vi "Text control 2 v6.0_pump-specific.vi"() -> ()   [LabVIEW 2016]
panel:
  in  "Tab Control":enum32{"Main", "Other parameters"}(tab)
  out "Line running":i32
  out "Total lines":i32
  out "Path":path=path "C:/users/rlp38/09Apr2009LTtesting/test2.txt"
  out "I vs Vg":cluster{"Y data in":dbl[], "X data in":dbl[]}[](graph)
  out "Is max":dbl format="%.2e"
  out "Id max":dbl format="%.2e"
  out "Ig max":dbl format="%.2e"
  out "Imax vs time":cluster{"Y data in":dbl[], "X data in":dbl[]}[](graph)
  out "Imin vs time":cluster{"Y data in":dbl[], "X data in":dbl[]}[](graph)
  out "I vs Vd":cluster{"Y data in":dbl[], "X data in":dbl[]}[](graph)
  in  "Script":string="#-------------------------------------------------------\n# SPM pump cleaning script\n#\n# Version 0.5\n# Author: Dimitrios Simatos\n# Last updated: 2018-01-05\n#-------------------------------------------------------\n# Description\n#\n# This script is designed to run the cleaning sequence of the SPM OEM pump.\n# This script needs to be run 4 times!\n#-------------------------------------------------------\n# Changes\n#\n# Placed initialization and hard stop commands in the beginning.\n#-------------------------------------------------------\n# Important points\n#\n# Never leave any liquid in the pump to dry after the experiments. If they dry, the residue may block the valve.\n# Always run the cleaning cycle after the experiments.\n# Use clockwise rotation when going up in valve port numbers and vice versa.\n#-------------------------------------------------------\n# Things to do before running the script\n#\n# Set time units to minutes.\n# Set filenames.\n# Replace the tubing, if necessary.\n#-------------------------------------------------------\n# Port connections\n#\n# Port 1: Waste\n# Port 2: Waste\n# Port 3: Various cleaning liquids\n# Port 4: Waste\n# Port 5: Waste\n# Port 6: Waste\n#\n# Between each of the 4 runs, the settings of Port 3 will change, according to the cleaning protocol.\n# The settings for Port 3 are:\n# 1st run: 1% v/v solution of sodium hypochlorite in ultrapure water\n# 2nd run: 0.1% w/v solution of sodium dodecyl sulfate in ultrapure water\n# 3rd run: Ultrapure water\n# 4th run: Waste (in air, not immersed in liquid)\n#-------------------------------------------------------\n# Cleaning protocol for the SPM OEM pump (from the manual)\n#\n# A cleaning procedure should be performed at the end of each day or in between two different experiments.\n# An effective cleaning can be performed in the following manner:\n# • Bleach solution to kill microorganisms\n# 1. Prepare a solution of 1% chlorine bleach and deionized water\n#    NOTE: Prepare a 1% v/v solution of sodium hypochlorite in deionized water\n# 2. Prepare a reservoir and place 1 tubing in the bleach solution and 5 tubings in a waste recipient\n# 3. Pick up the bleach solution through 1 port to entirely fill the syringe\n# 4. Sequentially output the syringe content through the remaining ports and throw it to the waste\n# 5. Repeat operation at least 2 times\n# • Detergent solution to remove debris\n# 1. Prepare a solution of 0.1% detergent and deionized water\n#    NOTE: Prepare a 0.1% w/v solution of sodium dodecyl sulfate in deionized water\n# 2. Move the tubing from the bleach solution reservoir and place it into a reservoir of detergent solution\n# 3. Pick up the detergent solution through 1 port to entirely fill the syringe\n# 4. Sequentially output the detergent solution through the remaining ports into the waste recipient\n# 5. Repeat operation at least 2 times\n# • Rinsing water to prepare the pump for your next experiment\n# 1. Move the tubing from the detergent solution reservoir and place it into a reservoir of deionized water\n# 2. Pick up the rinsing solution through 1 port to entirely fill the syringe\n# 3. Sequentially output the rinse water through the remaining ports into the waste recipient\n# 4. Repeat operation at least 2 times\n# • Replace the tubing, if necessary\n#-------------------------------------------------------\n# Pumping cycles and execution time\n#\n# Execution time for a single cycle: 6 x (1 min + 10 sec) = 7 minutes\n# Total execution time: 4 x 7 = 28 minutes\n# Since the script has to run 4 times, the cleaning lasts for: 4 x 28 = 112 minutes\n# Air must be the last to be pumped through the valve, to remove all liquids.\n# There are 4 pumping cycles. Each one draws a different liquid through port 3 and pumps it sequentially through ports 1,2,4,5,6.\n# During the sequential pumping, each port receives 200 ml of liquid (20% of the total syringe volume = 600 \"plunger units\")\n# The device must be disconnected from the port during the cleaning procedure.\n# All cycles are similar, except cycle 1 has the initialization command uncommented and the first report valve command commented.\n#-------------------------------------------------------\n# Volume of liquid needed\n#\n# Volume of liquid needed per cycle: 1 ml\n# Total volume of liquid needed per script run: 4 x 1 = 4 ml\n# Since the script has to run 4 times, the first 3 with different liquids, I need:\n# 4 ml of 1% v/v solution of sodium hypochlorite in ultrapure water\n# 4 ml of 0.1% w/v solution of sodium dodecyl sulfate in ultrapure water\n# 4 ml of ultrapure water\n#-------------------------------------------------------\n# Parameters\n#\n# Syringe size: 1 ml\n# Step resolution N = 0.01 mm\n# Drawing flow V = 300 pulses/second (6000 ul/min)\n# Pumping flow V = 300 pulses/second (6000 ul/min)\n#-------------------------------------------------------\n# Pump initialization\npump /1T #hard stop pump\npump /1ZR #initialize pump\n#-------------------------------------------------------\n# Cycle 1\n# Fill the syringe\npump /1Q #query pump\npump /1? #report absolute plunger position\n#pump /1?6 #report valve position\nwait-min 1 #wait 1 minute\npump /1N0R #set step resolution: 0.01 mm\npump /1Q #query pump\npump /1? #report absolute plunger position (the plunger should be at 0)\npump /1?6 #report valve position\nwait 1000 #wait 1 second\npump /1V300R #choose speed: 300 steps/s (6000 ul/min)\npump /1Q #query pump\nwait 1000 #wait 1 second\npump /1I3R #go to port 3, clockwise rotation\npump /1Q #query pump\npump /1?6 #report valve position\nwait 1000 #wait 1 second\npump /1A3000R #go to absolute position 3000 (= draw 1 ml)\nwait 30000 #wait 30 seconds\npump /1Q #query pump\npump /1? #report absolute plunger position (the plunger should have finished moving)\n#pump /1?6 #report valve position\n# The sequential pumping begins\n# Port 1\npump /1O1R #switch to port 1, counterclockwise rotation\npump /1Q #query pump\npump /1?6 #report valve position\npump /1A2400R #go to absolute position 2400 (= pump 200 ul)\npump /1Q #query pump\npump /1? #report absolute plunger position (the plunger should be moving to 0)\nwait-min 1 #wait 1 minute\npump /1? #report absolute plunger position (the plunger should have finished moving)\n# Port 2\npump /1I2R #switch to port 2, clockwise rotation\npump /1Q #query pump\npump /1?6 #report valve position\npump /1A1800R #go to absolute position 1800 (= pump 200 ul)\npump /1Q #query pump\npump /1? #report absolute plunger position (the plunger should be moving to 0)\nwait-min 1 #wait 1 minute\npump /1? #report absolute plunger position (the plunger should have finished moving)\n# Port 4\npump /1I4R #switch to port 4, clockwise rotation\npump /1Q #query pump\npump /1?6 #report valve position\npump /1A1200R #go to absolute position 1200 (= pump 200 ul)\npump /1Q #query pump\npump /1? #report absolute plunger position (the plunger should be moving to 0)\nwait-min 1 #wait 1 minute\npump /1? #report absolute plunger position (the plunger should have finished moving)\n# Port 5\npump /1I5R #switch to port 5, clockwise rotation\npump /1Q #query pump\npump /1?6 #report valve position\npump /1A600R #go to absolute position 600 (= pump 200 ul)\npump /1Q #query pump\npump /1? #report absolute plunger position (the plunger should be moving to 0)\nwait-min 1 #wait 1 minute\npump /1? #report absolute plunger position (the plunger should have finished moving)\n# Port 6\npump /1I6R #switch to port 6, clockwise rotation\npump /1Q #query pump\npump /1?6 #report valve position\npump /1A0R #go to absolute position 0 (= pump 200 ul)\npump /1Q #query pump\npump /1? #report absolute plunger position (the plunger should be moving to 0)\nwait-min 1 #wait 1 minute\npump /1? #report absolute plunger position (the plunger should have finished moving)\n#-------------------------------------------------------\n# Cycle 2\n# Fill the syringe\n#pump /1ZR #initialize pump\npump /1Q #query pump\npump /1? #report absolute plunger position\npump /1?6 #report valve position\nwait-min 1 #wait 1 minute\npump /1N0R #set step resolution: 0.01 mm\npump /1Q #query pump\npump /1? #report absolute plunger position (the plunger should be at 0)\npump /1?6 #report valve position\nwait 1000 #wait 1 second\npump /1V300R #choose speed: 300 steps/s (6000 ul/min)\npump /1Q #query pump\nwait 1000 #wait 1 second\npump /1O3R #go to port 3, counterclockwise rotation\npump /1Q #query pump\npump /1?6 #report valve position\nwait 1000 #wait 1 second\npump /1A3000R #go to absolute position 3000 (= draw 1 ml)\nwait 30000 #wait 30 seconds\npump /1Q #query pump\npump /1? #report absolute plunger position (the plunger should have finished moving)\n#pump /1?6 #report valve position\n# The sequential pumping begins\n# Port 1\npump /1O1R #switch to port 1, counterclockwise rotation\npump /1Q #query pump\npump /1?6 #report valve position\npump /1A2400R #go to absolute position 2400 (= pump 200 ul)\npump /1Q #query pump\npump /1? #report absolute plunger position (the plunger should be moving to 0)\nwait-min 1 #wait 1 minute\npump /1? #report absolute plunger position (the plunger should have finished moving)\n# Port 2\npump /1I2R #switch to port 2, clockwise rotation\npump /1Q #query pump\npump /1?6 #report valve position\npump /1A1800R #go to absolute position 1800 (= pump 200 ul)\npump /1Q #query pump\npump /1? #report absolute plunger position (the plunger should be moving to 0)\nwait-min 1 #wait 1 minute\npump /1? #report absolute plunger position (the plunger should have finished moving)\n# Port 4\npump /1I4R #switch to port 4, clockwise rotation\npump /1Q #query pump\npump /1?6 #report valve position\npump /1A1200R #go to absolute position 1200 (= pump 200 ul)\npump /1Q #query pump\npump /1? #report absolute plunger position (the plunger should be moving to 0)\nwait-min 1 #wait 1 minute\npump /1? #report absolute plunger position (the plunger should have finished moving)\n# Port 5\npump /1I5R #switch to port 5, clockwise rotation\npump /1Q #query pump\npump /1?6 #report valve position\npump /1A600R #go to absolute position 600 (= pump 200 ul)\npump /1Q #query pump\npump /1? #report absolute plunger position (the plunger should be moving to 0)\nwait-min 1 #wait 1 minute\npump /1? #report absolute plunger position (the plunger should have finished moving)\n# Port 6\npump /1I6R #switch to port 6, clockwise rotation\npump /1Q #query pump\npump /1?6 #report valve position\npump /1A0R #go to absolute position 0 (= pump 200 ul)\npump /1Q #query pump\npump /1? #report absolute plunger position (the plunger should be moving to 0)\nwait-min 1 #wait 1 minute\npump /1? #report absolute plunger position (the plunger should have finished moving)\n#-------------------------------------------------------\n# Cycle 3\n# Fill the syringe\n#pump /1ZR #initialize pump\npump /1Q #query pump\npump /1? #report absolute plunger position\npump /1?6 #report valve position\nwait-min 1 #wait 1 minute\npump /1N0R #set step resolution: 0.01 mm\npump /1Q #query pump\npump /1? #report absolute plunger position (the plunger should be at 0)\npump /1?6 #report valve position\nwait 1000 #wait 1 second\npump /1V300R #choose speed: 300 steps/s (6000 ul/min)\npump /1Q #query pump\nwait 1000 #wait 1 second\npump /1O3R #go to port 3, counterclockwise rotation\npump /1Q #query pump\npump /1?6 #report valve position\nwait 1000 #wait 1 second\npump /1A3000R #go to absolute position 3000 (= draw 1 ml)\nwait 30000 #wait 30 seconds\npump /1Q #query pump\npump /1? #report absolute plunger position (the plunger should have finished moving)\n#pump /1?6 #report valve position\n# The sequential pumping begins\n# Port 1\npump /1O1R #switch to port 1, counterclockwise rotation\npump /1Q #query pump\npump /1?6 #report valve position\npump /1A2400R #go to absolute position 2400 (= pump 200 ul)\npump /1Q #query pump\npump /1? #report absolute plunger position (the plunger should be moving to 0)\nwait-min 1 #wait 1 minute\npump /1? #report absolute plunger position (the plunger should have finished moving)\n# Port 2\npump /1I2R #switch to port 2, clockwise rotation\npump /1Q #query pump\npump /1?6 #report valve position\npump /1A1800R #go to absolute position 1800 (= pump 200 ul)\npump /1Q #query pump\npump /1? #report absolute plunger position (the plunger should be moving to 0)\nwait-min 1 #wait 1 minute\npump /1? #report absolute plunger position (the plunger should have finished moving)\n# Port 4\npump /1I4R #switch to port 4, clockwise rotation\npump /1Q #query pump\npump /1?6 #report valve position\npump /1A1200R #go to absolute position 1200 (= pump 200 ul)\npump /1Q #query pump\npump /1? #report absolute plunger position (the plunger should be moving to 0)\nwait-min 1 #wait 1 minute\npump /1? #report absolute plunger position (the plunger should have finished moving)\n# Port 5\npump /1I5R #switch to port 5, clockwise rotation\npump /1Q #query pump\npump /1?6 #report valve position\npump /1A600R #go to absolute position 600 (= pump 200 ul)\npump /1Q #query pump\npump /1? #report absolute plunger position (the plunger should be moving to 0)\nwait-min 1 #wait 1 minute\npump /1? #report absolute plunger position (the plunger should have finished moving)\n# Port 6\npump /1I6R #switch to port 6, clockwise rotation\npump /1Q #query pump\npump /1?6 #report valve position\npump /1A0R #go to absolute position 0 (= pump 200 ul)\npump /1Q #query pump\npump /1? #report absolute plunger position (the plunger should be moving to 0)\nwait-min 1 #wait 1 minute\npump /1? #report absolute plunger position (the plunger should have finished moving)\n#-------------------------------------------------------\n# Cycle 4\n# Fill the syringe\n#pump /1ZR #initialize pump\npump /1Q #query pump\npump /1? #report absolute plunger position\npump /1?6 #report valve position\nwait-min 1 #wait 1 minute\npump /1N0R #set step resolution: 0.01 mm\npump /1Q #query pump\npump /1? #report absolute plunger position (the plunger should be at 0)\npump /1?6 #report valve position\nwait 1000 #wait 1 second\npump /1V300R #choose speed: 300 steps/s (6000 ul/min)\npump /1Q #query pump\nwait 1000 #wait 1 second\npump /1O3R #go to port 3, counterclockwise rotation\npump /1Q #query pump\npump /1?6 #report valve position\nwait 1000 #wait 1 second\npump /1A3000R #go to absolute position 3000 (= draw 1 ml)\nwait 30000 #wait 30 seconds\npump /1Q #query pump\npump /1? #report absolute plunger position (the plunger should have finished moving)\n#pump /1?6 #report valve position\n# The sequential pumping begins\n# Port 1\npump /1O1R #switch to port 1, counterclockwise rotation\npump /1Q #query pump\npump /1?6 #report valve position\npump /1A2400R #go to absolute position 2400 (= pump 200 ul)\npump /1Q #query pump\npump /1? #report absolute plunger position (the plunger should be moving to 0)\nwait-min 1 #wait 1 minute\npump /1? #report absolute plunger position (the plunger should have finished moving)\n# Port 2\npump /1I2R #switch to port 2, clockwise rotation\npump /1Q #query pump\npump /1?6 #report valve position\npump /1A1800R #go to absolute position 1800 (= pump 200 ul)\npump /1Q #query pump\npump /1? #report absolute plunger position (the plunger should be moving to 0)\nwait-min 1 #wait 1 minute\npump /1? #report absolute plunger position (the plunger should have finished moving)\n# Port 4\npump /1I4R #switch to port 4, clockwise rotation\npump /1Q #query pump\npump /1?6 #report valve position\npump /1A1200R #go to absolute position 1200 (= pump 200 ul)\npump /1Q #query pump\npump /1? #report absolute plunger position (the plunger should be moving to 0)\nwait-min 1 #wait 1 minute\npump /1? #report absolute plunger position (the plunger should have finished moving)\n# Port 5\npump /1I5R #switch to port 5, clockwise rotation\npump /1Q #query pump\npump /1?6 #report valve position\npump /1A600R #go to absolute position 600 (= pump 200 ul)\npump /1Q #query pump\npump /1? #report absolute plunger position (the plunger should be moving to 0)\nwait-min 1 #wait 1 minute\npump /1? #report absolute plunger position (the plunger should have finished moving)\n# Port 6\npump /1I6R #switch to port 6, clockwise rotation\npump /1Q #query pump\npump /1?6 #report valve position\npump /1A0R #go to absolute position 0 (= pump 200 ul)\npump /1Q #query pump\npump /1? #report absolute plunger position (the plunger should be moving to 0)\nwait-min 1 #wait 1 minute\npump /1? #report absolute plunger position (the plunger should have finished moving)\n#-------------------------------------------------------"
  out "Command running:":string
  out "Serial port data":string
  out "Elapsed Time":dbl caption="Elapsed Time (s)"
  in  "Units (label only)":u16(ring)=1 items=["Seconds", "Minutes", "Hours"]
  in  "Time Offset":dbl caption="Set Start Time (s)"
  in  "Reset":bool
  in  "Auto Reset":bool
  in  "integration time":u32(slide) max=2 step=1 scale=0.0..2.0
  in  "Interrupt run":bool
  out "Absolute plunger position vs time":cluster{"Y data in":dbl[], "X data in":dbl[]}[](graph)
  out "Valve position vs time":cluster{"Y data in":dbl[], "X data in":dbl[]}[](graph)
  out "Is on":dbl format="%.2e"
  out "Id on":dbl format="%.2e"
  out "Ig on":dbl format="%.2e"
  out "Ion vs time":cluster{"Y data in":dbl[], "X data in":dbl[]}[](graph)
  out "Ioff vs time":cluster{"Y data in":dbl[], "X data in":dbl[]}[](graph)
  out "Ig min":dbl format="%.2e"
  out "Id min":dbl format="%.2e"
  out "Is min":dbl format="%.2e"
  out "Is off":dbl format="%.2e"
  out "Id off":dbl format="%.2e"
  out "Ig off":dbl format="%.2e"
  in  "Integration time (long)":dbl=0.32 min=0.04 max=2.0 step=0.02 format="%.2f"
  in  "Integration time (short)":dbl=0.0019 min=8e-05 max=0.0019 step=8e-05 format="%^.0e"
  in  "Gate: Compliance":dbl=0.001 format="%.8f"
  in  "Drain: Compliance":dbl=0.001 format="%.8f"
  in  "Hard stop pump":bool
  in  "Halt pump":bool
  in  "Gate Range\nmode":u16(ring) items=["Auto", "Limited", "Fixed"]
  in  "Gate Range":u8(slide)=6 max=11 scale=0.0..11.0
  in  "Source/Drain\nRange mode":u16(ring) items=["Auto", "Limited", "Fixed"]
  in  "Source/Drain Range":u8(slide)=6 max=11 scale=0.0..11.0
  in  "Panel Controls":T1={"Emergency Stop"=refnum, "TransGraph Max"=1e-05, "Text/Graph (text=false)"=TRUE} {"TransGraph Max" format="%.2e"}
  in  "Panel Controls 2":T2={"Emergency Stop"=refnum, "TransGraph Max"=1e-05, "Text/Graph (text=false)"=TRUE, "TransGraph Min"=1e-11} {"TransGraph Min" format="%.2e"; "TransGraph Max" format="%.2e"}
  in  "SMU4":cluster{"on/off":bool, "Voltage":dbl} {"Voltage" min=-100.0 max=100.0 format="%.2f"}
  in  "Full Reset":bool
  in  "Standby":T3
  out "error out":errorcluster
  in  "Delay before read (ms)":u32=1000
  in  "byte count":u32=64
  in  "Serial End Mode for Reads":u16(ring)=2 items=["None", "LastBit", "TermChar"]
  in  "Timeout (ms)":u32=10000
  in  "Enable Termination\nChar (T)":bool=TRUE
  in  "Termination char\n(0xA = '\\n' = LF)\n(0xD = '\\r' = CR)":u8=13 format="%.0x"
  in  "flow control":u16(ring) items=["None"=0, "XON/XOFF"=1, "RTS/CTS"=2, "DTR/DSR"=4]
  in  "stop bits":u16(ring)=10 items=["1.0"=10, "1.5"=15, "2.0"=20]
  in  "parity":u16(ring) items=["None", "Odd", "Even", "Mark", "Space"]
  in  "data bits":u16=8 min=5 max=8 step=1
  in  "VISA resource name":refnum<visa-resource-name>="COM6"
  in  "baud rate":u32=9600
  in  "Filename (variable part)":string="step_1_up-H2O_initial_"
  in  "Suffix (script)":string="step_1_up-H2O_initial_script.txt"
  out "Timings Indicator":T4
  in  "Timings (overwritten by the Front Panel)":T5={"integration time"=0, "Short/Long integration time"=0.00064, "hold time (sec)"=0.0, "delay time (sec)"=0.0, "Step Time (0 disables)"=0.0, "sweep method"=0, "Pulse period"=0.005, "Base voltage"=0.0, "Pulse width"=0.0005} {"Pulse width" min=0.0005 max=0.1 step=0.0001 format="%.4f"; "Base voltage" format="%^.4e"; "Pulse period" min=0.005 max=1.0 step=0.0001 format="%.4f"; "sweep method" items=["Continuous", "Pulsed"]; "Step Time (0 disables)" format="%.2f"; "delay time (sec)" format="%.4f"; "hold time (sec)" format="%.4f"; "Short/Long integration time" format="%^.0e"; "integration time" scale=0.0..2.0}
  in  "Gate":T6={"Gate Start"=0.0, "Gate Stop"=2.0, "Gate Step (linear only)"=1.0, "Gate Compliance"=0.0001, "Gate PComp"=0.0, "Range mode"=0, "Range"=6} {"Range" max=11 scale=0.0..11.0; "Range mode" items=["Auto", "Limited", "Fixed"]; "Gate PComp" format="%^.2e"; "Gate Compliance" format="%^.2e"; "Gate Step (linear only)" format="%^.4e"; "Gate Stop" format="%^.4e"; "Gate Start" format="%^.4e"}
  in  "Drain 2":T7={"Drain Start"=0.0, "Drain Stop"=2.0, "Drain Compliance"=0.0001, "Drain Step"=1.0, "Drain PComp"=0.0, "Range mode"=0, "Range"=6} {"Range" max=11 scale=0.0..11.0; "Range mode" items=["Auto", "Limited", "Fixed"]; "Drain PComp" format="%^.2e"; "Drain Step" format="%^.4e"; "Drain Compliance" format="%^.2e"; "Drain Stop" format="%^.4e"; "Drain Start" format="%^.4e"}
  # "Syntax:\nitime [s|m|l] time(sec): [s|m|l] determines the integration time setting (small|medium|long) and time sets the value.\nNOTE: The value of the integration time has to be within the range allowed by its category (s|m|l), otherwise, the closest value will be used. (e.g. if the category is set to short but the time value is very long, the actual value used will be the maximum short integration time.\nIntegration times:\n    Short: Default: 640 us. Range: 8E-5 - 1.92E-3 seconds.\n    Medium: Fixed at 1 NPL cycle (0.02 seconds).\n    Long: Default: 16 NPL cycles (0.32 seconds). Range: 2-100 NPL cycles (0.04 seconds - 2 seconds).\ngaterangemode [a|l|f]\ndrainrangemode [a|l|f]\npulsed [on|off] PulsePeriod(sec) PulseBaseVoltage PulseONWidth(sec)\nstandby [on l off]\nwait NumMilliseconds\nwait-min NumMinutes\n# texthere = comment\ntransfer [s|d] VgStart VgStop VgStep VdStart VdStop VdStep\noutput [s|d] VgStart VgStop VgStep VdStart VdStop VdStep\nsample Vg Vd NumSamples Time(s) SampleInterval(s)\nsamplei Idg NumSamples Time(s) SampleInterval(s) VDGcompliance\n100 samples is approximately 13 seconds with medium integration\n# if in doubt use SampleInterval(s) = 0.004\nstressV VG VD IGcompliance IDcompliance Duration(sec)\nstressI IDG VDGcompliance Duration(sec)\nvsu2pulse Bias Duration(s)\npulsedstressV [s|d] VEstop VgON VgOFF Period(s) PulseONwidth(s) Vd\nsample-fpp Vg Vd NumSamples Time\nresample-fpp Vg Vd\ntransfer-fpp [s|d] VgStart VgStop VgStep VdStart VdStop VdStep\noutput-fpp [s|d] VgStart VgStop VgStep VdStart VdStop VdStep\nserial SerialPortCommand\npump SerialPortCommand for the SPM pump\n\nSPM Pump Syntax (<x>: pump number, use 1 if only one pump):\nif the command syntax contains [R], then append the letter R to the command\n/<x>Q: query (a query command should follow each command)\n/<x>Z[R] or /<x>Y[R]: initialize pump\n/<x>N<n>[R] (<n>=0,1): <0> (<1>) microstep 0.01 mm (0.00125 mm) resolution\n/<x>I<n> (<n>=0-6): turn to port number n (clockwise)\n/<x>O<n> (<n>=0-6): turn to port number n (counterclockwise)\n/<x>X: Re-execute last command string\n/<x>G<n>[R] (<n>=0-60000): repeat command sequence (default: 0, 0=loop forever)\n/<x>g: Mark the start of a repeat sequence (max = 10)\n/<x>M<n>[R] (<n>=0-86400000): delay command execution by n milliseconds\n/<x>H: Halt; Pause the sequence after finishing the current move\n/<x>T: Hardstop; Interrupt the current move and suppress it from the sequence\n/<x>A<n>[R] (<n>=0-3000 with N=0, 0-24000 with N=1): absolute position\n/<x>P<n>[R] (<n>=0-3000 with N=0, 0-24000 with N=1): relative pickup\n/<x>D<n>[R] (<n>=0-3000 with N=0, 0-24000 with N=1): relative dispense\n/<x>V<n>[R] (<n>=1-1600 default: 150): set peak speed (pulses/sec)\nNOTE: The lowest speed limit is 1 pulse/sec, not 5, as the manual states.\n/<x>S<n>[R] (<n>=10-40 default: 22): set speed (NOT in pulses/sec, look in manual)\nNOTE: When controlled with absolute position, one does not need to pay special attention to the syringe that is mounted on the pump.\nWithdraw from lower stage (ports 3, 5), dispense from higher stage (ports 2, 4, 6).\nConnect Port 1 to waste."
  # "Time"
  # "1\n2\n3\n4\n5\n6\n7\n8\n9\n10\n11\n12\n13\n14\n15\n16\n17\n18\n19\n20"
  # "Serial port settings"
  # "Filename settings"
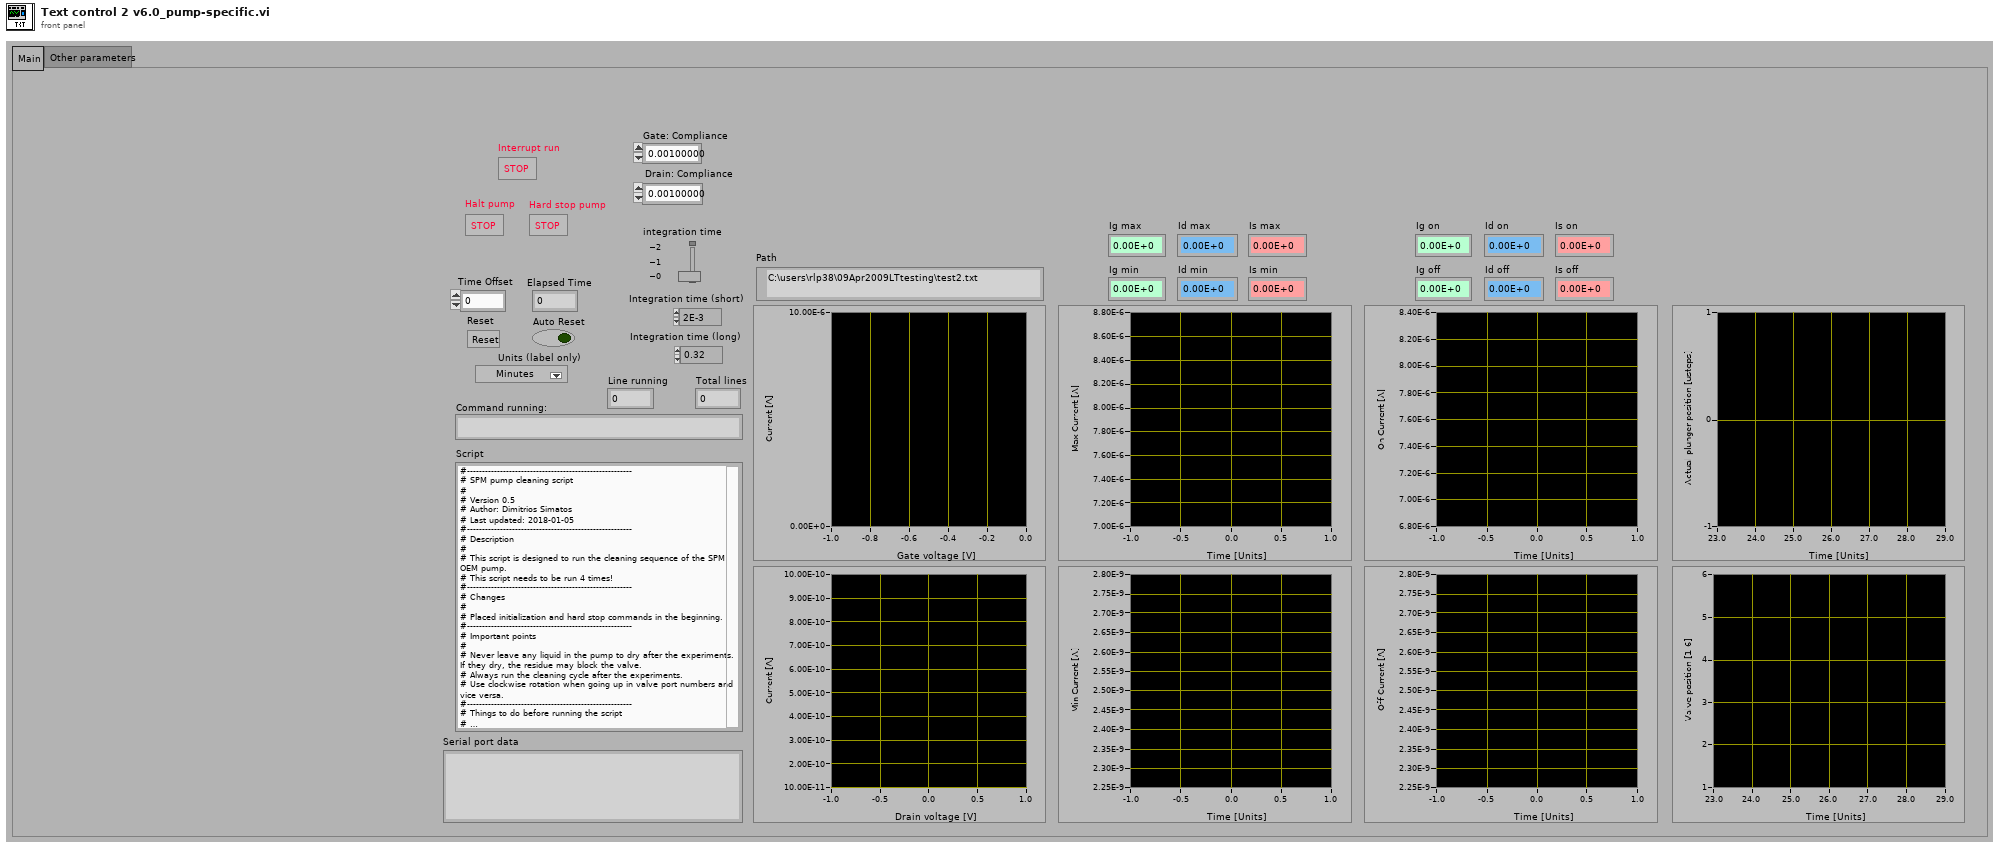
[diagram p1: front panel]
types:
  T1 = cluster{"Emergency Stop":refnum<vi>, "TransGraph Max":dbl, "Text/Graph (text=false)":bool}
  T2 = cluster{"Emergency Stop":refnum<vi>, "TransGraph Max":dbl, "Text/Graph (text=false)":bool, "TransGraph Min":dbl}
  T3 = cluster{"Gate Standby":bool, "Drain Standby":bool}
  T4 = cluster{"integration time (0:s, 1:m, 2:l)":u32, "Short/Long integration time":dbl, "hold time (sec)":dbl, "delay time (sec)":dbl, "Step Time (0 disables)":dbl, "sweep method":u16, "Pulse period":dbl, "Base voltage":dbl, "Pulse width":dbl}
  T5 = cluster{"integration time":u32, "Short/Long integration time":dbl, "hold time (sec)":dbl, "delay time (sec)":dbl, "Step Time (0 disables)":dbl, "sweep method":u16, "Pulse period":dbl, "Base voltage":dbl, "Pulse width":dbl}
  T6 = cluster{"Gate Start":dbl, "Gate Stop":dbl, "Gate Step (linear only)":dbl, "Gate Compliance":dbl, "Gate PComp":dbl, "Range mode":u16, "Range":u8}
  T7 = cluster{"Drain Start":dbl, "Drain Stop":dbl, "Drain Compliance":dbl, "Drain Step":dbl, "Drain PComp":dbl, "Range mode":u16, "Range":u8}
  T8 = enum16{"open", "replace", "create", "open or create", "replace or create", "replace or create with confirmation"}
  T9 = cluster{"V2 Start":dbl, "V2 Step":dbl, "Number of points":i32}
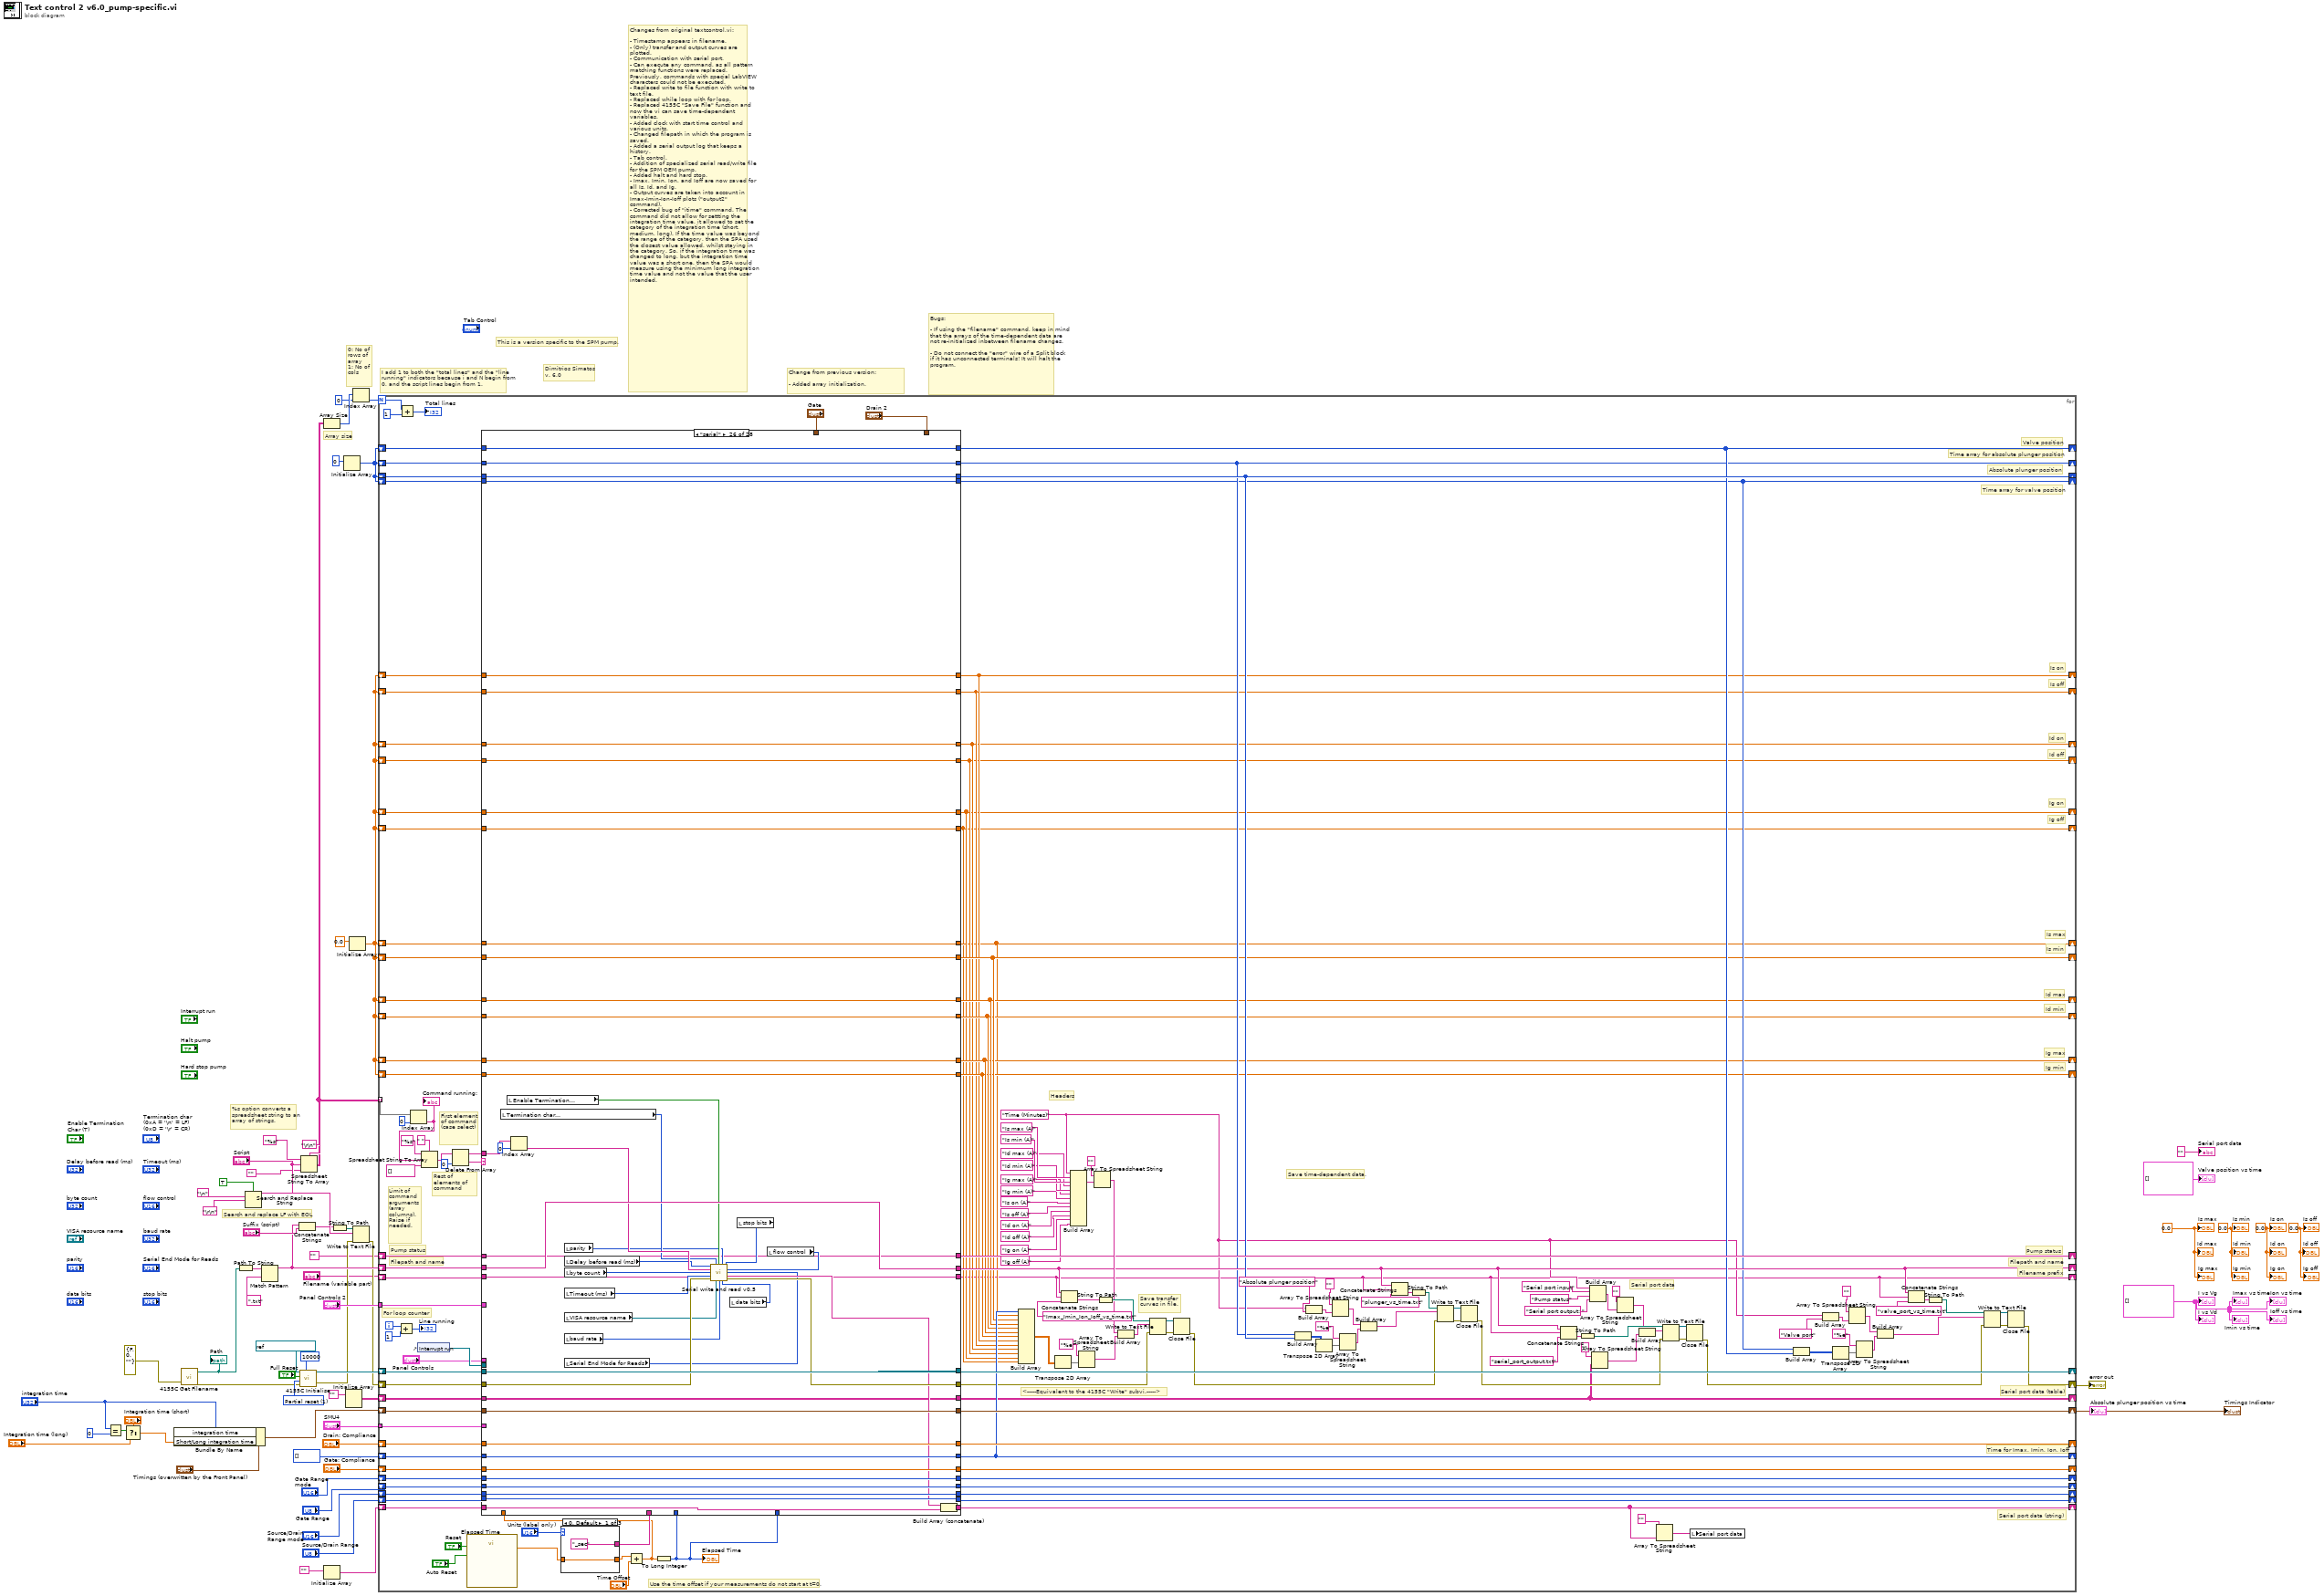
[diagram p0: block diagram]
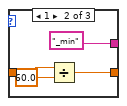
[diagram p2: hidden frame]
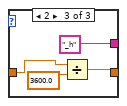
[diagram p3: hidden frame]
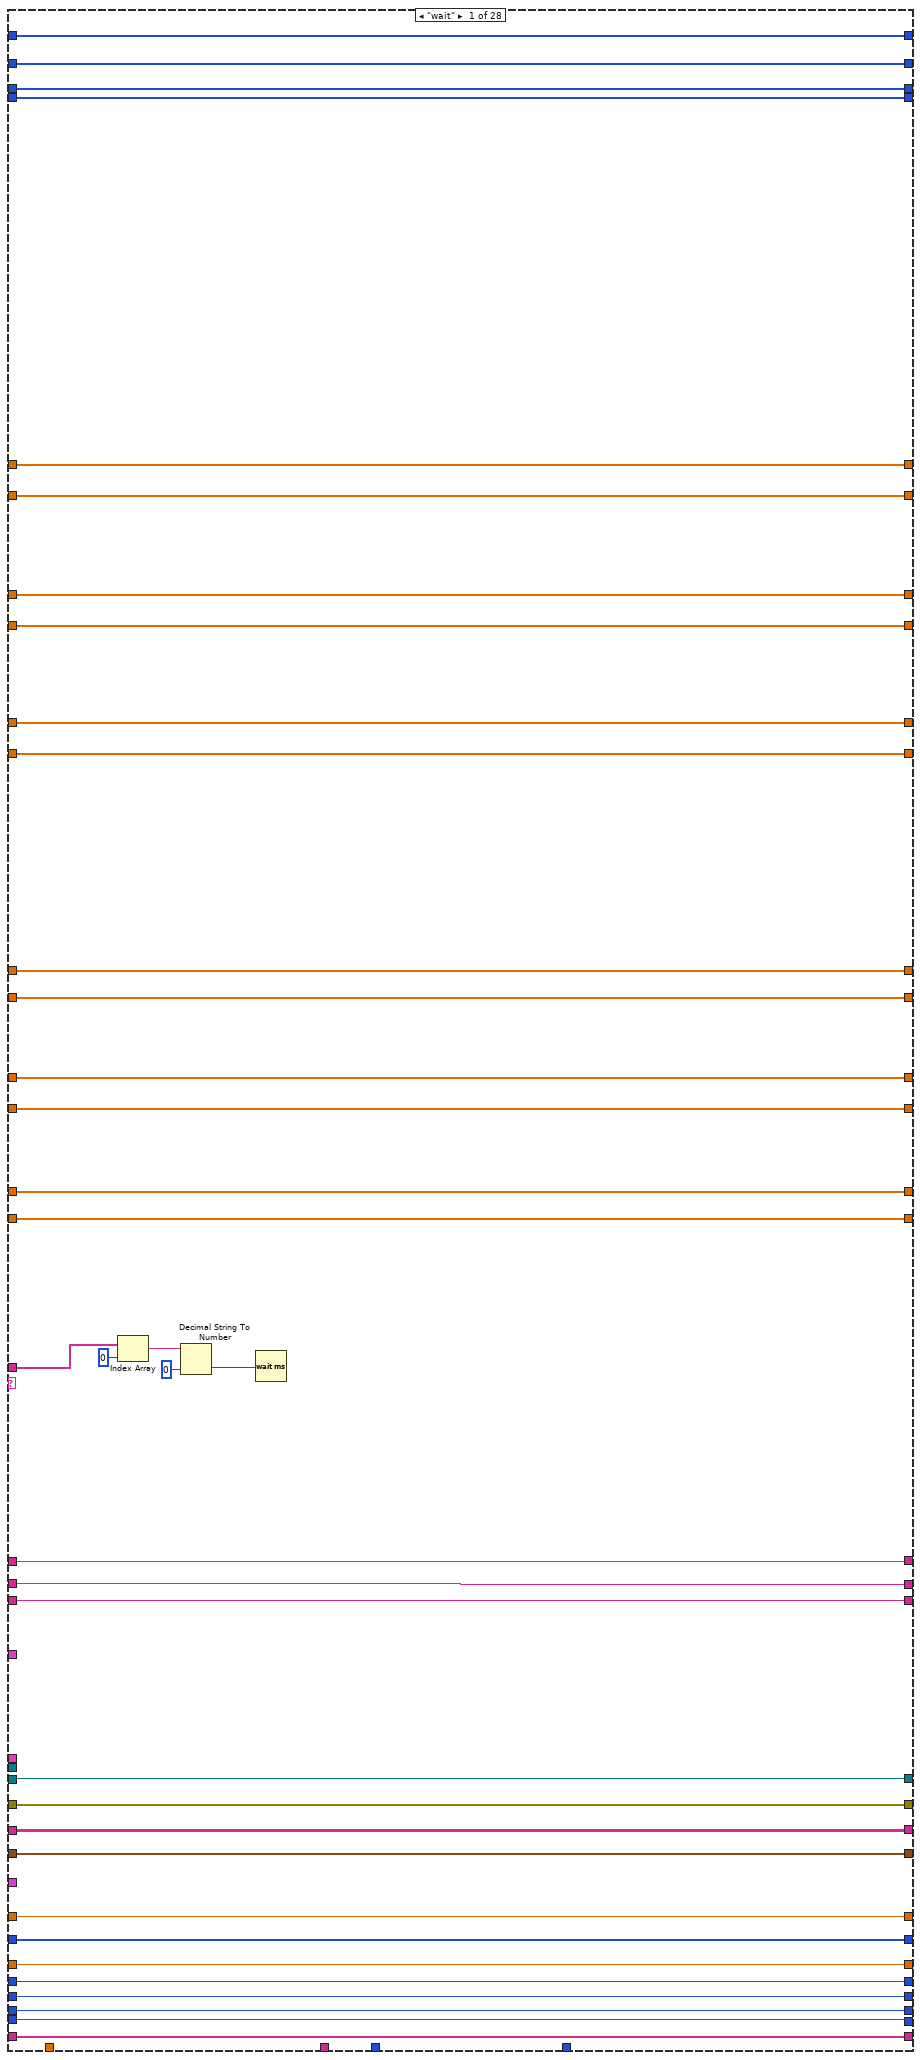
[diagram p4: hidden frame]
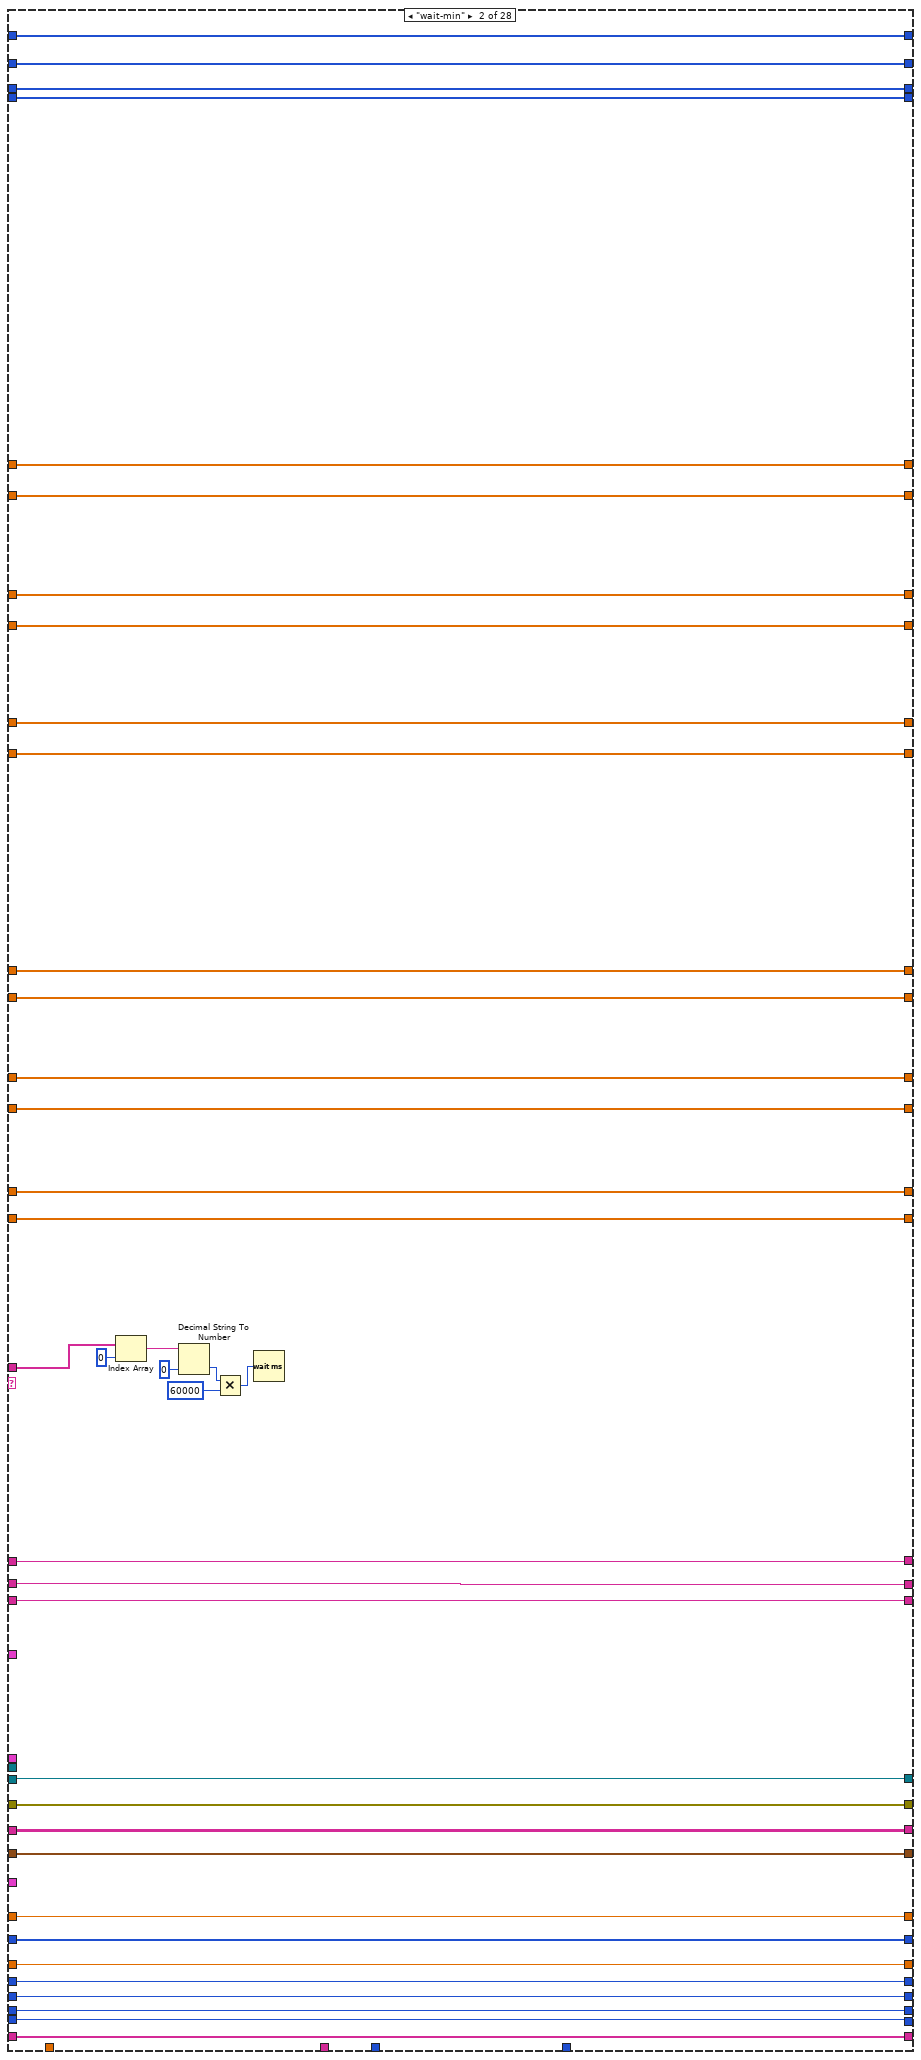
[diagram p5: hidden frame]
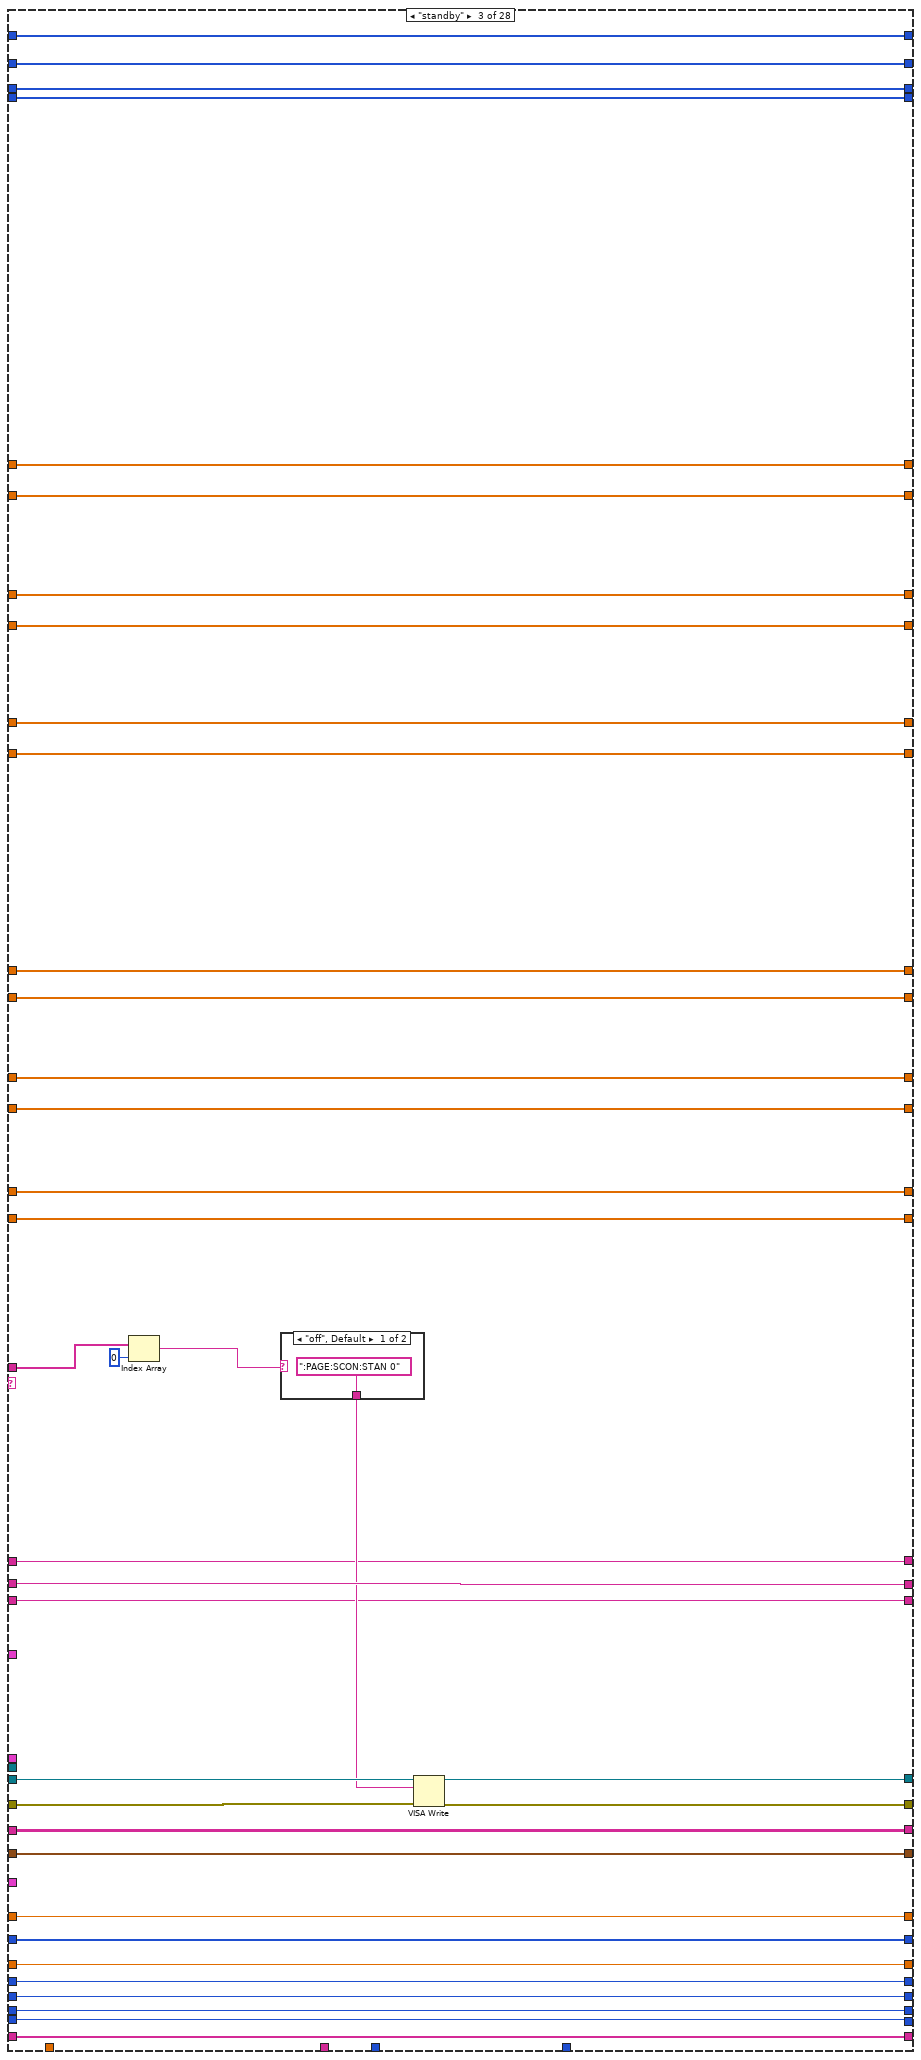
[diagram p6: hidden frame]
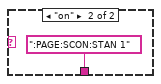
[diagram p7: hidden frame]
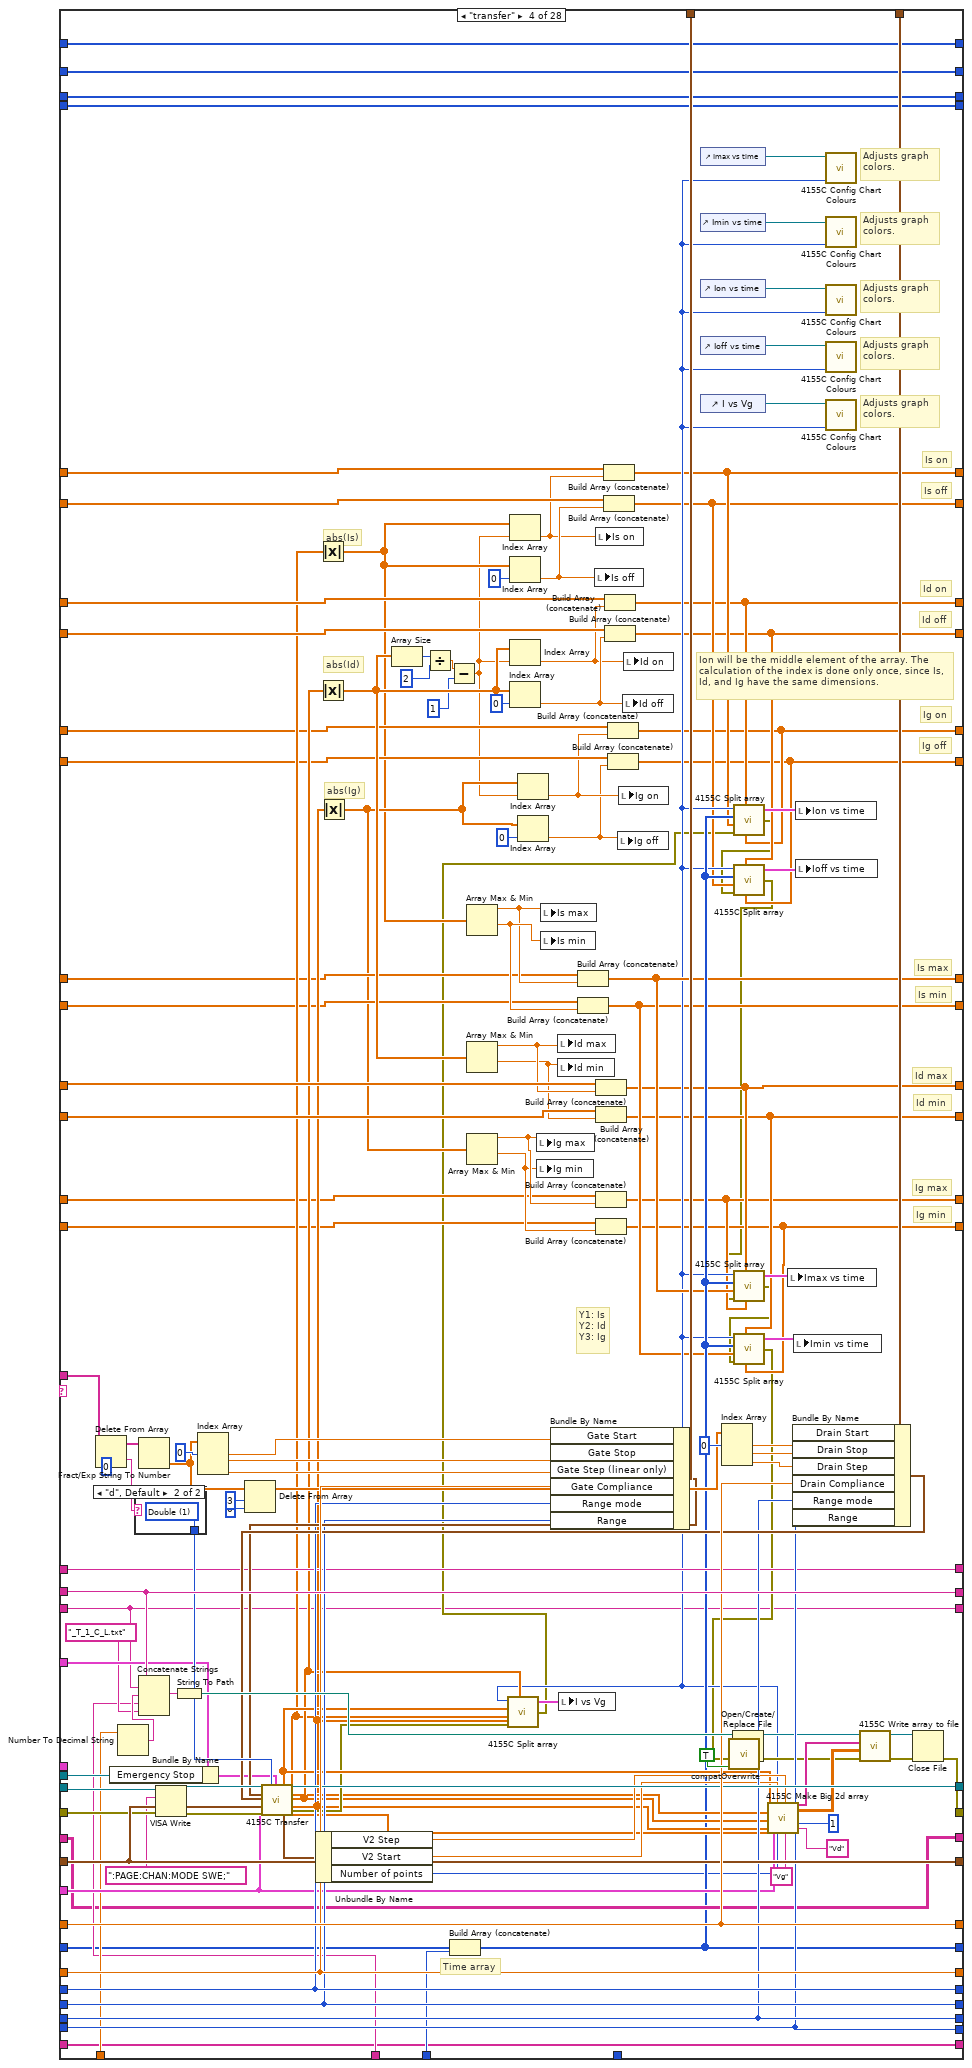
[diagram p8: hidden frame]
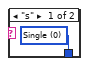
[diagram p9: hidden frame]
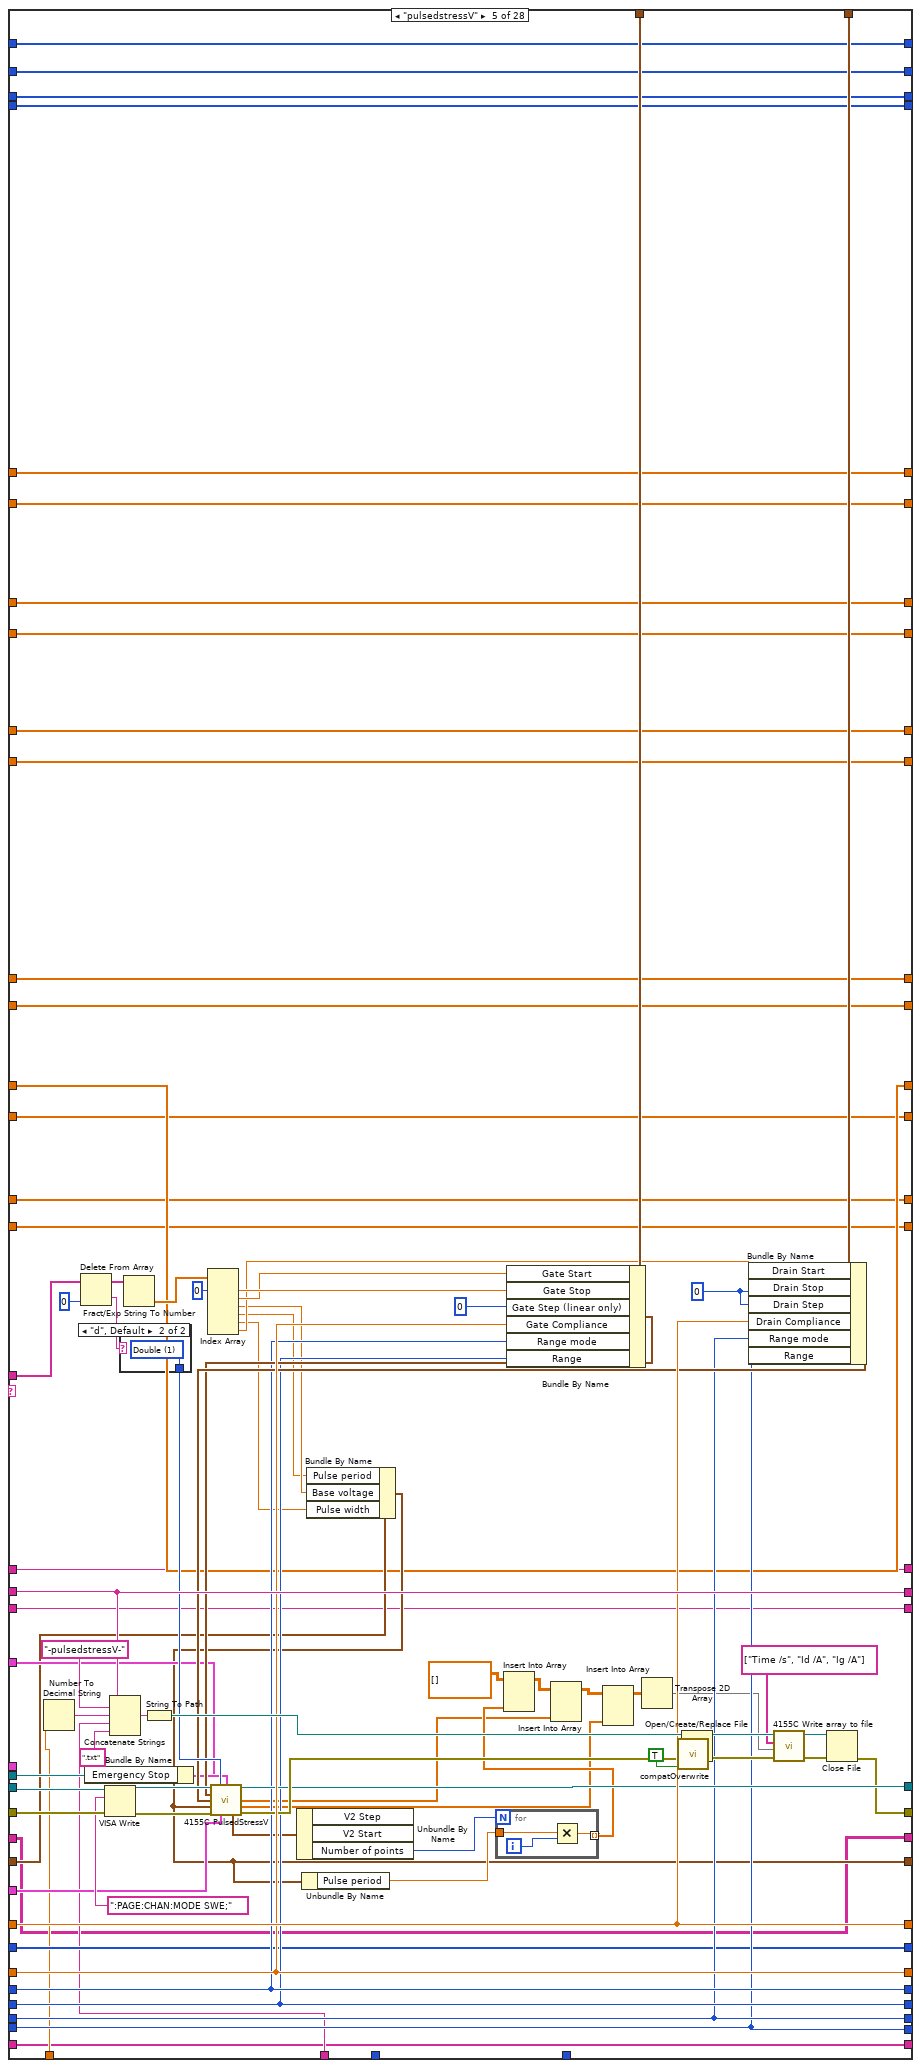
[diagram p10: hidden frame]
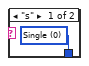
[diagram p11: hidden frame]
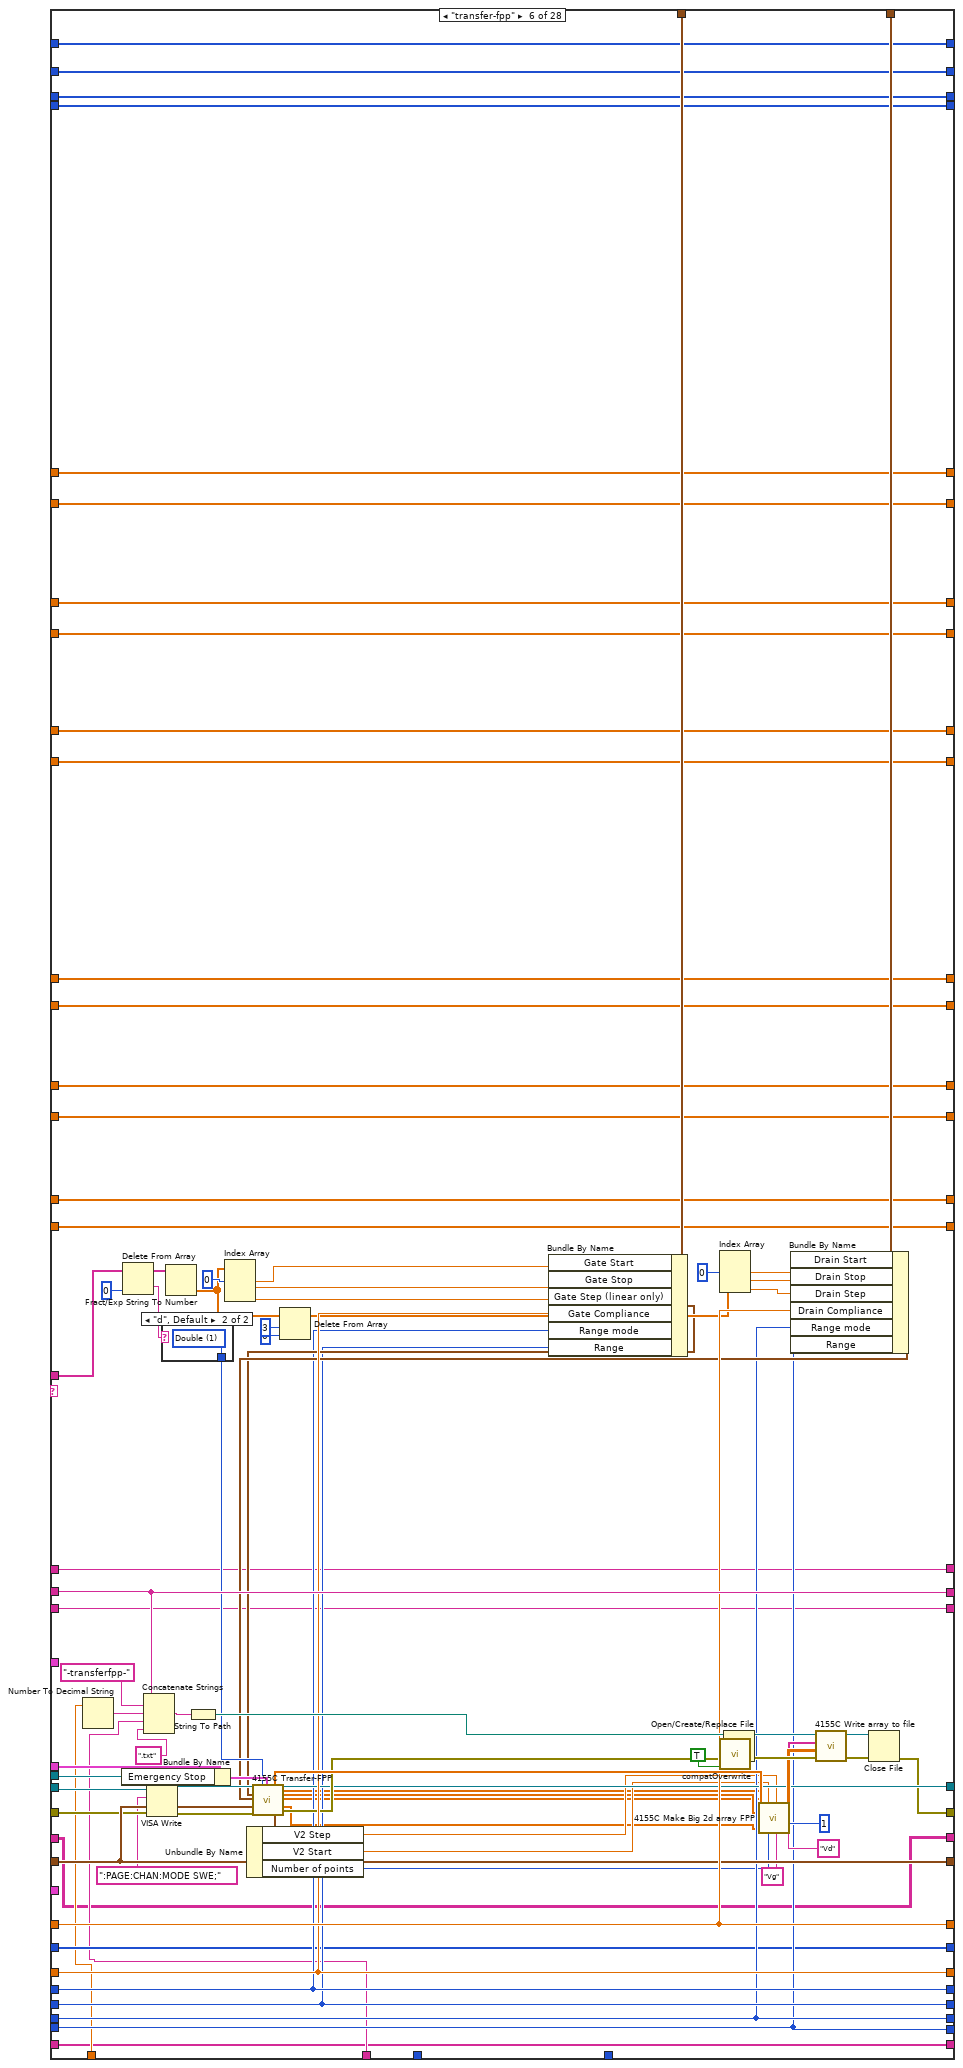
[diagram p12: hidden frame]
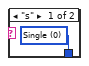
[diagram p13: hidden frame]
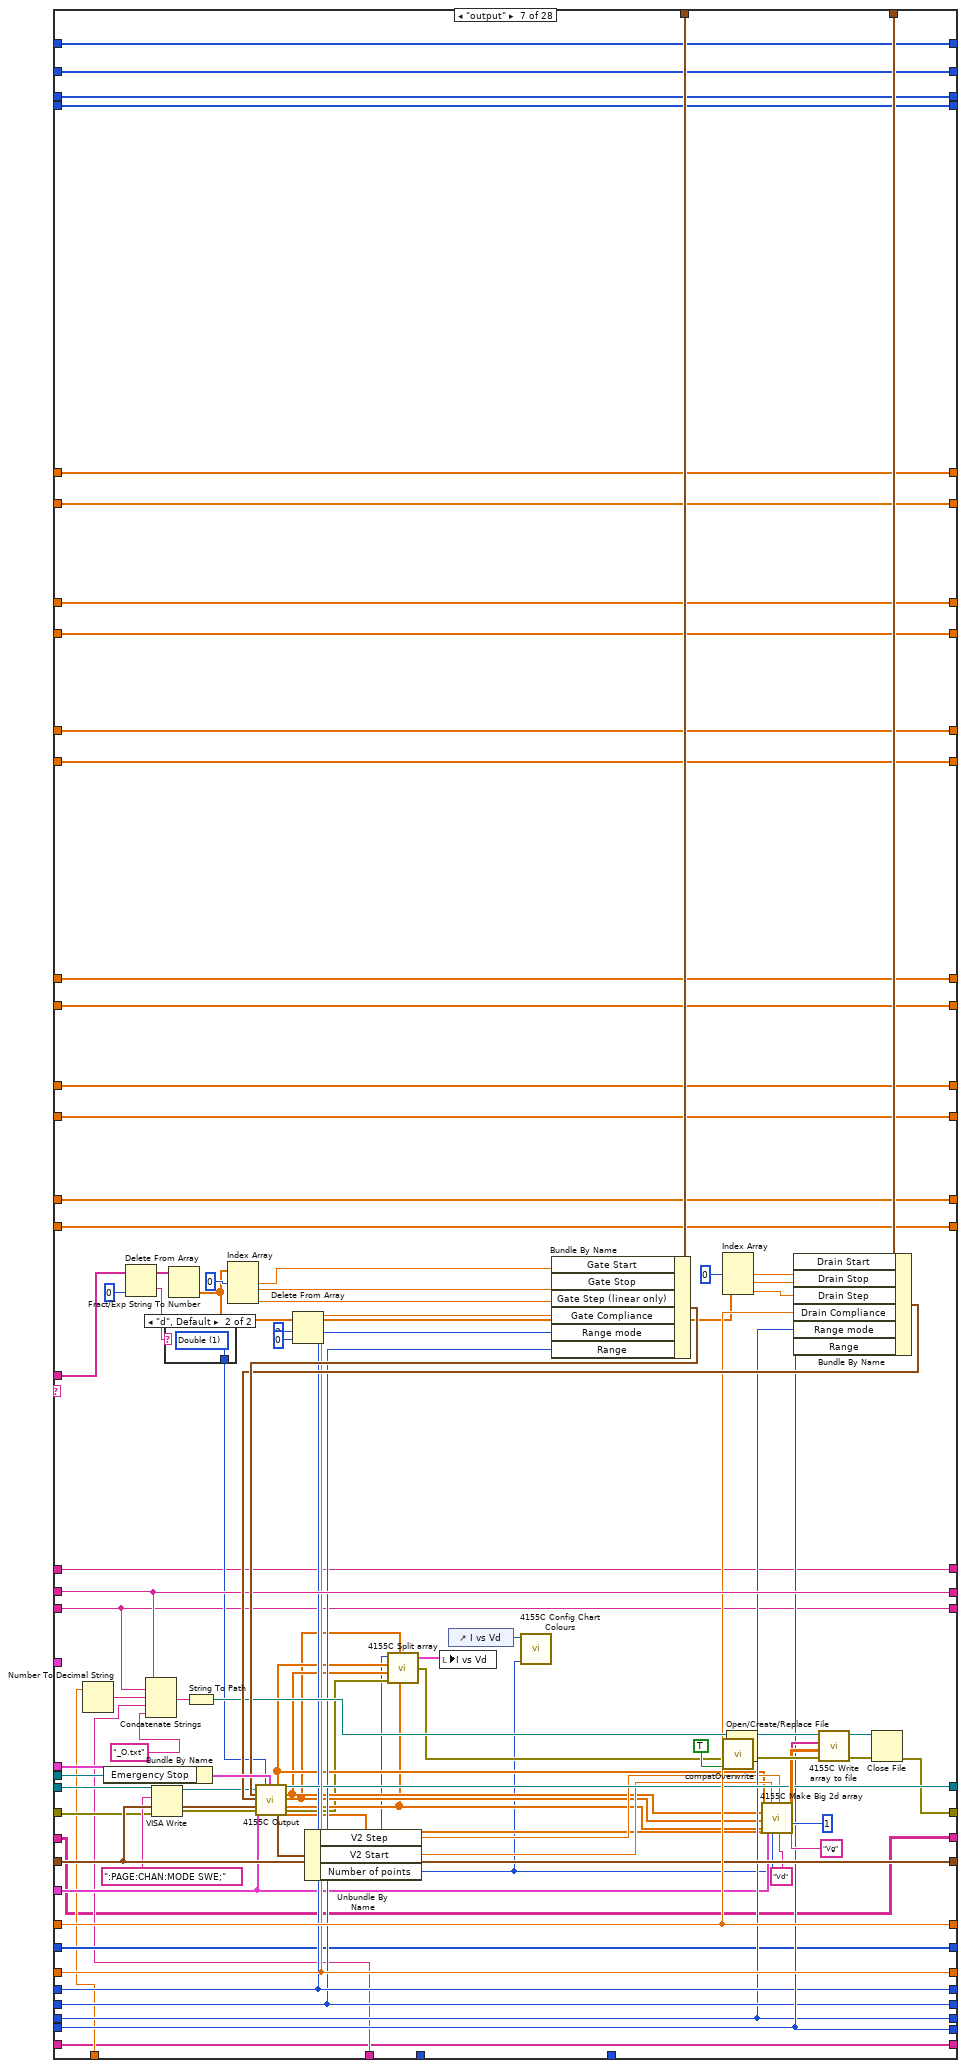
[diagram p14: hidden frame]
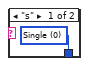
[diagram p15: hidden frame]
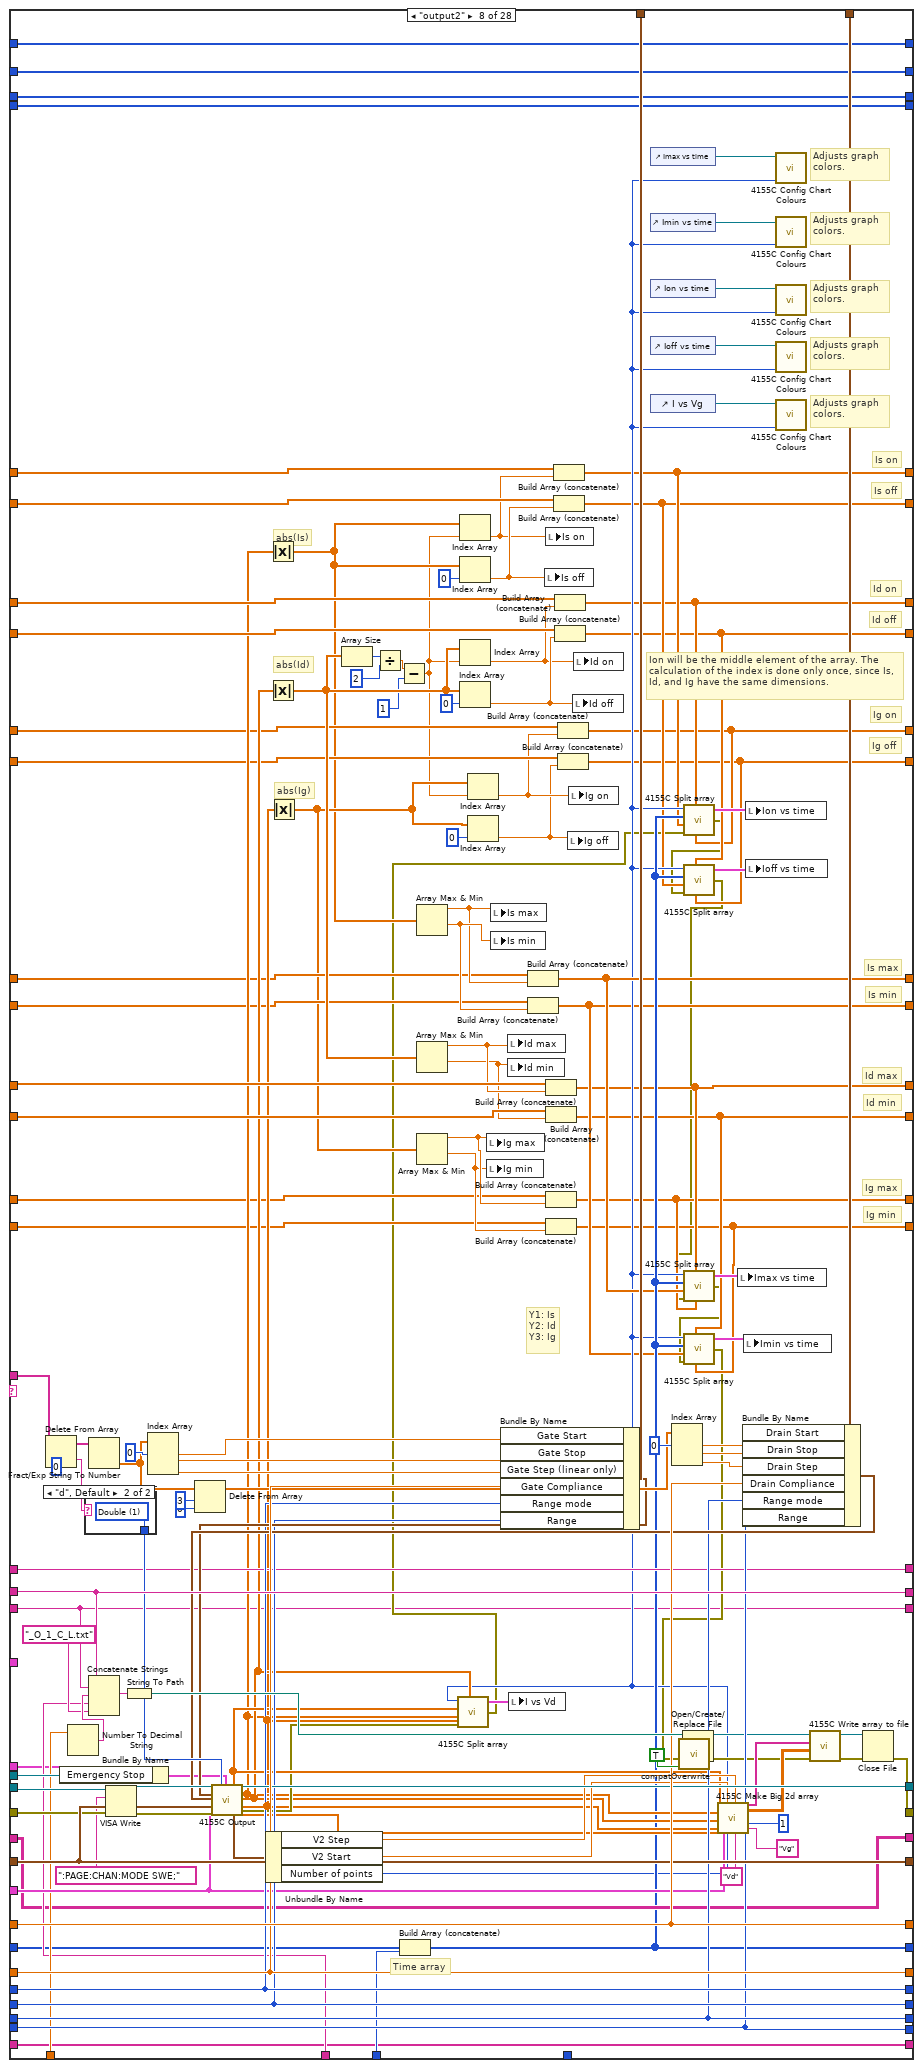
[diagram p16: hidden frame]
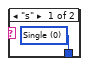
[diagram p17: hidden frame]
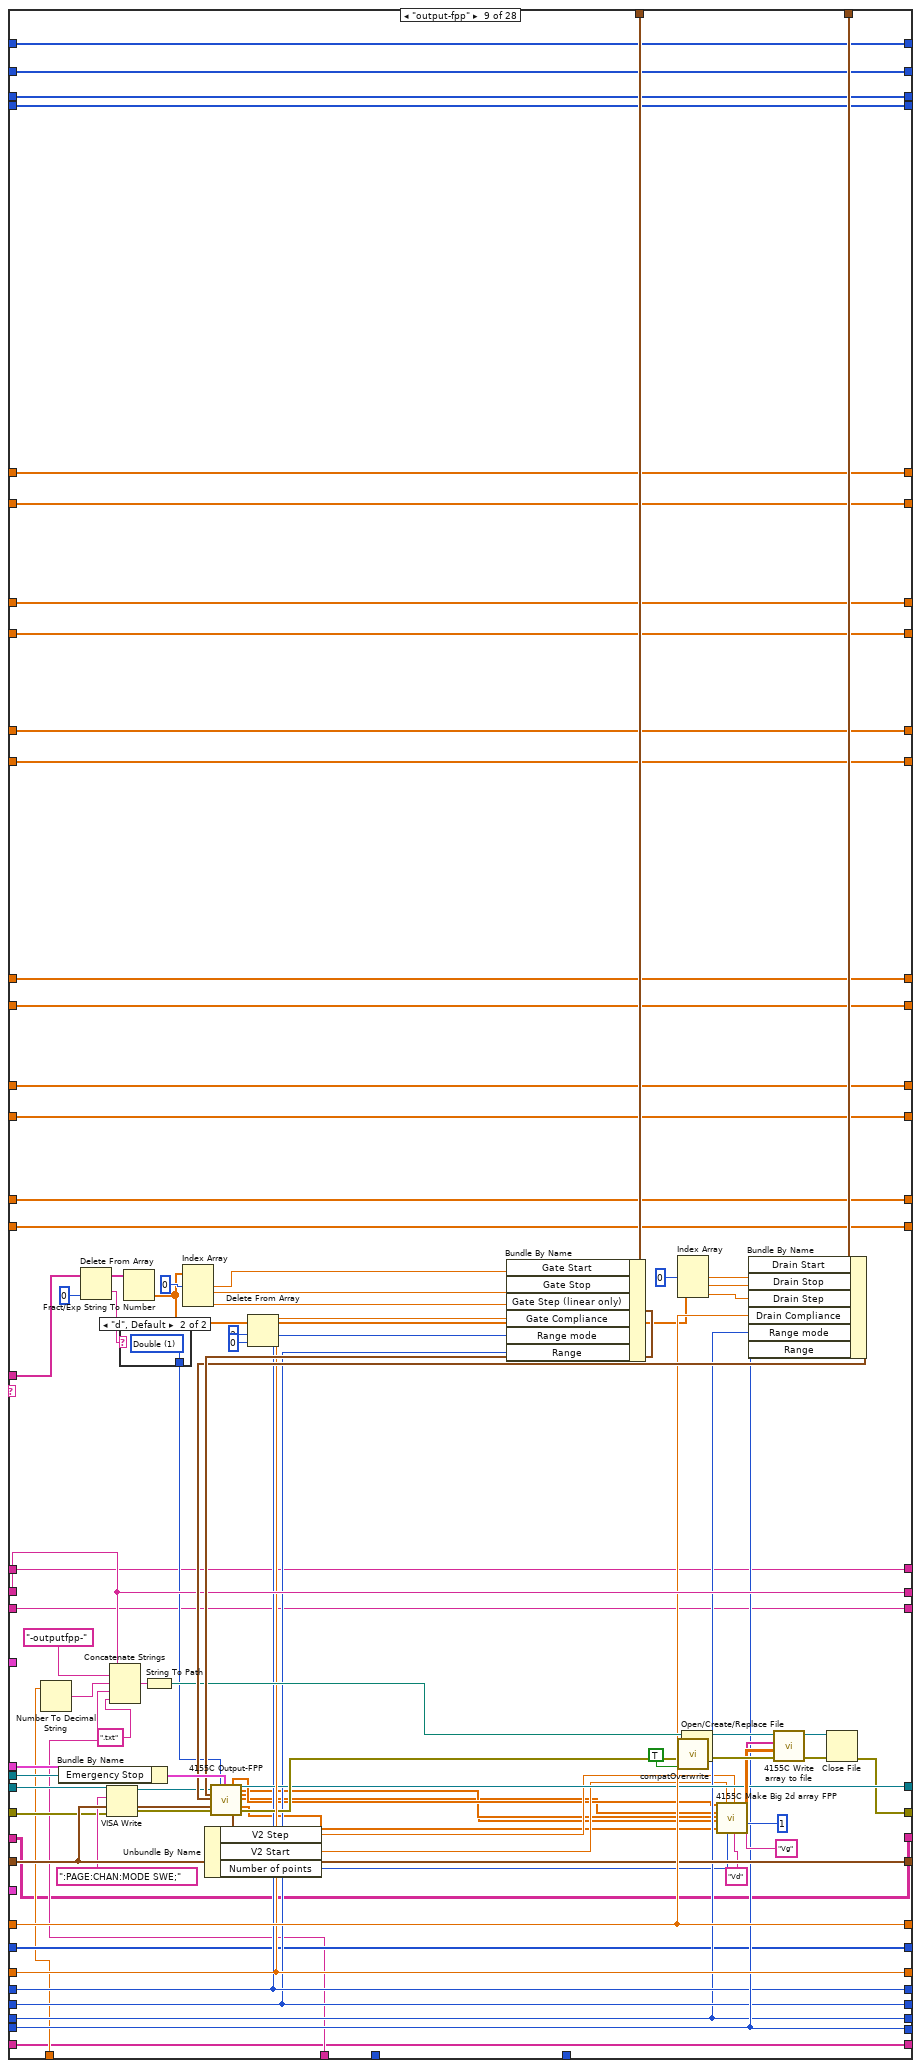
[diagram p18: hidden frame]
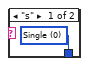
[diagram p19: hidden frame]
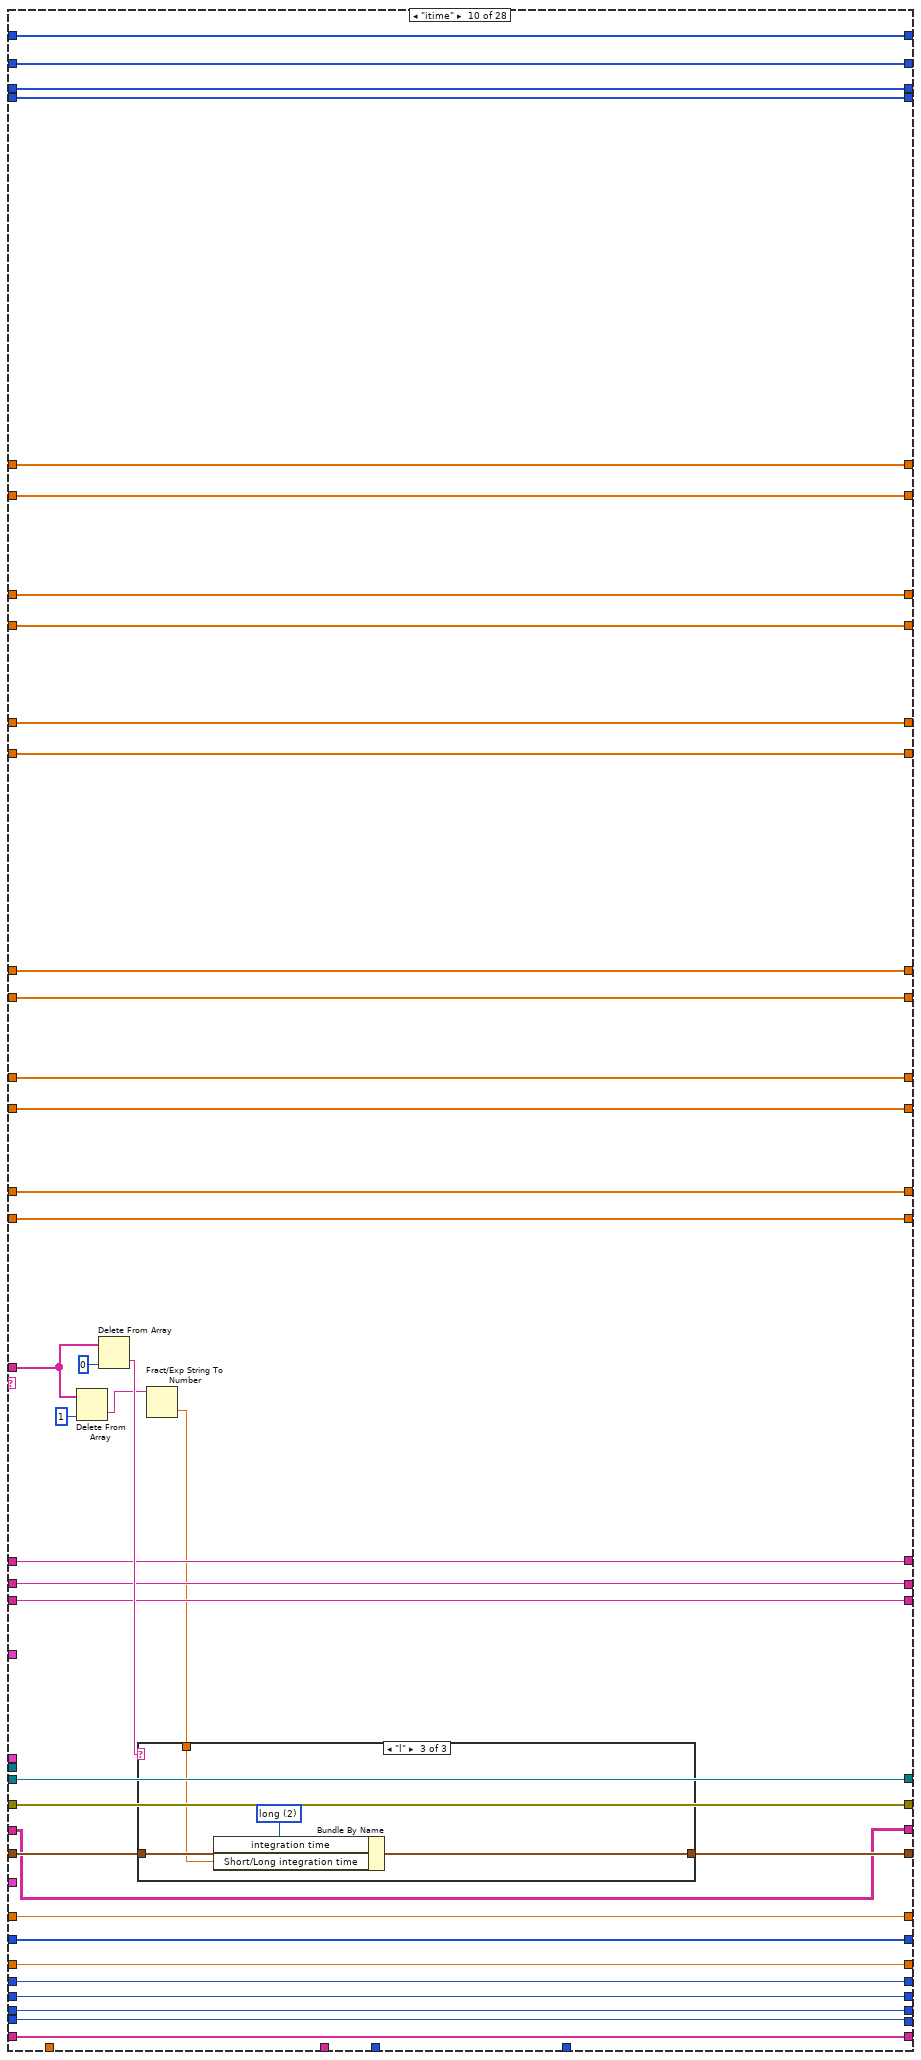
[diagram p20: hidden frame]
diagram:
  w4 = cluster{"Y data in":dbl[], "X data in":dbl[]}[] [] ("I vs Vg")
  w5 = 0.0 ("Is off")
  w6 = 0.0 ("Is on")
  w7 = 0.0 ("Is min")
  w8 = 0.0 ("Is max")
  w59 = u16 1 items=["Reset All", "Partial reset"] ("Type of reset")
  # "Change from previous version:\n\n- Added array initialization."
  # "This is a version specific to the SPM pump."
  # "I add 1 to both the \"total lines\" and the \"line running\" indicators because i and N begin from 0, and the script lines begin from 1."
  # "Bugs:\n\n- If using the \"filename\" command, keep in mind that the arrays of the time-dependent data are not re-initialized inbetween filename changes. \n\n- Do not connect the \"error\" wire of a Split block if it has unconnected terminals! It will halt the program."
  # "Array size"
  # "%s option converts a spreadsheet string to an array of strings."
  # "0: No of rows of array\n1: No of cols"
  # "Dimitrios Simatos\nv. 6.0"
  # "Changes from original textcontrol.vi:\n\n- Timestamp appears in filename.\n- (Only) transfer and output curves are plotted.\n- Communication with serial port.\n- Can execute any command, as all pattern matching functions were replaced. Previously, commands with special LabVIEW characters could not be executed.\n- Replaced write to file function with write to text file.\n- Replaced while loop with for loop.\n- Replaced 4155C \"Save File\" function and now the vi can save time-dependent variables.\n- Added clock with start time control and various units.\n- Changed filepath in which the program is saved.\n- Added a serial output log that keeps a history.\n- Tab control.\n- Addition of specialized serial read/write file for the SPM OEM pump.\n- Added halt and hard stop.\n- Imax, Imin, Ion, and Ioff are now saved for all Is, Id, and Ig.\n- Output curves are taken into account in Imax-Imin-Ion-Ioff plots (\"output2\" command).\n- Corrected bug of \"itime\" command. The command did not allow for settting the integration time value, it allowed to set the category of the integration time (short, medium, long). If the time value was beyond the range of the category, then the SPA used the closest value allowed, whilst staying in the category. So, if the integration time was changed to long, but the integration time value was a short one, then the SPA would measure using the minimum long integration time value and not the value that the user intended."
  # "Search and replace LF with EOL"
  n1 = Equal?(x="integration time", y=u32 0) -> (x = y?=w60:bool)
  n2 = Select(t="Integration time (short)", s=w60, f="Integration time (long)") -> (s? t:f=w9:dbl)
  n3 = Bundle By Name(cluster="Timings (overwritten by the Front Panel)", "integration time"="integration time", "Short/Long integration time"=w9) -> (w52:T5)
  n4 = call "4155C Get Filename.vi"("error in (no error)"=errorcluster {"status"=FALSE, "code"=0, "source"=""}) -> ("error out"=w54:errorcluster, "path"=w29:path)  [unwired: 2 in, 1 out]
  "Path" <- w29
  n5 = Path To String(path=w29) -> (string=w30:string)
  n6 = Search and Replace String(replace all?=TRUE ("replace all? (F)"), input string="Script", search string="\n", replace string="\r\n") -> (result string=w42:string)  [unwired: 4 in, 3 out]
  n7 = Match Pattern(string=w30, regular expression=".txt") -> (before substring=w25:string)  [unwired: 1 in, 3 out]
  n8 = Concatenate Strings(w25, "Suffix (script)") -> (w24:string)
  n9 = call "4155C Initialise.vi"("VISA resource name in"=refnum<visa-resource-name> "GPIB0::14::INSTR", "Reset"="Full Reset", "Type of reset"=w59, "error in (no error)"=w54, "VISA Timeout Value"=u32 10000) -> ("VISA Resource Name out"=w53:refnum<visa-resource-name>, "error out"=w22:errorcluster)
  n10 = Spreadsheet String To Array(delimiter (Tab)="\r\n", format string="%s", spreadsheet string="Script", array type (2D Dbl)="") -> (array=w33:string[][])
  n11 = Array Size(array=w33) -> (size(s)=w37:i32[])
  n12 = Initialize Array("") -> (w14:string[])  [unwired: 1 in]
  n13 = String To Path(string=w24) -> (path=w23:path)
  n14 = Initialize Array(0 ("element")) -> (w16:i32[])  [unwired: 1 in]
  n15 = Initialize Array("") -> (w12:string[][])  [unwired: 2 in]
  n16 = Initialize Array(0.0 ("element")) -> (w18:dbl[])  [unwired: 1 in]
  n17 = Index Array(array=w37, index=0) -> (element=w35:i32)
  n18 = Write to Text File(file (use dialog)=w23, text=w42, error in=w22) -> (error out=w21:errorcluster)  [unwired: 1 in, 2 out]
  n19 = for {
    N: w35 -> [w173]
    tunnel: "SMU4" -> [w209]
    shift-left: "Source/Drain Range" -> [w214]
    shift-right: [w210] -> _
    shift-left: "Source/Drain\nRange mode" -> [w215]
    shift-right: [w211] -> _
    shift-left: "Gate Range" -> [w216]
    shift-right: [w212] -> _
    shift-left: "Gate Range\nmode" -> [w217]
    shift-right: [w213] -> _
    shift-left: "Gate: Compliance" -> [w226]
    shift-right: [w222] -> _
    shift-left: "Drain: Compliance" -> [w227]
    shift-right: [w223] -> _
    shift-left: w52 -> [w228]
    shift-right: [w224] -> w10
    shift-left: w21 -> [w229]
    shift-right: [w119] -> w28
    shift-left: w53 -> [w230]
    shift-right: [w225] -> _
    shift-left: w25 -> [w231]
    shift-right: [w123] -> _
    tunnel: "Panel Controls 2" -> [w208]
    shift-right: [w81] -> _
    shift-left: w18 -> [w207]
    shift-right: [w143] -> _
    shift-left: i32[] [] -> [w203]
    tunnel: w33 -> [w202] mode=indexing
    shift-right: [w80] -> _
    shift-left: w18 -> [w179]
    shift-right: [w113] -> _
    shift-left: w14 -> [w165]
    shift-right: [w144] -> _
    shift-left: w16 -> [w160]
    shift-right: [w125] -> _
    shift-left: w16 -> [w159]
    shift-right: [w158] -> _
    shift-left: "" -> [w157]
    shift-right: [w118] -> _
    shift-left: w16 -> [w140]
    shift-right: [w117] -> _
    shift-left: w16 -> [w124]
    shift-right: [w114] -> _
    shift-left: w12 -> [w116]
    shift-right: [w74] -> _
    shift-left: w18 -> [w102]
    shift-right: [w75] -> _
    shift-left: w18 -> [w101]
    shift-right: [w79] -> _
    shift-left: w18 -> [w90]
    shift-right: [w78] -> _
    shift-left: w18 -> [w89]
    shift-right: [w72] -> _
    shift-left: w18 -> [w88]
    shift-right: [w82] -> _
    shift-left: w18 -> [w87]
    shift-right: [w73] -> _
    shift-left: w18 -> [w86]
    shift-right: [w71] -> _
    shift-left: w18 -> [w85]
    shift-right: [w77] -> _
    shift-left: w18 -> [w84]
    shift-right: [w76] -> _
    shift-left: w18 -> [w83]
    shift-right: [w66] -> _
    shift-left: "Filename (variable part)" -> [w65]
    i -> [w168]
    w104 = "Time (Minutes)" ("element")
    # "Filename prefix"
    # "Is off"
    # "Is on"
    # "Ig off"
    # "Ig on"
    # "Is min"
    # "Is max"
    # "Ig min"
    # "Ig max"
    # "Id min"
    # "Id max"
    # "Id off"
    # "Id on"
    # "Pump status"
    # "Filepath and name"
    # "Pump status"
    # "Limit of command arguments (array columns). Raise if needed."
    # "Serial port data (string)"
    # "Serial port data (table)"
    # "Time array for valve position"
    # "Time array for absolute plunger position"
    # "Valve position"
    # "Absolute plunger position"
    # "Serial port data"
    # "For loop counter"
    # "<-----Equivalent to the 4155C \"Write\" subvi.----->"
    # "Headers"
    # "Save transfer curves in file."
    # "Filepath and name"
    # "Save time-dependent data."
    # "Use the time offset if your measurements do not start at t=0."
    # "Time for Imax, Imin, Ion, Ioff"
    # "Rest of elements of command"
    # "First element of command\n(case select)"
    n20 = Add(x=w168, y=1) -> (x+y=→"Line running":i32)
    n21 = Add(x=w173, y=1) -> (x+y=→"Total lines":i32)
    n22 = Index Array(array=w202, index=0 ("line index")) -> (element=w197:string)
    "Command running:" <- w197
    n23 = control-ref of="Interrupt run"() -> (w221:refnum<vi>)
    n24 = Spreadsheet String To Array(delimiter (Tab)=" ", format string="%s", spreadsheet string=w197, array type (2D Dbl)=string[] []) -> (array=w195:string[])
    n25 = Delete From Array(array=w195, index=0) -> (deleted portion=w103:string, array with subset deleted=w194:string[])  [unwired: 1 in]
    n26 = call "Elapsed Time"("Reset"="Reset", "Auto Reset"="Auto Reset") -> ("Elapsed Time (s)"=w204:dbl)  [unwired: 10 in, 7 out]
    n27 = case shown="0, Default" "Units (label only)" {
      tunnel: ["_sec" "_min" "_h"] -> w205
      tunnel: [w232 w236 w239] -> w175
      tunnel: w204 -> [w232 w235 w240]
      frame 0, Default {
      }
      frame 1 {
        n28 = Divide(x=w235, y=60.0) -> (x/y=w236:dbl)
      }
      frame 2 {
        n29 = Divide(x=w240, y=3600.0) -> (x/y=w239:dbl)
      }
    }
    n30 = Add(x=w175, y="Time Offset") -> (x+y=w174:dbl)
    n31 = To Long Integer(number=w174) -> (32bit integer=w141:i32)
    "Elapsed Time" <- w141
    n32 = case shown="\"serial\"" w103 {
      tunnel: w194 -> [w277 w315 w352 w484 w508 w654 w748 w900 w978 w1005 w1085 w1131 w1175 w1215 w1248 _ _ w1409 w1489 _ w1592 w1655 w1716 w1805 w1886 w1925 w1995 w2049]
      tunnel: w231 -> [w272 w311 w350 w491 w573 w662 w755 w907 w986 w1028 w1074 w1123 w1168 w1209 w1241 w1279 w1340 w1387 w1471 w1521 w1579 w1642 w1704 w1799 w1882 w1927 w1997 w2051]
      tunnel: w230 -> [w271 w310 w341 w462 w558 w631 w724 w878 w954 w1029 w1075 w1124 w1169 w1210 w1242 w1284 w1342 w1415 w1495 w1525 w1598 w1661 w1722 w1811 w1840 w1931 w2001 w2053]
      tunnel: w229 -> [w270 w309 w340 w461 w557 w630 w721 w877 w951 w1030 w1076 w1125 w1170 w1211 w1243 w1283 w1313 w1414 w1494 w1524 w1597 w1660 w1721 w1810 w1839 w1930 w2000 w2054]
      tunnel: w228 -> [w269 w308 w349 w487 w533 w658 w751 w903 w982 w1038 w1084 w1122 w1167 w1208 w1240 w1282 w1337 w1378 w1463 w1530 w1572 w1635 w1697 w1798 w1881 w1932 w2002 w2056]
      tunnel: w227 -> [w268 w307 w348 w489 w571 w660 w753 w905 w984 w1037 w1083 w1130 w1174 w1214 w1247 w1281 w1322 w1413 w1493 w1533 w1596 w1659 w1720 w1809 w1890 w1933 w2003 w2057]
      tunnel: w226 -> [w267 w306 w347 w488 w570 w659 w752 w904 w983 w1036 w1082 w1129 w1173 w1213 w1246 w1280 w1323 w1388 w1472 w1532 w1580 w1643 w1705 w1800 w1883 w1935 w2004 w2059]
      tunnel: [w271 w310 w339 w486 w568 w656 w750 w902 w980 w1029 w1075 w1124 w1169 w1210 w1242 w1284 w1342 w1379 w1445 w1523 w1573 w1636 w1698 w1751 w1842 w1931 w2001 w2053] -> w225
      tunnel: [w270 w309 w338 w485 w567 w655 w749 w901 w979 w1030 w1076 w1125 w1170 w1211 w1243 w1283 w1312 w1389 w1446 w1522 w1581 w1644 w1706 w1750 w1841 w1929 w1999 w2054] -> w139
      tunnel: [w269 w308 w349 w487 w529 w658 w751 w903 w982 w1031 w1077 w1122 w1167 w1208 w1240 w1282 w1337 w1378 w1463 w1530 w1572 w1635 w1697 w1798 w1881 w1932 w2002 w2056] -> w224
      tunnel: [w268 w307 w348 w489 w571 w660 w753 w905 w984 w1037 w1083 w1130 w1174 w1214 w1247 w1281 w1322 w1413 w1493 w1533 w1596 w1659 w1720 w1809 w1890 w1933 w2003 w2057] -> w223
      tunnel: [w267 w306 w347 w488 w570 w659 w752 w904 w983 w1036 w1082 w1129 w1173 w1213 w1246 w1280 w1323 w1388 w1472 w1532 w1580 w1643 w1705 w1800 w1883 w1935 w2004 w2059] -> w222
      tunnel: [w272 w311 w350 w491 w573 w662 w755 w907 w986 w1028 w1074 w1123 w1168 w1209 w1241 w1279 w1340 w1387 w1471 w1521 w1579 w1642 w1704 w1799 w1882 w1927 w1997 w2051] -> w123
      tunnel: w221 -> [_ _ _ w493 w577 w667 w758 w909 w990 _ _ _ _ _ _ _ _ w1384 w1468 _ w1578 w1641 w1703 w1771 w1858 _ _ _]
      tunnel: "Gate" -> [_ _ _ w471 w561 w641 w735 w887 w965 _ _ _ _ _ _ _ _ _ _ _ _ _ _ _ _ _ _ _]
      tunnel: "Drain 2" -> [_ _ _ w470 w560 w640 w734 w886 w964 _ _ _ _ _ _ _ _ _ _ _ _ _ _ _ _ _ _ _]
      tunnel: "Panel Controls" -> [_ _ _ _ _ w639 w733 w771 w963 _ _ _ _ _ _ _ _ _ _ _ _ _ _ _ _ _ _ _]
      tunnel: w217 -> [w266 w305 w346 w455 w551 w624 w719 w871 w949 w1035 w1081 _ w1166 w1207 w1239 w1278 w1324 w1374 w1459 w1526 w1568 w1631 w1693 w1794 w1877 w1936 w2005 w2060]
      tunnel: w216 -> [w265 w304 w345 w454 w550 w623 w718 w870 w948 w1034 w1080 w1128 _ w1198 w1245 w1277 w1325 w1375 w1460 w1527 w1569 w1632 w1694 w1795 w1878 w1937 w2006 w2061]
      tunnel: w215 -> [w264 w303 w344 w453 w549 w622 w717 w869 w947 w1033 w1079 w1127 w1172 w1212 _ w1276 w1326 w1376 w1461 w1528 w1570 w1633 w1695 w1796 w1879 w1938 w2007 w2062]
      tunnel: w214 -> [w263 w302 w343 w452 w548 w621 w720 w868 w950 w1032 w1078 w1126 w1171 _ w1244 w1275 w1327 w1377 w1462 w1529 w1571 w1634 w1696 w1797 w1880 w1939 w2008 w2063]
      tunnel: [w266 w305 w346 w455 w551 w624 w719 w871 w949 w1035 w1081 w1121 w1166 w1207 w1239 w1278 w1324 w1374 w1459 w1526 w1568 w1631 w1693 w1794 w1877 w1936 w2005 w2060] -> w213
      tunnel: [w265 w304 w345 w454 w550 w623 w718 w870 w948 w1034 w1080 w1128 w1158 w1198 w1245 w1277 w1325 w1375 w1460 w1527 w1569 w1632 w1694 w1795 w1878 w1937 w2006 w2061] -> w212
      tunnel: [w264 w303 w344 w453 w549 w622 w717 w869 w947 w1033 w1079 w1127 w1172 w1212 w1238 w1276 w1326 w1376 w1461 w1528 w1570 w1633 w1695 w1796 w1879 w1938 w2007 w2062] -> w211
      tunnel: [w263 w302 w343 w452 w548 w621 w720 w868 w950 w1032 w1078 w1126 w1171 w1199 w1244 w1275 w1327 w1377 w1462 w1529 w1571 w1634 w1696 w1797 w1880 w1939 w2008 w2063] -> w210
      tunnel: w209 -> [_ _ _ w447 w545 _ w713 w863 _ _ _ _ _ _ _ _ _ _ _ _ _ _ _ _ _ _ _ _]
      tunnel: w208 -> [_ _ _ w445 w544 _ _ _ _ _ _ _ _ _ _ _ _ _ _ _ _ _ _ _ _ _ _ _]
      tunnel: [w262 w298 w336 w373 w521 w611 w710 w790 w936 w1027 w1072 w1120 w1157 w1197 w1237 w1274 w1308 w1366 w1424 w1520 w1557 w1624 w1687 w1748 w1835 w1928 w1998 w2068] -> w81
      tunnel: w207 -> [w262 w298 w336 w442 w521 w611 w710 w859 w936 w1027 w1072 w1120 w1157 w1197 w1237 w1274 w1308 w1366 w1424 w1520 w1557 w1624 w1687 w1748 w1835 w1928 w1998 w2068]
      tunnel: w174 -> [_ _ _ w439 w518 w609 w707 w856 w933 _ _ _ _ _ _ _ w1306 w1364 w1441 _ w1554 w1621 w1684 w1745 w1831 _ _ _]
      tunnel: w205 -> [_ _ _ w436 w517 w607 w706 w853 w932 _ _ _ _ _ _ _ w1304 w1362 w1440 _ w1553 w1620 w1683 w1744 w1832 _ w1966 _]
      tunnel: w141 -> [_ _ _ w431 _ _ _ w848 _ _ _ _ _ _ _ _ _ _ _ _ _ _ _ _ _ _ w1969 _]
      tunnel: [w261 w297 w335 w381 w520 w610 w709 w798 w935 w1026 w1071 w1119 w1156 w1196 w1236 w1273 w1307 w1365 w1443 w1519 w1556 w1623 w1686 w1747 w1834 w1934 w1978 w2058] -> w143
      tunnel: w203 -> [w261 w297 w335 w435 w520 w610 w709 w852 w935 w1026 w1071 w1119 w1156 w1196 w1236 w1273 w1307 w1365 w1443 w1519 w1556 w1623 w1686 w1747 w1834 w1934 w1978 w2058]
      tunnel: [w260 w296 w334 w372 w516 w606 w705 w789 w931 w1025 w1070 w1118 w1155 w1195 w1235 w1272 w1303 w1361 w1423 w1518 w1552 w1619 w1682 w1743 w1830 w1923 w1994 w2067] -> w80
      tunnel: w179 -> [w260 w296 w334 w429 w516 w606 w705 w846 w931 w1025 w1070 w1118 w1155 w1195 w1235 w1272 w1303 w1361 w1423 w1518 w1552 w1619 w1682 w1743 w1830 w1923 w1994 w2067]
      tunnel: [w259 w295 w333 w422 w515 w605 w695 w839 w930 w1024 w1069 w1117 w1154 w1194 w1234 w1271 w1302 w1360 w1439 w1517 w1551 w1618 w1681 w1742 w1829 w1922 w1993 w2064] -> w113
      tunnel: w165 -> [w259 w295 w333 w422 w515 w605 w695 w839 w930 w1024 w1069 w1117 w1154 w1194 w1234 w1271 w1302 w1360 w1439 w1517 w1551 w1618 w1681 w1742 w1829 w1921 w1967 w2064]
      tunnel: [w258 w294 w332 w421 w514 w604 w694 w838 w929 w1023 w1068 w1116 w1153 w1193 w1233 w1270 w1301 w1359 w1438 w1516 w1550 w1617 w1680 w1741 w1828 w1907 w1980 w2078] -> w144
      tunnel: w160 -> [w258 w294 w332 w421 w514 w604 w694 w838 w929 w1023 w1068 w1116 w1153 w1193 w1233 w1270 w1301 w1359 w1438 w1516 w1550 w1617 w1680 w1741 w1828 w1907 w1979 w2078]
      tunnel: [w257 w293 w331 w420 w513 w603 w693 w837 w928 w1022 w1067 w1115 w1152 w1192 w1232 w1269 w1300 w1358 w1437 w1515 w1549 w1616 w1679 w1740 w1827 w1906 w1962 w2080] -> w125
      tunnel: w159 -> [w257 w293 w331 w420 w513 w603 w693 w837 w928 w1022 w1067 w1115 w1152 w1192 w1232 w1269 w1300 w1358 w1437 w1515 w1549 w1616 w1679 w1740 w1827 w1906 w1960 w2080]
      tunnel: [w256 w292 w330 w419 w512 w602 w692 w836 w927 w1021 w1066 w1114 w1151 w1191 w1231 w1268 w1299 w1357 w1436 w1514 w1548 w1615 w1678 w1739 w1826 w1905 w1959 w2052] -> w158
      tunnel: w157 -> [w256 w292 w330 w419 w512 w602 w692 w836 w927 w1021 w1066 w1114 w1151 w1191 w1231 w1268 w1299 w1357 w1436 w1514 w1548 w1615 w1678 w1739 w1826 w1905 w1970 w2052]
      tunnel: w141 -> [_ _ _ _ _ _ _ _ _ _ _ _ _ _ _ _ _ _ _ _ _ _ _ _ _ _ w1958 _]
      tunnel: w140 -> [w255 w291 w329 w418 w511 w601 w691 w835 w926 w1020 w1065 w1113 w1150 w1190 w1230 w1267 w1298 w1356 w1435 w1513 w1547 w1614 w1677 w1738 w1825 w1904 w1957 w2079]
      tunnel: [w255 w291 w329 w418 w511 w601 w691 w835 w926 w1020 w1065 w1113 w1150 w1190 w1230 w1267 w1298 w1356 w1435 w1513 w1547 w1614 w1677 w1738 w1825 w1904 w1956 w2079] -> w118
      tunnel: [w254 w290 w328 w417 w510 w600 w690 w834 w925 w1019 w1064 w1112 w1149 w1189 w1229 w1266 w1297 w1355 w1434 w1512 w1546 w1613 w1676 w1737 w1824 w1903 w1955 w2077] -> w117
      tunnel: w124 -> [w254 w290 w328 w417 w510 w600 w690 w834 w925 w1019 w1064 w1112 w1149 w1189 w1229 w1266 w1297 w1355 w1434 w1512 w1546 w1613 w1676 w1737 w1824 w1903 w1954 w2077]
      tunnel: [w253 w289 w327 w416 w509 w599 w689 w833 w924 w1018 w1063 w1111 w1148 w1188 w1228 w1265 w1296 w1354 w1433 w1511 w1545 w1612 w1675 w1736 w1823 w1902 w1952 w2055] -> w114
      tunnel: w116 -> [w253 w289 w327 w416 w509 w599 w689 w833 w924 w1018 w1063 w1111 w1148 w1188 w1228 w1265 w1296 w1354 w1433 w1511 w1545 w1612 w1675 w1736 w1823 w1902 w1951 w2055]
      tunnel: [w251 w287 w325 w366 w506 w597 w687 w783 w922 w1016 w1062 w1110 w1146 w1186 w1226 w1263 w1294 w1353 w1432 w1510 w1544 w1611 w1673 w1735 w1822 w1901 w1950 w2073] -> w74
      tunnel: w102 -> [w251 w287 w325 w412 w506 w597 w687 w829 w922 w1016 w1062 w1110 w1146 w1186 w1226 w1263 w1294 w1353 w1432 w1510 w1544 w1611 w1673 w1735 w1822 w1901 w1950 w2073]
      tunnel: [w252 w288 w326 w367 w507 w598 w688 w784 w923 w1017 w1061 w1109 w1147 w1187 w1227 w1264 w1295 w1352 w1431 w1509 w1543 w1610 w1674 w1734 w1821 w1900 w1949 w2074] -> w75
      tunnel: w101 -> [w252 w288 w326 w411 w507 w598 w688 w828 w923 w1017 w1061 w1109 w1147 w1187 w1227 w1264 w1295 w1352 w1431 w1509 w1543 w1610 w1674 w1734 w1821 w1900 w1949 w2074]
      tunnel: [w244 w280 w318 w371 w503 w595 w685 w788 w920 w1009 w1059 w1107 w1144 w1184 w1224 w1261 w1287 w1345 w1422 w1508 w1536 w1603 w1666 w1727 w1816 w1893 w1948 w2066] -> w79
      tunnel: w90 -> [w244 w280 w318 w401 w503 w595 w685 w818 w920 w1009 w1059 w1107 w1144 w1184 w1224 w1261 w1287 w1345 w1422 w1508 w1536 w1603 w1666 w1727 w1816 w1893 w1948 w2066]
      tunnel: [w243 w279 w317 w370 w504 w596 w686 w787 w921 w1008 w1060 w1108 w1145 w1185 w1225 w1262 w1286 w1344 w1421 w1507 w1535 w1602 w1665 w1726 w1815 w1892 w1947 w2065] -> w78
      tunnel: w89 -> [w243 w279 w317 w400 w504 w596 w686 w817 w921 w1008 w1060 w1108 w1145 w1185 w1225 w1262 w1286 w1344 w1421 w1507 w1535 w1602 w1665 w1726 w1815 w1892 w1947 w2065]
      tunnel: [w246 w282 w320 w376 w502 w593 w683 w793 w918 w1014 w1057 w1105 w1142 w1182 w1222 w1259 w1289 w1347 w1426 w1502 w1538 w1605 w1668 w1729 w1814 w1897 w1945 w2070] -> w72
      tunnel: w88 -> [w246 w282 w320 w397 w502 w593 w683 w814 w918 w1014 w1057 w1105 w1142 w1182 w1222 w1259 w1289 w1347 w1426 w1502 w1538 w1605 w1668 w1729 w1814 w1897 w1945 w2070]
      tunnel: [w245 w281 w319 w374 w505 w594 w684 w791 w919 w1015 w1058 w1106 w1143 w1183 w1223 w1260 w1288 w1346 w1425 w1501 w1537 w1604 w1667 w1728 w1813 w1896 w1946 w2069] -> w82
      tunnel: w87 -> [w245 w281 w319 w396 w505 w594 w684 w813 w919 w1015 w1058 w1106 w1143 w1183 w1223 w1260 w1288 w1346 w1425 w1501 w1537 w1604 w1667 w1728 w1813 w1896 w1946 w2069]
      tunnel: [w248 w284 w322 w365 w501 w591 w681 w782 w916 w1012 w1055 w1103 w1140 w1180 w1220 w1257 w1291 w1349 w1428 w1504 w1540 w1607 w1670 w1731 w1818 w1899 w1943 w2072] -> w73
      tunnel: w86 -> [w248 w284 w322 w393 w501 w591 w681 w810 w916 w1012 w1055 w1103 w1140 w1180 w1220 w1257 w1291 w1349 w1428 w1504 w1540 w1607 w1670 w1731 w1818 w1899 w1943 w2072]
      tunnel: [w247 w283 w321 w364 w500 w592 w682 w781 w917 w1013 w1056 w1104 w1141 w1181 w1221 w1258 w1290 w1348 w1427 w1503 w1539 w1606 w1669 w1730 w1817 w1898 w1944 w2071] -> w71
      tunnel: w85 -> [w247 w283 w321 w392 w500 w592 w682 w809 w917 w1013 w1056 w1104 w1141 w1181 w1221 w1258 w1290 w1348 w1427 w1503 w1539 w1606 w1669 w1730 w1817 w1898 w1944 w2071]
      tunnel: [w250 w286 w324 w369 w499 w589 w679 w786 w914 w1010 w1053 w1101 w1138 w1178 w1218 w1255 w1293 w1351 w1430 w1506 w1542 w1609 w1672 w1733 w1820 w1895 w1941 w2076] -> w77
      tunnel: w84 -> [w250 w286 w324 w389 w499 w589 w679 w806 w914 w1010 w1053 w1101 w1138 w1178 w1218 w1255 w1293 w1351 w1430 w1506 w1542 w1609 w1672 w1733 w1820 w1895 w1941 w2076]
      tunnel: [w249 w285 w323 w368 w498 w590 w680 w785 w915 w1011 w1054 w1102 w1139 w1179 w1219 w1256 w1292 w1350 w1429 w1505 w1541 w1608 w1671 w1732 w1819 w1894 w1942 w2075] -> w76
      tunnel: w83 -> [w249 w285 w323 w388 w498 w590 w680 w805 w915 w1011 w1054 w1102 w1139 w1179 w1219 w1256 w1292 w1350 w1429 w1505 w1541 w1608 w1671 w1732 w1819 w1894 w1942 w2075]
      tunnel: w65 -> [w242 w278 w316 w355 w497 w588 w678 w772 w913 w1007 w1052 w1100 w1137 w1177 w1217 w1254 w1285 w1343 w1420 w1500 w1534 w1601 w1664 w1725 w1812 w1891 w1940 _]
      tunnel: [w242 w278 w316 w355 w497 w588 w678 w772 w913 w1007 w1052 w1100 w1137 w1177 w1217 w1254 w1285 w1343 w1420 w1500 w1534 w1601 w1664 w1725 w1812 w1891 w1940 w2048] -> w66
      frame "wait" {
        n33 = Index Array(array=w277, index=0 ("Index")) -> (element=w275:string)
        n34 = Decimal String To Number(string=w275, default (0L)=u32 0) -> (number=w274:u32)  [unwired: 1 in, 1 out]
        n35 = Wait (ms)(milliseconds to wait=w274) -> ()  [unwired: 1 out]
      }
      frame "wait-min" {
        n36 = Index Array(array=w315, index=0 ("Index")) -> (element=w313:string)
        n37 = Decimal String To Number(string=w313, default (0L)=u32 0) -> (number=w301:u32)  [unwired: 1 in, 1 out]
        n38 = Multiply(x=w301, y=u32 60000) -> (x*y=w300:u32)
        n39 = Wait (ms)(milliseconds to wait=w300) -> ()  [unwired: 1 out]
      }
      frame "standby" {
        n40 = Index Array(array=w352, index=0 ("Index")) -> (element=w342:string)
        n41 = case shown="\"off\", Default" w342 {
          tunnel: [":PAGE:SCON:STAN 0" ":PAGE:SCON:STAN 1"] -> w337
          frame "off", Default {
          }
          frame "on" {
          }
        }
        n42 = VISA Write(VISA resource name=w341, write buffer=w337, error in (no error)=w340) -> (VISA resource name out=w339:refnum<visa-resource-name>, error out=w338:errorcluster)  [unwired: 1 out]
      }
      frame "transfer" {
        # "Adjusts graph colors."
        # "Adjusts graph colors."
        # "Is off"
        # "Is on"
        # "Ion will be the middle element of the array. The calculation of the index is done only once, since Is, Id, and Ig have the same dimensions."
        # "Ig off"
        # "Ig on"
        # "Is min"
        # "Is max"
        # "Ig min"
        # "Ig max"
        # "abs(Ig)"
        # "abs(Is)"
        # "Id min"
        # "Id max"
        # "Y1: Is\nY2: Id\nY3: Ig"
        # "abs(Id)"
        # "Adjusts graph colors."
        # "Adjusts graph colors."
        # "Id off"
        # "Id on"
        # "Adjusts graph colors."
        # "Time array"
        n43 = Delete From Array(array=w484, index=0 ("Index")) -> (deleted portion=w482:string, array with subset deleted=w481:string[])  [unwired: 1 in]
        n44 = Bundle By Name(cluster=w445, "Emergency Stop"=w493) -> (w446:T2)
        n45 = Number To Decimal String(number=w439) -> (decimal integer string=w438:string)  [unwired: 1 in]
        n46 = case shown="\"d\", Default" w482 {
          tunnel: [w495 w496] -> w480
          frame "s" {
            w495 = u16 0 items=["Single", "Double"] ("sweep mode")
          }
          frame "d", Default {
            w496 = u16 1 items=["Single", "Double"] ("sweep mode")
          }
        }
        n47 = Fract/Exp String To Number(string=w481) -> (number=w466:dbl[])  [unwired: 3 in, 1 out]
        n48 = Concatenate Strings(w491, w355, w438, w436, "_T_1_C_L.txt" ("Suffix (transfer)")) -> (w492:string)
        n49 = VISA Write(VISA resource name=w462, write buffer=":PAGE:CHAN:MODE SWE;" ("write buffer (\"\")"), error in (no error)=w461) -> (VISA resource name out=w459:refnum<visa-resource-name>, error out=w460:errorcluster)  [unwired: 1 out]
        n50 = String To Path(string=w492) -> (path=w490:path)
        n51 = Index Array(array=w466, index #1=0 ("Index")) -> (element #1=w479:dbl, element #2=w478:dbl, element #3=w477:dbl)  [unwired: 2 in]
        n52 = Delete From Array(array=w466, length=3 ("Length"), index=0 ("Index")) -> (array with subset deleted=w464:dbl[])  [unwired: 1 out]
        n53 = Build Array (concatenate)(w435, w431) -> (w381:i32[])
        n54 = Bundle By Name(cluster=w471, "Gate Start"=w479, "Gate Stop"=w478, "Gate Step (linear only)"=w477, "Gate Compliance"=w488, "Range mode"=w455, "Range"=w454) -> (w456:T6)
        n55 = control-ref of="Imax vs time"() -> (w410:refnum<vi>)
        n56 = control-ref of="Imin vs time"() -> (w409:refnum<vi>)
        n57 = control-ref of="Ion vs time"() -> (w378:refnum<vi>)
        n58 = control-ref of="Ioff vs time"() -> (w377:refnum<vi>)
        n59 = control-ref of="I vs Vg"() -> (w440:refnum<vi>)
        n60 = Index Array(array=w464, index #1=0 ("Index")) -> (element #1=w474:dbl, element #2=w473:dbl, element #3=w472:dbl)  [unwired: 2 in]
        n61 = call <vilib>:"compatOverwrite.vi"("overwrite (F)"=TRUE) -> ("overwrite?"=w444:T8)
        n62 = Bundle By Name(cluster=w470, "Drain Start"=w474, "Drain Stop"=w473, "Drain Step"=w472, "Drain Compliance"=w489, "Range mode"=w453, "Range"=w452) -> (w457:T7)
        n63 = call "4155C Transfer.vi"("VISA resource name in"=w459, "Gate"=w456, "Drain"=w457, "Timings"=w487, "error in (no error)"=w460, "SMU4"=w447, "sweep mode"=w480, "Panel Controls"=w446) -> ("VG"=w443:dbl[], "Outparams"=w451:T9, "VISA Resource Name out"=w486:refnum<visa-resource-name>, "IS"=w406:dbl[], "ID"=w408:dbl[], "IG"=w405:dbl[], "error out"=w432:errorcluster, "SMU4"=w448:dbl[])  [unwired: 12 in]
        n64 = Unbundle By Name(w451) -> ("V2 Step"=w450:dbl, "V2 Start"=w449:dbl, "Number of points"=w375:i32)
        n65 = Absolute Value(x=w406) -> (abs(x)=w391:dbl[])
        n66 = Absolute Value(x=w408) -> (abs(x)=w407:dbl[])
        n67 = Absolute Value(x=w405) -> (abs(x)=w394:dbl[])
        n68 = Array Size(array=w407) -> (size(s)=w415:i32)
        n69 = Divide(x=w415, y=2) -> (x/y=w358:dbl)
        n70 = Subtract(x=w358, y=1) -> (x-y=w357:dbl)
        n71 = Array Max & Min(array=w391) -> (max value=w398:dbl, min value=w399:dbl)  [unwired: 2 out]
        n72 = Array Max & Min(array=w407) -> (max value=w441:dbl, min value=w404:dbl)  [unwired: 2 out]
        n73 = Array Max & Min(array=w394) -> (max value=w403:dbl, min value=w402:dbl)  [unwired: 2 out]
        n74 = call "4155C Split array.vi"("Number of VAR2 steps"=w375, "Y2 data in"=w408, "X data in"=w443, "Y1 data in"=w406, "Y3 data in"=w405, "error in (no error)"=w432) -> ("Array of clusters"=w434:cluster{"Y data in":dbl[], "X data in":dbl[]}[], "error out"=w363:errorcluster)  [unwired: 1 in]
        n75 = Index Array(array=w391, index=w357) -> (element=w382:dbl)
        n76 = Index Array(array=w391, index=0) -> (element=w383:dbl)
        n77 = Index Array(array=w407, index=w357) -> (element=w384:dbl)
        n78 = Index Array(array=w407, index=0) -> (element=w385:dbl)
        n79 = Index Array(array=w394, index=w357) -> (element=w387:dbl)
        n80 = Index Array(array=w394, index=0) -> (element=w386:dbl)
        n81 = local write "Ig max"(w403) -> ()
        n82 = local write "Ig min"(w402) -> ()
        n83 = local write "Is max"(w398) -> ()
        n84 = local write "Is min"(w399) -> ()
        n85 = local write "Id max"(w441) -> ()
        n86 = local write "Id min"(w404) -> ()
        n87 = local write "I vs Vg"(w434) -> ()
        n88 = Build Array (concatenate)(w397, w398) -> (w376:dbl[])
        n89 = Build Array (concatenate)(w396, w399) -> (w374:dbl[])
        n90 = local write "Is off"(w383) -> ()
        n91 = local write "Is on"(w382) -> ()
        n92 = Build Array (concatenate)(w442, w441) -> (w373:dbl[])
        n93 = Build Array (concatenate)(w429, w404) -> (w372:dbl[])
        n94 = Build Array (concatenate)(w401, w403) -> (w371:dbl[])
        n95 = Build Array (concatenate)(w400, w402) -> (w370:dbl[])
        n96 = Build Array (concatenate)(w389, w382) -> (w369:dbl[])
        n97 = Build Array (concatenate)(w388, w383) -> (w368:dbl[])
        n98 = Build Array (concatenate)(w411, w384) -> (w367:dbl[])
        n99 = Build Array (concatenate)(w412, w385) -> (w366:dbl[])
        n100 = Build Array (concatenate)(w393, w387) -> (w365:dbl[])
        n101 = Build Array (concatenate)(w392, w386) -> (w364:dbl[])
        n102 = local write "Ig off"(w386) -> ()
        n103 = local write "Ig on"(w387) -> ()
        n104 = local write "Id off"(w385) -> ()
        n105 = local write "Id on"(w384) -> ()
        n106 = call "4155C Split array.vi"("Number of VAR2 steps"=w375, "Y2 data in"=w367, "X data in"=w381, "Y1 data in"=w369, "Y3 data in"=w365, "error in (no error)"=w363) -> ("Array of clusters"=w379:cluster{"Y data in":dbl[], "X data in":dbl[]}[], "error out"=w362:errorcluster)  [unwired: 1 in]
        n107 = call "4155C Split array.vi"("Number of VAR2 steps"=w375, "Y2 data in"=w366, "X data in"=w381, "Y1 data in"=w368, "Y3 data in"=w364, "error in (no error)"=w362) -> ("Array of clusters"=w380:cluster{"Y data in":dbl[], "X data in":dbl[]}[], "error out"=w361:errorcluster)  [unwired: 1 in]
        n108 = call "4155C Split array.vi"("Number of VAR2 steps"=w375, "Y2 data in"=w373, "X data in"=w381, "Y1 data in"=w376, "Y3 data in"=w371, "error in (no error)"=w361) -> ("Array of clusters"=w433:cluster{"Y data in":dbl[], "X data in":dbl[]}[], "error out"=w360:errorcluster)  [unwired: 1 in]
        n109 = call "4155C Split array.vi"("Number of VAR2 steps"=w375, "Y2 data in"=w372, "X data in"=w381, "Y1 data in"=w374, "Y3 data in"=w370, "error in (no error)"=w360) -> ("Array of clusters"=w430:cluster{"Y data in":dbl[], "X data in":dbl[]}[], "error out"=w359:errorcluster)  [unwired: 1 in]
        n110 = Open/Create/Replace File(file path (use dialog)=w490, error in=w359, operation (0:open)=w444) -> (refnum out=w427:refnum<file>, error out=w425:errorcluster)  [unwired: 3 in, 1 out]
        n111 = call "4155C Make Big 2d array.vi"("1D Var1"=w443, "1d IS"=w406, "1d ID"=w408, "1d IG"=w405, "1d SMU4"=w448, "SMU4"=w447, "VAR2 START"=w449, "Number of VAR2 steps"=w375, "VAR2 STEP"=w450, "VAR1 Name"="Vg", "Decimal places in header"=i8 1, "VAR2 Name"="Vd") -> ("Header array"=w428:string[], "Data array"=w426:dbl[][])  [unwired: 14 in]
        n112 = local write "Imax vs time"(w433) -> ()
        n113 = local write "Imin vs time"(w430) -> ()
        n114 = local write "Ion vs time"(w379) -> ()
        n115 = local write "Ioff vs time"(w380) -> ()
        n116 = call "4155C Config Chart Colours.vi"("Numeric"=w375, "XY Graph 2"=w410) -> ()  [unwired: 6 in]
        n117 = call "4155C Config Chart Colours.vi"("Numeric"=w375, "XY Graph 2"=w409) -> ()  [unwired: 6 in]
        n118 = call "4155C Config Chart Colours.vi"("Numeric"=w375, "XY Graph 2"=w378) -> ()  [unwired: 6 in]
        n119 = call "4155C Config Chart Colours.vi"("Numeric"=w375, "XY Graph 2"=w377) -> ()  [unwired: 6 in]
        n120 = call "4155C Config Chart Colours.vi"("Numeric"=w375, "XY Graph 2"=w440) -> ()  [unwired: 6 in]
        n121 = call "4155C Write array to file.vi"("Byte Stream File Refnum"=w427, "Header"=w428, "Data Array"=w426, "error in (no error)"=w425) -> ("dup refnum"=w424:refnum<file>, "error out"=w423:errorcluster)  [unwired: 1 in]
        n122 = Close File(refnum=w424, error in=w423) -> (error out=w485:errorcluster)  [unwired: 1 out]
      }
      frame "pulsedstressV" {
        w527 = 0
        n123 = Number To Decimal String(number=w518) -> (decimal integer string=w574:string)  [unwired: 1 in]
        n124 = Delete From Array(array=w508, index=0 ("Index")) -> (deleted portion=w565:string, array with subset deleted=w564:string[])  [unwired: 1 in]
        n125 = Bundle By Name(cluster=w544, "Emergency Stop"=w577) -> (w546:T2)
        n126 = VISA Write(VISA resource name=w558, write buffer=":PAGE:CHAN:MODE SWE;" ("write buffer (\"\")"), error in (no error)=w557) -> (VISA resource name out=w555:refnum<visa-resource-name>, error out=w556:errorcluster)  [unwired: 1 out]
        n127 = Concatenate Strings(w573, "-pulsedstressV-" ("Substring"), w574, w517, ".txt" ("Substring")) -> (w576:string)
        n128 = case shown="\"d\", Default" w565 {
          tunnel: [w586 w587] -> w563
          frame "s" {
            w586 = u16 0 items=["Single", "Double"] ("sweep mode")
          }
          frame "d", Default {
            w587 = u16 1 items=["Single", "Double"] ("sweep mode")
          }
        }
        n129 = Fract/Exp String To Number(string=w564) -> (number=w559:dbl[])  [unwired: 3 in, 1 out]
        n130 = String To Path(string=w576) -> (path=w572:path)
        n131 = Index Array(array=w559, index #1=0 ("Index")) -> (element #1=w536:dbl, element #2=w535:dbl, element #3=w532:dbl, element #4=w531:dbl, element #5=w530:dbl, element #6=w534:dbl)  [unwired: 5 in]
        n132 = Bundle By Name(cluster=w533, "Pulse period"=w531, "Base voltage"=w532, "Pulse width"=w530) -> (w529:T5)
        n133 = Unbundle By Name(w529) -> ("Pulse period"=w537:dbl)
        n134 = Bundle By Name(cluster=w561, "Gate Start"=w535, "Gate Stop"=w536, "Gate Step (linear only)"=0, "Gate Compliance"=w570, "Range mode"=w551, "Range"=w550) -> (w552:T6)
        n135 = call <vilib>:"compatOverwrite.vi"("overwrite (F)"=TRUE) -> ("overwrite?"=w522:T8)
        n136 = Bundle By Name(cluster=w560, "Drain Start"=w534, "Drain Stop"=w527, "Drain Step"=w527, "Drain Compliance"=w571, "Range mode"=w549, "Range"=w548) -> (w553:T7)
        n137 = call "4155C PulsedStressV.vi"("VISA resource name in"=w555, "sweep mode"=w563, "Panel Controls"=w546, "Gate"=w552, "Drain"=w553, "Timings"=w529, "error in (no error)"=w556, "SMU4"=w545) -> ("VISA Resource Name out"=w568:refnum<visa-resource-name>, "ID"=w525:dbl[], "IG"=w523:dbl[], "Outparams"=w547:T9, "error out"=w569:errorcluster)  [unwired: 3 in]
        n138 = Unbundle By Name(w547) -> ("Number of points"=w524:i32)  [unwired: 2 out]
        n139 = for {
          N: w524 -> [_]
          tunnel: [w583] -> w526 mode=indexing
          tunnel: w537 -> [w585]
          i -> [w584]
          n140 = Multiply(x=w585, y=w584) -> (x*y=w583:dbl)
        }
        n141 = Insert Into Array(array=dbl[][] [] ("Input Array"), new element=w526) -> (w538:dbl[][])  [unwired: 2 in]
        n142 = Insert Into Array(array=w538, new element=w525) -> (w543:dbl[][])  [unwired: 2 in]
        n143 = Insert Into Array(array=w543, new element=w523) -> (w542:dbl[][])  [unwired: 2 in]
        n144 = Transpose 2D Array(2D array=w542) -> (transposed array=w541:dbl[][])
        n145 = Open/Create/Replace File(file path (use dialog)=w572, error in=w569, operation (0:open)=w522) -> (refnum out=w580:refnum<file>, error out=w581:errorcluster)  [unwired: 3 in, 1 out]
        n146 = call "4155C Write array to file.vi"("Byte Stream File Refnum"=w580, "Header"=string[] ["Time /s", "Id /A", "Ig /A"], "Data Array"=w541, "error in (no error)"=w581) -> ("dup refnum"=w578:refnum<file>, "error out"=w579:errorcluster)  [unwired: 1 in]
        n147 = Close File(refnum=w578, error in=w579) -> (error out=w567:errorcluster)  [unwired: 1 out]
      }
      frame "transfer-fpp" {
        n148 = Number To Decimal String(number=w609) -> (decimal integer string=w663:string)  [unwired: 1 in]
        n149 = Bundle By Name(cluster=w639, "Emergency Stop"=w667) -> (w675:T1)
        n150 = Delete From Array(array=w654, index=0 ("Index")) -> (deleted portion=w652:string, array with subset deleted=w651:string[])  [unwired: 1 in]
        n151 = Concatenate Strings(w662, "-transferfpp-" ("Substring"), w663, w607, ".txt" ("Substring")) -> (w665:string)
        n152 = VISA Write(VISA resource name=w631, write buffer=":PAGE:CHAN:MODE SWE;" ("write buffer (\"\")"), error in (no error)=w630) -> (VISA resource name out=w628:refnum<visa-resource-name>, error out=w629:errorcluster)  [unwired: 1 out]
        n153 = case shown="\"d\", Default" w652 {
          tunnel: [w676 w677] -> w650
          frame "s" {
            w676 = u16 0 items=["Single", "Double"] ("sweep mode")
          }
          frame "d", Default {
            w677 = u16 1 items=["Single", "Double"] ("sweep mode")
          }
        }
        n154 = Fract/Exp String To Number(string=w651) -> (number=w635:dbl[])  [unwired: 3 in, 1 out]
        n155 = String To Path(string=w665) -> (path=w661:path)
        n156 = Index Array(array=w635, index #1=0 ("Index")) -> (element #1=w649:dbl, element #2=w648:dbl, element #3=w647:dbl)  [unwired: 2 in]
        n157 = Delete From Array(array=w635, length=3 ("Length"), index=0 ("Index")) -> (array with subset deleted=w633:dbl[])  [unwired: 1 out]
        n158 = Bundle By Name(cluster=w641, "Gate Start"=w649, "Gate Stop"=w648, "Gate Step (linear only)"=w647, "Gate Compliance"=w659, "Range mode"=w624, "Range"=w623) -> (w625:T6)
        n159 = Index Array(array=w633, index #1=0 ("Index")) -> (element #1=w644:dbl, element #2=w643:dbl, element #3=w642:dbl)  [unwired: 2 in]
        n160 = call <vilib>:"compatOverwrite.vi"("overwrite (F)"=TRUE) -> ("overwrite?"=w612:T8)
        n161 = Bundle By Name(cluster=w640, "Drain Start"=w644, "Drain Stop"=w643, "Drain Step"=w642, "Drain Compliance"=w660, "Range mode"=w622, "Range"=w621) -> (w626:T7)
        n162 = call "4155C Transfer-FPP.vi"("VISA resource name in"=w628, "Gate"=w625, "Drain"=w626, "Timings"=w658, "error in (no error)"=w629, "sweep mode"=w650, "Panel Controls"=w675) -> ("VG"=w666:dbl[], "Outparams"=w620:T9, "VISA Resource Name out"=w656:refnum<visa-resource-name>, "Vprobe2"=w616:dbl[], "ID"=w615:dbl[], "IG"=w614:dbl[], "Vprobe1"=w613:dbl[], "error out"=w657:errorcluster)  [unwired: 13 in]
        n163 = Unbundle By Name(w620) -> ("V2 Step"=w619:dbl, "V2 Start"=w618:dbl, "Number of points"=w617:i32)
        n164 = Open/Create/Replace File(file path (use dialog)=w661, error in=w657, operation (0:open)=w612) -> (refnum out=w672:refnum<file>, error out=w673:errorcluster)  [unwired: 3 in, 1 out]
        n165 = call "4155C Make Big 2d array FPP.vi"("1D Var1"=w666, "1d ID"=w615, "1d Vp2"=w616, "1d IG"=w614, "1d Vp1"=w613, "VAR2 START"=w618, "Number of VAR2 steps"=w617, "VAR2 STEP"=w619, "VAR1 Name"="Vg", "Decimal places in header"=i8 1, "VAR2 Name"="Vd") -> ("Header array"=w668:string[], "Data array"=w669:dbl[][])  [unwired: 15 in]
        n166 = call "4155C Write array to file.vi"("Byte Stream File Refnum"=w672, "Header"=w668, "Data Array"=w669, "error in (no error)"=w673) -> ("dup refnum"=w670:refnum<file>, "error out"=w671:errorcluster)  [unwired: 1 in]
        n167 = Close File(refnum=w670, error in=w671) -> (error out=w655:errorcluster)  [unwired: 1 out]
      }
      frame "output" {
        n168 = Number To Decimal String(number=w707) -> (decimal integer string=w756:string)  [unwired: 1 in]
        n169 = Bundle By Name(cluster=w733, "Emergency Stop"=w758) -> (w768:T1)
        n170 = Delete From Array(array=w748, index=0 ("Index")) -> (deleted portion=w746:string, array with subset deleted=w745:string[])  [unwired: 1 in]
        n171 = Concatenate Strings(w755, w678, w756, w706, "_O.txt" ("Suffix (output)")) -> (w757:string)
        n172 = VISA Write(VISA resource name=w724, write buffer=":PAGE:CHAN:MODE SWE;" ("write buffer (\"\")"), error in (no error)=w721) -> (VISA resource name out=w723:refnum<visa-resource-name>, error out=w722:errorcluster)  [unwired: 1 out]
        n173 = case shown="\"d\", Default" w746 {
          tunnel: [w769 w770] -> w744
          frame "s" {
            w769 = u16 0 items=["Single", "Double"] ("sweep mode")
          }
          frame "d", Default {
            w770 = u16 1 items=["Single", "Double"] ("sweep mode")
          }
        }
        n174 = Fract/Exp String To Number(string=w745) -> (number=w727:dbl[])  [unwired: 3 in, 1 out]
        n175 = String To Path(string=w757) -> (path=w754:path)
        n176 = Index Array(array=w727, index #1=0 ("Index")) -> (element #1=w743:dbl, element #2=w742:dbl, element #3=w741:dbl)  [unwired: 2 in]
        n177 = Delete From Array(array=w727, length=3 ("Length"), index=0 ("Index")) -> (array with subset deleted=w726:dbl[])  [unwired: 1 out]
        n178 = control-ref of="I vs Vd"() -> (w697:refnum<vi>)
        n179 = Bundle By Name(cluster=w735, "Gate Start"=w743, "Gate Stop"=w742, "Gate Step (linear only)"=w741, "Gate Compliance"=w752, "Range mode"=w719, "Range"=w718) -> (w767:T6)
        n180 = Index Array(array=w726, index #1=0 ("Index")) -> (element #1=w738:dbl, element #2=w737:dbl, element #3=w736:dbl)  [unwired: 2 in]
        n181 = call <vilib>:"compatOverwrite.vi"("overwrite (F)"=TRUE) -> ("overwrite?"=w711:T8)
        n182 = Bundle By Name(cluster=w734, "Drain Start"=w738, "Drain Stop"=w737, "Drain Step"=w736, "Drain Compliance"=w753, "Range mode"=w717, "Range"=w720) -> (w766:T7)
        n183 = call "4155C Output.vi"("VISA resource name in"=w723, "Gate"=w767, "Drain"=w766, "Timings"=w751, "error in (no error)"=w722, "SMU4"=w713, "sweep mode"=w744, "Panel controls"=w768) -> ("VD"=w704:dbl[], "Outparams"=w715:T9, "VISA Resource Name out"=w750:refnum<visa-resource-name>, "IS"=w703:dbl[], "ID"=w702:dbl[], "IG"=w701:dbl[], "error out"=w699:errorcluster, "SMU4"=w712:dbl[])  [unwired: 12 in]
        n184 = Unbundle By Name(w715) -> ("V2 Step"=w716:dbl, "V2 Start"=w714:dbl, "Number of points"=w696:i32)
        n185 = call "4155C Split array.vi"("Number of VAR2 steps"=w696, "Y2 data in"=w702, "X data in"=w704, "Y1 data in"=w703, "Y3 data in"=w701, "error in (no error)"=w699) -> ("Array of clusters"=w700:cluster{"Y data in":dbl[], "X data in":dbl[]}[], "error out"=w698:errorcluster)  [unwired: 1 in]
        n186 = local write "I vs Vd"(w700) -> ()
        n187 = call "4155C Config Chart Colours.vi"("Numeric"=w696, "XY Graph 2"=w697) -> ()  [unwired: 6 in]
        n188 = Open/Create/Replace File(file path (use dialog)=w754, error in=w698, operation (0:open)=w711) -> (refnum out=w763:refnum<file>, error out=w764:errorcluster)  [unwired: 3 in, 1 out]
        n189 = call "4155C Make Big 2d array.vi"("1D Var1"=w704, "1d IS"=w703, "1d ID"=w702, "1d IG"=w701, "1d SMU4"=w712, "SMU4"=w713, "VAR2 START"=w714, "Number of VAR2 steps"=w696, "VAR2 STEP"=w716, "VAR1 Name"="Vd", "Decimal places in header"=i8 1, "VAR2 Name"="Vg") -> ("Header array"=w759:string[], "Data array"=w760:dbl[][])  [unwired: 14 in]
        n190 = call "4155C Write array to file.vi"("Byte Stream File Refnum"=w763, "Header"=w759, "Data Array"=w760, "error in (no error)"=w764) -> ("dup refnum"=w761:refnum<file>, "error out"=w762:errorcluster)  [unwired: 1 in]
        n191 = Close File(refnum=w761, error in=w762) -> (error out=w749:errorcluster)  [unwired: 1 out]
      }
      frame "output2" {
        # "Adjusts graph colors."
        # "Adjusts graph colors."
        # "Is off"
        # "Is on"
        # "Ion will be the middle element of the array. The calculation of the index is done only once, since Is, Id, and Ig have the same dimensions."
        # "Ig off"
        # "Ig on"
        # "Is min"
        # "Is max"
        # "Ig min"
        # "Ig max"
        # "abs(Ig)"
        # "abs(Is)"
        # "Id min"
        # "Id max"
        # "Y1: Is\nY2: Id\nY3: Ig"
        # "abs(Id)"
        # "Adjusts graph colors."
        # "Adjusts graph colors."
        # "Id off"
        # "Id on"
        # "Adjusts graph colors."
        # "Time array"
        n192 = Delete From Array(array=w900, index=0 ("Index")) -> (deleted portion=w898:string, array with subset deleted=w897:string[])  [unwired: 1 in]
        n193 = Bundle By Name(cluster=w771, "Emergency Stop"=w909) -> (w862:T1)
        n194 = Number To Decimal String(number=w856) -> (decimal integer string=w855:string)  [unwired: 1 in]
        n195 = case shown="\"d\", Default" w898 {
          tunnel: [w911 w912] -> w896
          frame "s" {
            w911 = u16 0 items=["Single", "Double"] ("sweep mode")
          }
          frame "d", Default {
            w912 = u16 1 items=["Single", "Double"] ("sweep mode")
          }
        }
        n196 = Fract/Exp String To Number(string=w897) -> (number=w882:dbl[])  [unwired: 3 in, 1 out]
        n197 = Concatenate Strings(w907, w772, w855, w853, "_O_1_C_L.txt" ("Suffix (transfer)")) -> (w908:string)
        n198 = VISA Write(VISA resource name=w878, write buffer=":PAGE:CHAN:MODE SWE;" ("write buffer (\"\")"), error in (no error)=w877) -> (VISA resource name out=w875:refnum<visa-resource-name>, error out=w876:errorcluster)  [unwired: 1 out]
        n199 = String To Path(string=w908) -> (path=w906:path)
        n200 = Index Array(array=w882, index #1=0 ("Index")) -> (element #1=w895:dbl, element #2=w894:dbl, element #3=w893:dbl)  [unwired: 2 in]
        n201 = Delete From Array(array=w882, length=3 ("Length"), index=0 ("Index")) -> (array with subset deleted=w880:dbl[])  [unwired: 1 out]
        n202 = Build Array (concatenate)(w852, w848) -> (w798:i32[])
        n203 = Bundle By Name(cluster=w887, "Gate Start"=w895, "Gate Stop"=w894, "Gate Step (linear only)"=w893, "Gate Compliance"=w904, "Range mode"=w871, "Range"=w870) -> (w872:T6)
        n204 = control-ref of="Imax vs time"() -> (w827:refnum<vi>)
        n205 = control-ref of="Imin vs time"() -> (w826:refnum<vi>)
        n206 = control-ref of="Ion vs time"() -> (w795:refnum<vi>)
        n207 = control-ref of="Ioff vs time"() -> (w794:refnum<vi>)
        n208 = control-ref of="I vs Vg"() -> (w857:refnum<vi>)
        n209 = Index Array(array=w880, index #1=0 ("Index")) -> (element #1=w890:dbl, element #2=w889:dbl, element #3=w888:dbl)  [unwired: 2 in]
        n210 = call <vilib>:"compatOverwrite.vi"("overwrite (F)"=TRUE) -> ("overwrite?"=w861:T8)
        n211 = Bundle By Name(cluster=w886, "Drain Start"=w890, "Drain Stop"=w889, "Drain Step"=w888, "Drain Compliance"=w905, "Range mode"=w869, "Range"=w868) -> (w873:T7)
        n212 = call "4155C Output.vi"("VISA resource name in"=w875, "Gate"=w872, "Drain"=w873, "Timings"=w903, "error in (no error)"=w876, "SMU4"=w863, "sweep mode"=w896, "Panel controls"=w862) -> ("VD"=w860:dbl[], "Outparams"=w867:T9, "VISA Resource Name out"=w902:refnum<visa-resource-name>, "IS"=w823:dbl[], "ID"=w825:dbl[], "IG"=w822:dbl[], "error out"=w849:errorcluster, "SMU4"=w864:dbl[])  [unwired: 12 in]
        n213 = Unbundle By Name(w867) -> ("V2 Step"=w866:dbl, "V2 Start"=w865:dbl, "Number of points"=w792:i32)
        n214 = Absolute Value(x=w823) -> (abs(x)=w808:dbl[])
        n215 = Absolute Value(x=w825) -> (abs(x)=w824:dbl[])
        n216 = Absolute Value(x=w822) -> (abs(x)=w811:dbl[])
        n217 = Array Size(array=w824) -> (size(s)=w832:i32)
        n218 = Divide(x=w832, y=2) -> (x/y=w775:dbl)
        n219 = Subtract(x=w775, y=1) -> (x-y=w774:dbl)
        n220 = Array Max & Min(array=w808) -> (max value=w815:dbl, min value=w816:dbl)  [unwired: 2 out]
        n221 = Array Max & Min(array=w824) -> (max value=w858:dbl, min value=w821:dbl)  [unwired: 2 out]
        n222 = Array Max & Min(array=w811) -> (max value=w820:dbl, min value=w819:dbl)  [unwired: 2 out]
        n223 = call "4155C Split array.vi"("Number of VAR2 steps"=w792, "Y2 data in"=w825, "X data in"=w860, "Y1 data in"=w823, "Y3 data in"=w822, "error in (no error)"=w849) -> ("Array of clusters"=w851:cluster{"Y data in":dbl[], "X data in":dbl[]}[], "error out"=w780:errorcluster)  [unwired: 1 in]
        n224 = Index Array(array=w808, index=w774) -> (element=w799:dbl)
        n225 = Index Array(array=w808, index=0) -> (element=w800:dbl)
        n226 = Index Array(array=w824, index=w774) -> (element=w801:dbl)
        n227 = Index Array(array=w824, index=0) -> (element=w802:dbl)
        n228 = Index Array(array=w811, index=w774) -> (element=w804:dbl)
        n229 = Index Array(array=w811, index=0) -> (element=w803:dbl)
        n230 = local write "Ig max"(w820) -> ()
        n231 = local write "Ig min"(w819) -> ()
        n232 = local write "Is max"(w815) -> ()
        n233 = local write "Is min"(w816) -> ()
        n234 = local write "Id max"(w858) -> ()
        n235 = local write "Id min"(w821) -> ()
        n236 = local write "I vs Vd"(w851) -> ()
        n237 = Build Array (concatenate)(w814, w815) -> (w793:dbl[])
        n238 = Build Array (concatenate)(w813, w816) -> (w791:dbl[])
        n239 = local write "Is off"(w800) -> ()
        n240 = local write "Is on"(w799) -> ()
        n241 = Build Array (concatenate)(w859, w858) -> (w790:dbl[])
        n242 = Build Array (concatenate)(w846, w821) -> (w789:dbl[])
        n243 = Build Array (concatenate)(w818, w820) -> (w788:dbl[])
        n244 = Build Array (concatenate)(w817, w819) -> (w787:dbl[])
        n245 = Build Array (concatenate)(w806, w799) -> (w786:dbl[])
        n246 = Build Array (concatenate)(w805, w800) -> (w785:dbl[])
        n247 = Build Array (concatenate)(w828, w801) -> (w784:dbl[])
        n248 = Build Array (concatenate)(w829, w802) -> (w783:dbl[])
        n249 = Build Array (concatenate)(w810, w804) -> (w782:dbl[])
        n250 = Build Array (concatenate)(w809, w803) -> (w781:dbl[])
        n251 = local write "Ig off"(w803) -> ()
        n252 = local write "Ig on"(w804) -> ()
        n253 = local write "Id off"(w802) -> ()
        n254 = local write "Id on"(w801) -> ()
        n255 = call "4155C Split array.vi"("Number of VAR2 steps"=w792, "Y2 data in"=w784, "X data in"=w798, "Y1 data in"=w786, "Y3 data in"=w782, "error in (no error)"=w780) -> ("Array of clusters"=w796:cluster{"Y data in":dbl[], "X data in":dbl[]}[], "error out"=w779:errorcluster)  [unwired: 1 in]
        n256 = call "4155C Split array.vi"("Number of VAR2 steps"=w792, "Y2 data in"=w783, "X data in"=w798, "Y1 data in"=w785, "Y3 data in"=w781, "error in (no error)"=w779) -> ("Array of clusters"=w797:cluster{"Y data in":dbl[], "X data in":dbl[]}[], "error out"=w778:errorcluster)  [unwired: 1 in]
        n257 = call "4155C Split array.vi"("Number of VAR2 steps"=w792, "Y2 data in"=w790, "X data in"=w798, "Y1 data in"=w793, "Y3 data in"=w788, "error in (no error)"=w778) -> ("Array of clusters"=w850:cluster{"Y data in":dbl[], "X data in":dbl[]}[], "error out"=w777:errorcluster)  [unwired: 1 in]
        n258 = call "4155C Split array.vi"("Number of VAR2 steps"=w792, "Y2 data in"=w789, "X data in"=w798, "Y1 data in"=w791, "Y3 data in"=w787, "error in (no error)"=w777) -> ("Array of clusters"=w847:cluster{"Y data in":dbl[], "X data in":dbl[]}[], "error out"=w776:errorcluster)  [unwired: 1 in]
        n259 = Open/Create/Replace File(file path (use dialog)=w906, error in=w776, operation (0:open)=w861) -> (refnum out=w844:refnum<file>, error out=w842:errorcluster)  [unwired: 3 in, 1 out]
        n260 = call "4155C Make Big 2d array.vi"("1D Var1"=w860, "1d IS"=w823, "1d ID"=w825, "1d IG"=w822, "1d SMU4"=w864, "SMU4"=w863, "VAR2 START"=w865, "Number of VAR2 steps"=w792, "VAR2 STEP"=w866, "VAR1 Name"="Vd", "Decimal places in header"=i8 1, "VAR2 Name"="Vg") -> ("Header array"=w845:string[], "Data array"=w843:dbl[][])  [unwired: 14 in]
        n261 = local write "Imax vs time"(w850) -> ()
        n262 = local write "Imin vs time"(w847) -> ()
        n263 = local write "Ion vs time"(w796) -> ()
        n264 = local write "Ioff vs time"(w797) -> ()
        n265 = call "4155C Config Chart Colours.vi"("Numeric"=w792, "XY Graph 2"=w827) -> ()  [unwired: 6 in]
        n266 = call "4155C Config Chart Colours.vi"("Numeric"=w792, "XY Graph 2"=w826) -> ()  [unwired: 6 in]
        n267 = call "4155C Config Chart Colours.vi"("Numeric"=w792, "XY Graph 2"=w795) -> ()  [unwired: 6 in]
        n268 = call "4155C Config Chart Colours.vi"("Numeric"=w792, "XY Graph 2"=w794) -> ()  [unwired: 6 in]
        n269 = call "4155C Config Chart Colours.vi"("Numeric"=w792, "XY Graph 2"=w857) -> ()  [unwired: 6 in]
        n270 = call "4155C Write array to file.vi"("Byte Stream File Refnum"=w844, "Header"=w845, "Data Array"=w843, "error in (no error)"=w842) -> ("dup refnum"=w841:refnum<file>, "error out"=w840:errorcluster)  [unwired: 1 in]
        n271 = Close File(refnum=w841, error in=w840) -> (error out=w901:errorcluster)  [unwired: 1 out]
      }
      frame "output-fpp" {
        n272 = Number To Decimal String(number=w933) -> (decimal integer string=w987:string)  [unwired: 1 in]
        n273 = Bundle By Name(cluster=w963, "Emergency Stop"=w990) -> (w1000:T1)
        n274 = Delete From Array(array=w978, index=0 ("Index")) -> (deleted portion=w976:string, array with subset deleted=w975:string[])  [unwired: 1 in]
        n275 = VISA Write(VISA resource name=w954, write buffer=":PAGE:CHAN:MODE SWE;" ("write buffer (\"\")"), error in (no error)=w951) -> (VISA resource name out=w953:refnum<visa-resource-name>, error out=w952:errorcluster)  [unwired: 1 out]
        n276 = Concatenate Strings(w986, "-outputfpp-" ("Substring"), w987, w932, ".txt" ("Substring")) -> (w989:string)
        n277 = case shown="\"d\", Default" w976 {
          tunnel: [w1001 w1002] -> w974
          frame "s" {
            w1001 = u16 0 items=["Single", "Double"] ("sweep mode")
          }
          frame "d", Default {
            w1002 = u16 1 items=["Single", "Double"] ("sweep mode")
          }
        }
        n278 = Fract/Exp String To Number(string=w975) -> (number=w957:dbl[])  [unwired: 3 in, 1 out]
        n279 = String To Path(string=w989) -> (path=w985:path)
        n280 = Index Array(array=w957, index #1=0 ("Index")) -> (element #1=w973:dbl, element #2=w972:dbl, element #3=w971:dbl)  [unwired: 2 in]
        n281 = Delete From Array(array=w957, length=3 ("Length"), index=0 ("Index")) -> (array with subset deleted=w956:dbl[])  [unwired: 1 out]
        n282 = Bundle By Name(cluster=w965, "Gate Start"=w973, "Gate Stop"=w972, "Gate Step (linear only)"=w971, "Gate Compliance"=w983, "Range mode"=w949, "Range"=w948) -> (w999:T6)
        n283 = Index Array(array=w956, index #1=0 ("Index")) -> (element #1=w968:dbl, element #2=w967:dbl, element #3=w966:dbl)  [unwired: 2 in]
        n284 = call <vilib>:"compatOverwrite.vi"("overwrite (F)"=TRUE) -> ("overwrite?"=w937:T8)
        n285 = Bundle By Name(cluster=w964, "Drain Start"=w968, "Drain Stop"=w967, "Drain Step"=w966, "Drain Compliance"=w984, "Range mode"=w947, "Range"=w950) -> (w998:T7)
        n286 = call "4155C Output-FPP.vi"("VISA resource name in"=w953, "Gate"=w999, "Drain"=w998, "Timings"=w982, "error in (no error)"=w952, "sweep mode"=w974, "Panel controls"=w1000) -> ("VD"=w942:dbl[], "Outparams"=w945:T9, "VISA Resource Name out"=w980:refnum<visa-resource-name>, "Vprobe2"=w941:dbl[], "ID"=w940:dbl[], "IG"=w939:dbl[], "Vprobe1"=w938:dbl[], "error out"=w981:errorcluster)  [unwired: 13 in]
        n287 = Unbundle By Name(w945) -> ("V2 Step"=w946:dbl, "V2 Start"=w944:dbl, "Number of points"=w943:i32)
        n288 = Open/Create/Replace File(file path (use dialog)=w985, error in=w981, operation (0:open)=w937) -> (refnum out=w995:refnum<file>, error out=w996:errorcluster)  [unwired: 3 in, 1 out]
        n289 = call "4155C Make Big 2d array FPP.vi"("1D Var1"=w942, "1d ID"=w940, "1d Vp2"=w941, "1d IG"=w939, "1d Vp1"=w938, "VAR2 START"=w944, "Number of VAR2 steps"=w943, "VAR2 STEP"=w946, "VAR1 Name"="Vd", "Decimal places in header"=i8 1, "VAR2 Name"="Vg") -> ("Header array"=w991:string[], "Data array"=w992:dbl[][])  [unwired: 15 in]
        n290 = call "4155C Write array to file.vi"("Byte Stream File Refnum"=w995, "Header"=w991, "Data Array"=w992, "error in (no error)"=w996) -> ("dup refnum"=w993:refnum<file>, "error out"=w994:errorcluster)  [unwired: 1 in]
        n291 = Close File(refnum=w993, error in=w994) -> (error out=w979:errorcluster)  [unwired: 1 out]
      }
      frame "itime" {
        n292 = Delete From Array(array=w1005, index=1) -> (deleted portion=w1004:string)  [unwired: 1 in, 1 out]
        n293 = Delete From Array(array=w1005, index=0 ("Index")) -> (deleted portion=w1039:string)  [unwired: 1 in, 1 out]
        n294 = Fract/Exp String To Number(string=w1004) -> (number=w1003:dbl)  [unwired: 3 in, 1 out]
        n295 = case shown="\"l\"" w1039 {
          tunnel: w1038 -> [w1044 w1046 w1050]
          tunnel: [w1043 w1045 w1049] -> w1031
          tunnel: w1003 -> [w1041 _ w1048]
          frame "s" {
            w1042 = u32 0 items=["short  ", "medium  ", "long  "] ("integration time 2")
            n296 = Bundle By Name(cluster=w1044, "integration time"=w1042, "Short/Long integration time"=w1041) -> (w1043:T5)
          }
          frame "m", Default {
            w1047 = u32 1 items=["short  ", "medium  ", "long  "] ("integration time 2")
            n297 = Bundle By Name(cluster=w1046, "integration time"=w1047) -> (w1045:T5)
          }
          frame "l" {
            w1051 = u32 2 items=["short  ", "medium  ", "long  "] ("integration time 2")
            n298 = Bundle By Name(cluster=w1050, "integration time"=w1051, "Short/Long integration time"=w1048) -> (w1049:T5)
          }
        }
      }
      frame "pulsed" {
        n299 = Delete From Array(array=w1085, index=0 ("Index")) -> (deleted portion=w1086:string, array with subset deleted=w1073:string[])  [unwired: 1 in]
        n300 = case shown="\"on\", Default" w1086 {
          tunnel: w1084 -> [w1096 w1099]
          tunnel: [w1095 w1098] -> w1077
          tunnel: w1073 -> [w1093 _]
          frame "on", Default {
            w1094 = u16 1 items=["Continuous", "Pulsed"] ("sweep method")
            n301 = Fract/Exp String To Number(string=w1093) -> (number=w1091:dbl[])  [unwired: 3 in, 1 out]
            n302 = Index Array(array=w1091, index #1=0 ("Index")) -> (element #1=w1090:dbl, element #2=w1089:dbl, element #3=w1088:dbl)  [unwired: 2 in]
            n303 = Bundle By Name(cluster=w1096, "sweep method"=w1094, "Pulse period"=w1090, "Base voltage"=w1089, "Pulse width"=w1088) -> (w1095:T5)
          }
          frame "off" {
            w1097 = u16 0 items=["Continuous", "Pulsed"] ("sweep method")
            n304 = Bundle By Name(cluster=w1099, "sweep method"=w1097) -> (w1098:T5)
          }
        }
      }
      frame "gaterangemode" {
        n305 = Delete From Array(array=w1131, index=0 ("Index")) -> (deleted portion=w1132:string)  [unwired: 1 in, 1 out]
        n306 = case shown="\"f\"" w1132 {
          tunnel: [w1134 w1135 w1136] -> w1121
          frame "a", Default {
            w1134 = u16 0 items=["Auto", "Limited", "Fixed"] ("Gate Range\nmode 2")
          }
          frame "f" {
            w1135 = u16 2 items=["Auto", "Limited", "Fixed"] ("Gate Range\nmode 2")
          }
          frame "l" {
            w1136 = u16 1 items=["Auto", "Limited", "Fixed"] ("Gate Range\nmode 2")
          }
        }
      }
      frame "gaterange" {
        (unwired) u8 11 items=["10fA  ", "100fA  ", "1nA  ", "10nA", "100nA", "1uA", "10uA", "100uA", "1mA", "10mA", "100mA", "1A"] ("Gate Range 2")
        n307 = Delete From Array(array=w1175, index=0 ("Index")) -> (deleted portion=w1165:string)  [unwired: 1 in, 1 out]
        n308 = Scan Value(string=w1165, format string="") -> (value=w1163:dbl)  [unwired: 1 in, 1 out]
        n309 = Logarithm Base 10(1:w1163) -> (0:w1162:dbl)
        n310 = Round To Nearest(number=w1162) -> (nearest integer value=w1161:dbl)
        n311 = Add(x=w1161, y=11.0) -> (x+y=w1159:dbl)
        n312 = To Unsigned Byte Integer(number=w1159) -> (unsigned 8bit integer=w1158:u8)
      }
      frame "drainrange" {
        (unwired) u8 11 items=["10fA  ", "100fA  ", "1nA  ", "10nA", "100nA", "1uA", "10uA", "100uA", "1mA", "10mA", "100mA", "1A"] ("Gate Range 2")
        n313 = Delete From Array(array=w1215, index=0 ("Index")) -> (deleted portion=w1206:string)  [unwired: 1 in, 1 out]
        n314 = Scan Value(string=w1206, format string="") -> (value=w1204:dbl)  [unwired: 1 in, 1 out]
        n315 = Logarithm Base 10(1:w1204) -> (0:w1203:dbl)
        n316 = Round To Nearest(number=w1203) -> (nearest integer value=w1202:dbl)
        n317 = Add(x=w1202, y=11.0) -> (x+y=w1200:dbl)
        n318 = To Unsigned Byte Integer(number=w1200) -> (unsigned 8bit integer=w1199:u8)
      }
      frame "drainrangemode" {
        n319 = Delete From Array(array=w1248, index=0 ("Index")) -> (deleted portion=w1249:string)  [unwired: 1 in, 1 out]
        n320 = case shown="\"f\"" w1249 {
          tunnel: [w1251 w1252 w1253] -> w1238
          frame "a", Default {
            w1251 = u16 0 items=["Auto", "Limited", "Fixed"] ("Gate Range\nmode 2")
          }
          frame "f" {
            w1252 = u16 2 items=["Auto", "Limited", "Fixed"] ("Gate Range\nmode 2")
          }
          frame "l" {
            w1253 = u16 1 items=["Auto", "Limited", "Fixed"] ("Gate Range\nmode 2")
          }
        }
      }
      frame "Error", Default {
      }
      frame "logfile" {
        n321 = Number To Decimal String(number=w1306) -> (decimal integer string=w1341:string)  [unwired: 1 in]
        n322 = Concatenate Strings(w1340, "logfile" ("Substring"), w1341, w1304, ".txt" ("Substring")) -> (w1338:string)
        n323 = String To Path(string=w1338) -> (path=w1311:path)
        n324 = Unbundle(w1337) -> ("integration time"=w1336:u32, "Short/Long integration time"=w1335:dbl, "hold time (sec)"=w1334:dbl, "delay time (sec)"=w1333:dbl, "Step Time (0 disables)"=w1332:dbl, "sweep method"=w1331:u16, "Pulse period"=w1330:dbl, "Base voltage"=w1329:dbl, "Pulse width"=w1328:dbl)
        n325 = Build Array(w1336, w1335, w1334, w1333, w1332, w1331, w1330, w1329, w1328, w1322, w1323, w1324, w1325, w1326, w1327) -> (w1315:dbl[])
        n326 = Insert Into Array(array=dbl[][] [] ("Input Array"), new element=w1315) -> (w1314:dbl[][])  [unwired: 2 in]
        n327 = call <vilib>:"compatOverwrite.vi"("overwrite (F)"=TRUE) -> ("overwrite?"=w1309:T8)
        n328 = Open/Create/Replace File(file path (use dialog)=w1311, error in=w1313, operation (0:open)=w1309) -> (refnum out=w1319:refnum<file>, error out=w1318:errorcluster)  [unwired: 3 in, 1 out]
        n329 = call "4155C Write array to file.vi"("Byte Stream File Refnum"=w1319, "Header"=string[] ["Int Time", "Short/Long Itime", "Hold time", "Delay time", "Step time", "Sweep method", "Pulse period", "Base Voltage", "Pulse width", "Drain compliance", "Gate compliance", "Gate range mode", "Gate range", "S/D range mode", "S/D range"], "Data Array"=w1314, "error in (no error)"=w1318) -> ("dup refnum"=w1321:refnum<file>, "error out"=w1320:errorcluster)  [unwired: 1 in]
        n330 = Close File(refnum=w1321, error in=w1320) -> (error out=w1312:errorcluster)  [unwired: 1 out]
      }
      frame "sample" {
        n331 = Number To Decimal String(number=w1364) -> (decimal integer string=w1412:string)  [unwired: 1 in]
        n332 = Fract/Exp String To Number(string=w1409) -> (number=w1370:dbl[])  [unwired: 3 in, 1 out]
        n333 = Concatenate Strings(w1387, "-sample-" ("Substring"), w1412, w1362, ".txt" ("Substring")) -> (w1410:string)
        n334 = Index Array(array=w1370, index=0 ("Index")) -> (element=w1407:dbl)
        n335 = String To Path(string=w1410) -> (path=w1391:path)
        n336 = Index Array(array=w1370, index=2 ("Index")) -> (element=w1403:dbl)
        n337 = Index Array(array=w1370, index=3 ("Index")) -> (element=w1372:dbl)
        n338 = Index Array(array=w1370, index=4 ("Index")) -> (element=w1369:dbl)
        n339 = call "4155C Config Sampling Measurements.vi"("Sampling interval"=w1369, "Sample time"=w1372, "Display on/off"=TRUE, "Timings"=w1378, "Num Points"=w1403, "error in (no error)"=w1414, "Drain Compliance"=w1413, "Gate Compliance"=w1388, "VISA session"=w1415) -> ("error out"=w1416:errorcluster, "dup VISA resource name"=w1417:refnum<visa-resource-name>)  [unwired: 1 in]
        n340 = Index Array(array=w1370, index=1 ("Index")) -> (element=w1404:dbl)
        n341 = call "4155C Take Sample.vi"("Emergency Stop"=w1384, "error in (no error)"=w1416, "Vd"=w1404, "Vg"=w1407, "VISA resource name in"=w1417) -> ("error out"=w1382:errorcluster, "Id"=w1419:dbl[], "Ig"=w1393:dbl[], "VISA Resource Name out"=w1380:refnum<visa-resource-name>, "Is"=w1418:dbl[], "Time"=w1397:dbl[])  [unwired: 1 in]
        n342 = Insert Into Array(array=dbl[][] [] ("Input Array"), new element=w1397) -> (w1396:dbl[][])  [unwired: 2 in]
        n343 = Insert Into Array(array=w1396, new element=w1393) -> (w1395:dbl[][])  [unwired: 2 in]
        n344 = Insert Into Array(array=w1395, new element=w1419) -> (w1394:dbl[][])  [unwired: 2 in]
        n345 = VISA Write(VISA resource name=w1380, write buffer=":DISP ON" ("write buffer (\"\")"), error in (no error)=w1382) -> (VISA resource name out=w1379:refnum<visa-resource-name>, error out=w1381:errorcluster)  [unwired: 1 out]
        n346 = Insert Into Array(array=w1394, new element=w1418) -> (w1386:dbl[][])  [unwired: 2 in]
        n347 = Transpose 2D Array(2D array=w1386) -> (transposed array=w1385:dbl[][])
        n348 = call <vilib>:"compatOverwrite.vi"("overwrite (F)"=TRUE) -> ("overwrite?"=w1367:T8)
        n349 = Open/Create/Replace File(file path (use dialog)=w1391, error in=w1381, operation (0:open)=w1367) -> (refnum out=w1400:refnum<file>, error out=w1399:errorcluster)  [unwired: 3 in, 1 out]
        n350 = call "4155C Write array to file.vi"("Byte Stream File Refnum"=w1400, "Header"=string[] ["Time /s", "Ig /A", "Id /A", "Is /A"], "Data Array"=w1385, "error in (no error)"=w1399) -> ("dup refnum"=w1402:refnum<file>, "error out"=w1401:errorcluster)  [unwired: 1 in]
        n351 = Close File(refnum=w1402, error in=w1401) -> (error out=w1389:errorcluster)  [unwired: 1 out]
      }
      frame "samplei" {
        n352 = Number To Decimal String(number=w1441) -> (decimal integer string=w1492:string)  [unwired: 1 in]
        n353 = Concatenate Strings(w1471, "-samplei-" ("Substring"), w1492, w1440, ".txt" ("Substring")) -> (w1490:string)
        n354 = Fract/Exp String To Number(string=w1489) -> (number=w1456:dbl[])  [unwired: 3 in, 1 out]
        n355 = String To Path(string=w1490) -> (path=w1474:path)
        n356 = Index Array(array=w1456, index=4 ("Index")) -> (element=w1450:dbl)
        n357 = Index Array(array=w1456, index=3 ("Index")) -> (element=w1451:dbl)
        n358 = Index Array(array=w1456, index=1 ("Index")) -> (element=w1453:dbl)
        n359 = Index Array(array=w1456, index=0 ("Index")) -> (element=w1454:dbl)
        n360 = Index Array(array=w1456, index=2 ("Index")) -> (element=w1452:dbl)
        n361 = call "4155C Config SamplingI Measurements.vi"("Sample time"=w1452, "Display on/off"=TRUE, "Timings"=w1463, "Num Points"=w1453, "error in (no error)"=w1494, "Sampling interval"=w1451, "VISA session"=w1495) -> ("error out"=w1496:errorcluster, "dup VISA resource name"=w1497:refnum<visa-resource-name>)  [unwired: 3 in]
        n362 = call "4155C Take SampleI.vi"("Emergency Stop"=w1468, "error in (no error)"=w1496, "Idg 2"=w1454, "Vdg compliance 2"=w1450, "VISA resource name in"=w1497) -> ("error out"=w1466:errorcluster, "Idg"=w1499:dbl[], "Vdg"=w1476:dbl[], "VISA Resource Name out"=w1464:refnum<visa-resource-name>, "Is"=w1498:dbl[], "Time"=w1480:dbl[])  [unwired: 1 in]
        n363 = Insert Into Array(array=dbl[][] [] ("Input Array"), new element=w1480) -> (w1479:dbl[][])  [unwired: 2 in]
        n364 = Insert Into Array(array=w1479, new element=w1476) -> (w1478:dbl[][])  [unwired: 2 in]
        n365 = Insert Into Array(array=w1478, new element=w1499) -> (w1477:dbl[][])  [unwired: 2 in]
        n366 = VISA Write(VISA resource name=w1464, write buffer=":DISP ON" ("write buffer (\"\")"), error in (no error)=w1466) -> (VISA resource name out=w1449:refnum<visa-resource-name>, error out=w1465:errorcluster)  [unwired: 1 out]
        n367 = Insert Into Array(array=w1477, new element=w1498) -> (w1470:dbl[][])  [unwired: 2 in]
        n368 = call <vilib>:"compatOverwrite.vi"("overwrite (F)"=TRUE) -> ("overwrite?"=w1444:T8)
        n369 = Open/Create/Replace File(file path (use dialog)=w1474, error in=w1465, operation (0:open)=w1444) -> (refnum out=w1483:refnum<file>, error out=w1482:errorcluster)  [unwired: 3 in, 1 out]
        n370 = Transpose 2D Array(2D array=w1470) -> (transposed array=w1469:dbl[][])
        n371 = call "4155C Write array to file.vi"("Byte Stream File Refnum"=w1483, "Header"=string[] ["Time /s", "Vdg /V", "Idg /A", "Is /A"], "Data Array"=w1469, "error in (no error)"=w1482) -> ("dup refnum"=w1485:refnum<file>, "error out"=w1484:errorcluster)  [unwired: 1 in]
        n372 = Close File(refnum=w1485, error in=w1484) -> (error out=w1447:errorcluster)  [unwired: 1 out]
        n373 = VISA Write(VISA resource name=w1449, write buffer=";:PAGE:SCON:STAN OFF;:PAGE:CHAN:VSU2:DIS;" ("write buffer (\"\")"), error in (no error)=w1447) -> (VISA resource name out=w1445:refnum<visa-resource-name>, error out=w1446:errorcluster)  [unwired: 1 out]
      }
      frame "#" {
        n374 = VISA Write(VISA resource name=w1525, write buffer=":DISP ON" ("write buffer (\"\")"), error in (no error)=w1524) -> (VISA resource name out=w1523:refnum<visa-resource-name>, error out=w1522:errorcluster)  [unwired: 1 out]
      }
      frame "stressV" {
        n375 = Number To Decimal String(number=w1554) -> (decimal integer string=w1595:string)  [unwired: 1 in]
        n376 = Concatenate Strings(w1579, "-stressV-" ("Substring"), w1595, w1553, ".txt" ("Substring")) -> (w1593:string)
        n377 = Fract/Exp String To Number(string=w1592) -> (number=w1565:dbl[])  [unwired: 3 in, 1 out]
        n378 = String To Path(string=w1593) -> (path=w1583:path)
        n379 = Index Array(array=w1565, index=3 ("Index")) -> (element=w1562:dbl)
        n380 = Index Array(array=w1565, index=1 ("Index")) -> (element=w1560:dbl)
        n381 = Index Array(array=w1565, index=0 ("Index")) -> (element=w1559:dbl)
        n382 = Index Array(array=w1565, index=4 ("Index")) -> (element=w1564:dbl)
        n383 = Index Array(array=w1565, index=2 ("Index")) -> (element=w1561:dbl)
        n384 = call "4155C Config V Stress.vi"("VISA session"=w1598, "ID compliance"=w1562, "VD"=w1560, "VG"=w1559, "IG compliance"=w1561, "error in (no error)"=w1597, "Display on/off"=TRUE) -> ("dup VISA resource name"=w1600:refnum<visa-resource-name>, "error out"=w1599:errorcluster)
        n385 = call "4155C Apply Stress.vi"("error in (no error)"=w1599, "Duration"=w1564, "Emergency Stop"=w1578, "VISA resource name in"=w1600) -> ("error out"=w1576:errorcluster, "VISA Resource Name out"=w1574:refnum<visa-resource-name>)
        n386 = VISA Write(VISA resource name=w1574, write buffer=":DISP ON" ("write buffer (\"\")"), error in (no error)=w1576) -> (VISA resource name out=w1573:refnum<visa-resource-name>, error out=w1575:errorcluster)  [unwired: 1 out]
        n387 = call <vilib>:"compatOverwrite.vi"("overwrite (F)"=TRUE) -> ("overwrite?"=w1558:T8)
        n388 = Open/Create/Replace File(file path (use dialog)=w1583, error in=w1575, operation (0:open)=w1558) -> (refnum out=w1586:refnum<file>, error out=w1585:errorcluster)  [unwired: 3 in, 1 out]
        n389 = call "4155C Write array to file.vi"("Byte Stream File Refnum"=w1586, "Header"=string[] ["V stress completed successfully", ""], "error in (no error)"=w1585) -> ("dup refnum"=w1588:refnum<file>, "error out"=w1587:errorcluster)  [unwired: 2 in]
        n390 = Close File(refnum=w1588, error in=w1587) -> (error out=w1581:errorcluster)  [unwired: 1 out]
      }
      frame "stressI" {
        n391 = Number To Decimal String(number=w1621) -> (decimal integer string=w1658:string)  [unwired: 1 in]
        n392 = Concatenate Strings(w1642, "-stressI-" ("Substring"), w1658, w1620, ".txt" ("Substring")) -> (w1656:string)
        n393 = Fract/Exp String To Number(string=w1655) -> (number=w1630:dbl[])  [unwired: 3 in, 1 out]
        n394 = Index Array(array=w1630, index=1 ("Index")) -> (element=w1626:dbl)
        n395 = Index Array(array=w1630, index=0 ("Index")) -> (element=w1627:dbl)
        n396 = call "4155C Config I Stress.vi"("VISA session"=w1661, "IDG"=w1627, "VDG compliance"=w1626, "error in (no error)"=w1660, "Display on/off"=TRUE) -> ("dup VISA resource name"=w1663:refnum<visa-resource-name>, "error out"=w1662:errorcluster)
        n397 = Index Array(array=w1630, index=2 ("Index")) -> (element=w1628:dbl)
        n398 = String To Path(string=w1656) -> (path=w1646:path)
        n399 = call "4155C Apply Stress.vi"("error in (no error)"=w1662, "Duration"=w1628, "Emergency Stop"=w1641, "VISA resource name in"=w1663) -> ("error out"=w1639:errorcluster, "VISA Resource Name out"=w1637:refnum<visa-resource-name>)
        n400 = VISA Write(VISA resource name=w1637, write buffer=":DISP ON" ("write buffer (\"\")"), error in (no error)=w1639) -> (VISA resource name out=w1636:refnum<visa-resource-name>, error out=w1638:errorcluster)  [unwired: 1 out]
        n401 = call <vilib>:"compatOverwrite.vi"("overwrite (F)"=TRUE) -> ("overwrite?"=w1625:T8)
        n402 = Open/Create/Replace File(file path (use dialog)=w1646, error in=w1638, operation (0:open)=w1625) -> (refnum out=w1649:refnum<file>, error out=w1648:errorcluster)  [unwired: 3 in, 1 out]
        n403 = call "4155C Write array to file.vi"("Byte Stream File Refnum"=w1649, "Header"=string[] ["I stress completed successfully", ""], "error in (no error)"=w1648) -> ("dup refnum"=w1651:refnum<file>, "error out"=w1650:errorcluster)  [unwired: 2 in]
        n404 = Close File(refnum=w1651, error in=w1650) -> (error out=w1644:errorcluster)  [unwired: 1 out]
      }
      frame "vsu2pulse" {
        n405 = Number To Decimal String(number=w1684) -> (decimal integer string=w1719:string)  [unwired: 1 in]
        n406 = Concatenate Strings(w1704, "-vsu2-" ("Substring"), w1719, w1683, ".txt" ("Substring")) -> (w1717:string)
        n407 = Fract/Exp String To Number(string=w1716) -> (number=w1692:dbl[])  [unwired: 3 in, 1 out]
        n408 = String To Path(string=w1717) -> (path=w1708:path)
        n409 = Index Array(array=w1692, index=1 ("Index")) -> (element=w1691:dbl)
        n410 = Index Array(array=w1692, index=0 ("Index")) -> (element=w1689:dbl)
        n411 = call "4155C Config VSU2 Stress.vi"("error in (no error)"=w1721, "VSU2"=w1689, "Display on/off"=TRUE, "VISA session"=w1722) -> ("error out"=w1723:errorcluster, "dup VISA resource name"=w1724:refnum<visa-resource-name>)
        n412 = call "4155C Apply Stress.vi"("error in (no error)"=w1723, "Duration"=w1691, "Emergency Stop"=w1703, "VISA resource name in"=w1724) -> ("error out"=w1701:errorcluster, "VISA Resource Name out"=w1699:refnum<visa-resource-name>)
        n413 = VISA Write(VISA resource name=w1699, write buffer=":DISP ON" ("write buffer (\"\")"), error in (no error)=w1701) -> (VISA resource name out=w1698:refnum<visa-resource-name>, error out=w1700:errorcluster)  [unwired: 1 out]
        n414 = call <vilib>:"compatOverwrite.vi"("overwrite (F)"=TRUE) -> ("overwrite?"=w1688:T8)
        n415 = Open/Create/Replace File(file path (use dialog)=w1708, error in=w1700, operation (0:open)=w1688) -> (refnum out=w1711:refnum<file>, error out=w1710:errorcluster)  [unwired: 3 in, 1 out]
        n416 = call "4155C Write array to file.vi"("Byte Stream File Refnum"=w1711, "Header"=string[] ["VSU2 pulse completed successfully", ""], "error in (no error)"=w1710) -> ("dup refnum"=w1713:refnum<file>, "error out"=w1712:errorcluster)  [unwired: 2 in]
        n417 = Close File(refnum=w1713, error in=w1712) -> (error out=w1706:errorcluster)  [unwired: 1 out]
      }
      frame "sample-fpp" {
        w1756 = string[] ["Time /s", "Id VgVd /A", "Ig VgVd /A", "Vp1 VgVd /V", "Vp2 VgVd /V"] ("Header")
        w1760 = "%d" ("format string")
        n418 = Number To Decimal String(number=w1745) -> (decimal integer string=w1808:string)  [unwired: 1 in]
        n419 = Fract/Exp String To Number(string=w1805) -> (number=w1793:dbl[])  [unwired: 3 in, 1 out]
        n420 = Concatenate Strings(w1799, "-samplefpp-" ("Substring"), w1808, w1744, ".txt" ("Substring")) -> (w1806:string)
        n421 = String To Path(string=w1806) -> (path=w1768:path)
        n422 = Index Array(array=w1793, index=0 ("Index")) -> (element=w1754:dbl)
        n423 = Index Array(array=w1793, index=1 ("Index")) -> (element=w1753:dbl)
        n424 = Index Array(array=w1793, index=2 ("Index")) -> (element=w1801:dbl)
        n425 = Index Array(array=w1793, index=3 ("Index")) -> (element=w1791:dbl)
        n426 = call "4155C Config Sampling Measurements FPP.vi"("VISA session"=w1811, "Num Points"=w1801, "Vg"=w1754, "Display on/off"=TRUE, "Gate Compliance"=w1800, "Drain Compliance"=w1809, "Standby"="Standby", "error in (no error)"=w1810, "Timings"=w1798, "Vd"=w1753, "Sample time"=w1791) -> ("dup VISA resource name"=w1770:refnum<visa-resource-name>, "error out"=w1769:errorcluster)  [unwired: 3 in]
        n427 = Number To Decimal String(number=w1754) -> (decimal integer string=w1780:string)  [unwired: 1 in]
        n428 = call "4155C Take Sample FPP.vi"("VISA resource name in"=w1770, "error in (no error)"=w1769, "Emergency Stop"=w1771) -> ("Time"=w1775:dbl[], "Vp1"=w1785:dbl[], "VISA Resource Name out"=w1751:refnum<visa-resource-name>, "Ig"=w1773:dbl[], "Id"=w1774:dbl[], "Vp2"=w1783:dbl[], "error out"=w1772:errorcluster)  [unwired: 10 in]
        n429 = Insert Into Array(array=dbl[][] [] ("Input Array"), new element=w1775) -> (w1789:dbl[][])  [unwired: 2 in]
        n430 = Number To Decimal String(number=w1753) -> (decimal integer string=w1778:string)  [unwired: 1 in]
        n431 = Insert Into Array(array=w1789, new element=w1774) -> (w1788:dbl[][])  [unwired: 2 in]
        n432 = Concatenate Strings("(Vg = " ("Substring"), w1780, "V, Vd = " ("Substring"), w1778, "V)" ("Substring")) -> (w1776:string)
        n433 = Insert Into Array(array=w1788, new element=w1773) -> (w1787:dbl[][])  [unwired: 2 in]
        n434 = Insert Into Array(array=w1787, new element=w1785) -> (w1784:dbl[][])  [unwired: 2 in]
        n435 = Insert Into Array(array=w1784, new element=w1783) -> (w1752:dbl[][])  [unwired: 2 in]
        n436 = Transpose 2D Array(2D array=w1752) -> (transposed array=w1782:dbl[][])
        n437 = call <vilib>:"compatOverwrite.vi"("overwrite (F)"=TRUE) -> ("overwrite?"=w1749:T8)
        n438 = Open/Create/Replace File(file path (use dialog)=w1768, error in=w1772, operation (0:open)=w1749) -> (refnum out=w1765:refnum<file>, error out=w1766:errorcluster)  [unwired: 3 in, 1 out]
        n439 = Array To Spreadsheet String(array=w1756, 3:w1760) -> (spreadsheet string=w1762:string)  [unwired: 1 in]
        n440 = Search and Replace String(replace all?=TRUE ("replace all? (F)"), input string=w1762, search string="VgVd", replace string=w1776) -> (result string=w1758:string)  [unwired: 4 in, 3 out]
        n441 = Spreadsheet String To Array(format string=w1760, spreadsheet string=w1758, array type (2D Dbl)=w1756) -> (array=w1757:string[])  [unwired: 1 in]
        n442 = call "4155C Write array to file.vi"("Byte Stream File Refnum"=w1765, "Header"=w1757, "Data Array"=w1782, "error in (no error)"=w1766) -> ("dup refnum"=w1763:refnum<file>, "error out"=w1764:errorcluster)  [unwired: 1 in]
        n443 = Close File(refnum=w1763, error in=w1764) -> (error out=w1750:errorcluster)  [unwired: 1 out]
      }
      frame "resample-fpp" {
        w1845 = string[] ["Time /s", "Id VgVd /A", "Ig VgVd /A", "Vp1 VgVd /V", "Vp2 VgVd /V"] ("Header")
        w1849 = "%d" ("format string")
        n444 = Number To Decimal String(number=w1831) -> (decimal integer string=w1889:string)  [unwired: 1 in]
        n445 = Fract/Exp String To Number(string=w1886) -> (number=w1838:dbl[])  [unwired: 3 in, 1 out]
        n446 = Concatenate Strings(w1882, "-resamplefpp-" ("Substring"), w1889, w1832, ".txt" ("Substring")) -> (w1887:string)
        n447 = String To Path(string=w1887) -> (path=w1857:path)
        n448 = Index Array(array=w1838, index=0 ("Index")) -> (element=w1844:dbl)
        n449 = Index Array(array=w1838, index=1 ("Index")) -> (element=w1843:dbl)
        n450 = Number To Decimal String(number=w1844) -> (decimal integer string=w1867:string)  [unwired: 1 in]
        n451 = call "4155C Take Sample FPP.vi"("VISA resource name in"=w1840, "error in (no error)"=w1839, "Emergency Stop"=w1858) -> ("Time"=w1862:dbl[], "Vp1"=w1872:dbl[], "VISA Resource Name out"=w1842:refnum<visa-resource-name>, "Ig"=w1860:dbl[], "Id"=w1861:dbl[], "Vp2"=w1870:dbl[], "error out"=w1859:errorcluster)  [unwired: 10 in]
        n452 = Insert Into Array(array=dbl[][] [] ("Input Array"), new element=w1862) -> (w1876:dbl[][])  [unwired: 2 in]
        n453 = Number To Decimal String(number=w1843) -> (decimal integer string=w1865:string)  [unwired: 1 in]
        n454 = Insert Into Array(array=w1876, new element=w1861) -> (w1875:dbl[][])  [unwired: 2 in]
        n455 = Concatenate Strings("(Vg = " ("Substring"), w1867, "V, Vd = " ("Substring"), w1865, "V)" ("Substring")) -> (w1863:string)
        n456 = Insert Into Array(array=w1875, new element=w1860) -> (w1874:dbl[][])  [unwired: 2 in]
        n457 = Insert Into Array(array=w1874, new element=w1872) -> (w1871:dbl[][])  [unwired: 2 in]
        n458 = Insert Into Array(array=w1871, new element=w1870) -> (w1837:dbl[][])  [unwired: 2 in]
        n459 = call <vilib>:"compatOverwrite.vi"("overwrite (F)"=TRUE) -> ("overwrite?"=w1836:T8)
        n460 = Open/Create/Replace File(file path (use dialog)=w1857, error in=w1859, operation (0:open)=w1836) -> (refnum out=w1854:refnum<file>, error out=w1855:errorcluster)  [unwired: 3 in, 1 out]
        n461 = Array To Spreadsheet String(array=w1845, 3:w1849) -> (spreadsheet string=w1851:string)  [unwired: 1 in]
        n462 = Transpose 2D Array(2D array=w1837) -> (transposed array=w1869:dbl[][])
        n463 = Search and Replace String(replace all?=TRUE ("replace all? (F)"), input string=w1851, search string="VgVd", replace string=w1863) -> (result string=w1847:string)  [unwired: 4 in, 3 out]
        n464 = Spreadsheet String To Array(format string=w1849, spreadsheet string=w1847, array type (2D Dbl)=w1845) -> (array=w1846:string[])  [unwired: 1 in]
        n465 = call "4155C Write array to file.vi"("Byte Stream File Refnum"=w1854, "Header"=w1846, "Data Array"=w1869, "error in (no error)"=w1855) -> ("dup refnum"=w1852:refnum<file>, "error out"=w1853:errorcluster)  [unwired: 1 in]
        n466 = Close File(refnum=w1852, error in=w1853) -> (error out=w1841:errorcluster)  [unwired: 1 out]
      }
      frame "serial" {
        n467 = local read "Termination char\n(0xA = '\\n' = LF)\n(0xD = '\\r' = CR)"() -> (w1917:u8)
        n468 = local read "Enable Termination\nChar (T)"() -> (w1918:bool)
        n469 = Index Array(array=w1925, index=0 ("Index")) -> (element=w1924:string)
        n470 = local read "parity"() -> (w1908:u16)
        n471 = local read "Delay before read (ms)"() -> (w1919:u32)
        n472 = local read "byte count"() -> (w1916:u32)
        n473 = local read "Timeout (ms)"() -> (w1915:u32)
        n474 = local read "VISA resource name"() -> (w1912:refnum<visa-resource-name>)
        n475 = local read "baud rate"() -> (w1911:u32)
        n476 = local read "Serial End Mode for Reads"() -> (w1910:u16)
        n477 = local read "data bits"() -> (w1909:u16)
        n478 = local read "stop bits"() -> (w1914:u16)
        n479 = local read "flow control"() -> (w1913:u16)
        n480 = call "Serial write and read v0.5.vi"("Delay before read (ms)"=w1919, "Termination char\n(0xA = '\\n' = LF)\n(0xD = '\\r' = CR)"=w1917, "Enable Termination\nChar (T)"=w1918, "parity"=w1908, "stop bits"=w1914, "string to write"=w1924, "flow control"=w1913, "byte count"=w1916, "Serial Settings:Serial End Mode for Reads"=w1910, "Timeout (ms)"=w1915, "error in (no error)"=w1930, "VISA resource name"=w1912, "baud rate"=w1911, "data bits"=w1909) -> ("Serial port output"=w1920:string, "error out"=w1929:errorcluster)
        n481 = Build Array (concatenate)(w1920, w1921) -> (w1922:string[])
      }
      frame "pump" {
        # "Time array for valve position"
        # "Time array for absolute plunger position"
        # "Valve position"
        # "Absolute plunger position"
        # "Remove \"_\""
        # "Check if hard stop is pressed."
        # "Check if halt is pressed."
        # "Check if pump is idle. Else halt."
        n482 = Index Array(array=w1995, index=0 ("Index")) -> (element=w1972:string)
        n483 = case shown="\"No error\", Default" w1970 {
          tunnel: w1972 -> [w2031 _ w2033 w2034 w2035 w2036 _ _ w2039 w2040 _]
          tunnel: [w2031 "/1H" w2033 w2034 w2035 w2036 "/1H" "/1H" w2039 w2040 "/1H"] -> w1971
          frame "No error", Default {
          }
          frame "Initialization" {
          }
          frame "Invalid command" {
          }
          frame "Invalid operand" {
          }
          frame "Device not initialized" {
          }
          frame "Internal failure" {
          }
          frame "Plunger overload" {
          }
          frame "Valve overload" {
          }
          frame "Plunger move not allowed" {
          }
          frame "A/D converter failure" {
          }
          frame "Command overflow" {
          }
        }
        n484 = local read "Hard stop pump"() -> (w1974:bool)
        n485 = local read "Halt pump"() -> (w1977:bool)
        n486 = local read "Serial End Mode for Reads"() -> (w1983:u16)
        n487 = local read "flow control"() -> (w1986:u16)
        n488 = local read "stop bits"() -> (w1987:u16)
        n489 = local read "parity"() -> (w1981:u16)
        n490 = local read "Delay before read (ms)"() -> (w1992:u32)
        n491 = local read "byte count"() -> (w1989:u32)
        n492 = local read "Timeout (ms)"() -> (w1988:u32)
        n493 = local read "VISA resource name"() -> (w1985:refnum<visa-resource-name>)
        n494 = local read "baud rate"() -> (w1984:u32)
        n495 = local read "Enable Termination\nChar (T)"() -> (w1991:bool)
        n496 = local read "Termination char\n(0xA = '\\n' = LF)\n(0xD = '\\r' = CR)"() -> (w1990:u8)
        n497 = case shown="True" w1977 {
          tunnel: [w2045 "/1H"] -> w1976
          tunnel: w1971 -> [w2045 _]
          frame False {
          }
          frame True {
            n498 = local write "Halt pump"(FALSE) -> ()
          }
        }
        n499 = case shown="True" w1974 {
          tunnel: [w2042 "/1T"] -> w1975
          tunnel: w1976 -> [w2042 _]
          frame False {
          }
          frame True {
            n500 = local write "Hard stop pump"(FALSE) -> ()
          }
        }
        n501 = local read "data bits"() -> (w1982:u16)
        n502 = String Subset(string=w1966, offset (0)=1) -> (substring=w1964:string)  [unwired: 1 in]
        n503 = call "SPM Pump v0.6.vi"("Termination char\n(0xA = '\\n' = LF)\n(0xD = '\\r' = CR)"=w1990, "Enable Termination\nChar (T)"=w1991, "Timeout (ms)"=w1988, "Serial Settings:Serial End Mode for Reads"=w1983, "byte count"=w1989, "Delay before read (ms)"=w1992, "Time <input>"=w1969, "error in (no error)"=w2000, "Serial port input"=w1975, "VISA resource name"=w1985, "parity"=w1981, "baud rate"=w1984, "stop bits"=w1987, "data bits"=w1982, "flow control"=w1986, "Time units <input>"=w1964) -> ("Input command"=w1963:string, "Serial port data"=w1953:string[], "Pump status"=w1959:string, "Valve position"=w1961:i32, "Absolute plunger position"=w1973:i32, "Serial port"=w1968:string, "error out"=w1999:errorcluster)  [unwired: 1 in, 4 out]
        n504 = case shown="\"?6\"" w1963 {
          tunnel: [w2012 w2020 w2026] -> w1980
          tunnel: w1979 -> [w2012 w2019 w2026]
          tunnel: w1973 -> [_ w2018 _]
          tunnel: w1960 -> [w2011 w2017 w2027]
          tunnel: [w2011 w2017 w2029] -> w1962
          tunnel: w1961 -> [_ _ w2028]
          tunnel: w1958 -> [_ w2016 w2024]
          tunnel: w1957 -> [w2010 w2015 w2025]
          tunnel: [w2010 w2014 w2025] -> w1956
          tunnel: [w2009 w2013 w2023] -> w1955
          tunnel: w1954 -> [w2009 w2013 w2022]
          frame "Q", Default {
          }
          frame "?" {
            n505 = Build Array (concatenate)(w2019, w2018) -> (w2020:i32[])
            n506 = Build Array (concatenate)(w2015, w2016) -> (w2014:i32[])
            n507 = call "4155C Split array.vi"("X data in"=w2014, "Y1 data in"=w2020) -> ("Array of clusters"=w2021:cluster{"Y data in":dbl[], "X data in":dbl[]}[])  [unwired: 5 in, 1 out]
            n508 = local write "Absolute plunger position vs time"(w2021) -> ()
          }
          frame "?6" {
            n509 = Build Array (concatenate)(w2027, w2028) -> (w2029:i32[])
            n510 = Build Array (concatenate)(w2022, w2024) -> (w2023:i32[])
            n511 = call "4155C Split array.vi"("X data in"=w2023, "Y1 data in"=w2029) -> ("Array of clusters"=w2030:cluster{"Y data in":dbl[], "X data in":dbl[]}[])  [unwired: 5 in, 1 out]
            n512 = local write "Valve position vs time"(w2030) -> ()
          }
        }
        n513 = Build Array (concatenate)(w1951, w1953) -> (w1952:string[][])
        n514 = Build Array (concatenate)(w1967, w1968) -> (w1993:string[])
      }
      frame "filename" {
        n515 = Index Array(array=w2049, index=0 ("Index")) -> (element=w2048:string)
      }
    }
    n516 = Build Array(w143, w72, w82, w81, w80, w79, w78, w77, w76, w75, w74, w73, w71) -> (w182:dbl[][])
    n517 = Transpose 2D Array(2D array=w182) -> (transposed array=w181:dbl[][])
    n518 = Concatenate Strings(w123, w66, "Imax_Imin_Ion_Ioff_vs_time.txt" ("Suffix (Imax,Imin,Ion,Ioff)")) -> (w192:string)
    n519 = Build Array(w104, "Is max (A)" ("VAR2 Name"), "Is min (A)" ("VAR2 Name"), "Id max (A)" ("VAR2 Name"), "Id min (A)" ("VAR2 Name"), "Ig max (A)" ("VAR2 Name"), "Ig min (A)" ("VAR2 Name"), "Is on (A)" ("VAR2 Name"), "Is off (A)" ("VAR2 Name"), "Id on (A)" ("VAR2 Name"), "Id off (A)" ("VAR2 Name"), "Ig on (A)" ("VAR2 Name"), "Ig off (A)" ("VAR2 Name")) -> (w187:string[])
    n520 = Array To Spreadsheet String(array=w181, 3:"%e" ("format string")) -> (spreadsheet string=w185:string)  [unwired: 1 in]
    n521 = Array To Spreadsheet String(array=w187, 3:"" ("format string")) -> (spreadsheet string=w186:string)  [unwired: 1 in]
    n522 = String To Path(string=w192) -> (path=w191:path)
    n523 = Build Array(w186, w185) -> (w184:string[])
    n524 = Write to Text File(file (use dialog)=w191, text=w184, error in=w139) -> (refnum out=w193:refnum<file>, error out=w183:errorcluster)  [unwired: 1 in, 1 out]
    n525 = Close File(refnum=w193, error in=w183) -> (error out=w122:errorcluster)  [unwired: 1 out]
    n526 = Build Array(w118, w144) -> (w149:i32[][])
    n527 = Build Array(w104, "Absolute plunger position" ("VAR2 Name")) -> (w152:string[])
    n528 = Transpose 2D Array(2D array=w149) -> (transposed array=w142:i32[][])
    n529 = Array To Spreadsheet String(array=w152, 3:"" ("format string")) -> (spreadsheet string=w151:string)  [unwired: 1 in]
    n530 = Array To Spreadsheet String(array=w142, 3:"%e" ("format string")) -> (spreadsheet string=w148:string)  [unwired: 1 in]
    n531 = Build Array(w151, w148) -> (w154:string[])
    n532 = Concatenate Strings(w123, w66, "plunger_vs_time.txt" ("Suffix (plunger)")) -> (w146:string)
    n533 = String To Path(string=w146) -> (path=w145:path)
    n534 = Write to Text File(file (use dialog)=w145, text=w154, error in=w122) -> (refnum out=w147:refnum<file>, error out=w156:errorcluster)  [unwired: 1 in, 1 out]
    n535 = Close File(refnum=w147, error in=w156) -> (error out=w121:errorcluster)  [unwired: 1 out]
    n536 = Concatenate Strings(w123, w66, "serial_port_output.txt" ("Suffix (serial port log)")) -> (w162:string)
    n537 = String To Path(string=w162) -> (path=w161:path)
    n538 = Build Array(w104, "Serial port input" ("VAR2 Name"), "Pump status" ("VAR2 Name"), "Serial port output: ") -> (w108:string[])
    n539 = Array To Spreadsheet String(array=w114, 3:"" ("format string")) -> (spreadsheet string=w105:string)  [unwired: 1 in]
    n540 = Array To Spreadsheet String(array=w108, 3:"" ("format string")) -> (spreadsheet string=w106:string)  [unwired: 1 in]
    n541 = Build Array(w106, w105) -> (w107:string[])
    n542 = Array To Spreadsheet String(array=w113, 3:"" ("format string")) -> (spreadsheet string=w167:string)  [unwired: 1 in]
    n543 = Write to Text File(file (use dialog)=w161, text=w107, error in=w121) -> (refnum out=w163:refnum<file>, error out=w164:errorcluster)  [unwired: 1 in, 1 out]
    n544 = Close File(refnum=w163, error in=w164) -> (error out=w120:errorcluster)  [unwired: 1 out]
    n545 = local write "Serial port data"(w167) -> ()
    n546 = Build Array(w117, w125) -> (w131:i32[][])
    n547 = Build Array(w104, "Valve port" ("VAR2 Name")) -> (w134:string[])
    n548 = Transpose 2D Array(2D array=w131) -> (transposed array=w126:i32[][])
    n549 = Array To Spreadsheet String(array=w134, 3:"" ("format string")) -> (spreadsheet string=w133:string)  [unwired: 1 in]
    n550 = Array To Spreadsheet String(array=w126, 3:"%e" ("format string")) -> (spreadsheet string=w130:string)  [unwired: 1 in]
    n551 = Build Array(w133, w130) -> (w136:string[])
    n552 = Concatenate Strings(w123, w66, "valve_port_vs_time.txt" ("Suffix (valve)")) -> (w128:string)
    n553 = String To Path(string=w128) -> (path=w127:path)
    n554 = Write to Text File(file (use dialog)=w127, text=w136, error in=w120) -> (refnum out=w129:refnum<file>, error out=w138:errorcluster)  [unwired: 1 in, 1 out]
    n555 = Close File(refnum=w129, error in=w138) -> (error out=w119:errorcluster)  [unwired: 1 out]
  }
  "error out" <- w28
  "Timings Indicator" <- w10
  "Is max" <- w8
  "Id max" <- w8
  "Ig max" <- w8
  "Imax vs time" <- w4
  "I vs Vg" <- w4
  "Imin vs time" <- w4
  "I vs Vd" <- w4
  "Serial port data" <- "" ("Serial port data")
  "Valve position vs time" <- cluster{"Y data in":dbl[], "X data in":dbl[]}[] [] ("Valve position vs time")
  "Is min" <- w7
  "Id min" <- w7
  "Ig min" <- w7
  "Ion vs time" <- w4
  "Ioff vs time" <- w4
  "Is on" <- w6
  "Id on" <- w6
  "Ig on" <- w6
  "Is off" <- w5
  "Id off" <- w5
  "Ig off" <- w5
